vi "MC_8_21_12a_PD.vi"() -> ()   [LabVIEW 2011]
uses:
  <vilib>/Utility/file.llb/Read From Spreadsheet File (string).vi
  <vilib>/Utility/inputDevices.llb/keyboardAcquire.vi
  <vilib>/Utility/file.llb/Write To Spreadsheet File (DBL).vi
  <vilib>/Utility/file.llb/Write To Spreadsheet File (string).vi
  <vilib>/regexp/Match Regular Expression.xnode
panel:
  in  "Treatment Concentration (mM):":dbl=nan
  in  "Surface Treatment:":string="NaN"
  in  "# Drops*:":dbl=inf
  in  "Solution Temp (C):":dbl=nan
  in  "Relative Humidity (%):":dbl=nan
  in  "Room Temp (F):":dbl=nan
  in  "Time (s):":dbl=nan
  in  "RPM:":dbl=nan
  in  "Wait Time (s):":dbl=nan
  in  "Sample #:":dbl=1.0
  in  "Fabricator:":string="NaN"
  in  "Ramp (s):":dbl=3.0
  out "X Axis Display Type":string
  out "Opj X Axis":string
  in  "Room Temp":dbl=294.0
  out "No Image 2":path=path "\\\\acad1\\physics/Jurchescu-group/JW-PD/Image Not Found.png"
  out "Save1 Array":string[][](array[string])
  out "Lin Vd":dbl
  out "Lin-Vg Array-Used":dbl[](array[numeric])
  out "Lin Id-Used":dbl[](array[numeric])
  out "Rec: Comments":string
  out "Folder Index":dbl caption="Length"
  out "Current \nRecord":string[](array[string])
  out "Transformer \nHeaders":string[](array[string])
  out "Current Device ID":string
  out "Column":string
  out "Row":string
  out "Rec: Concentration":dbl
  out "Rec: Solvent":string
  out "Rec: Method":string
  in  "?":T1(tab)
  in  "Transport File":path
  out "Transport Folder":path
  out "Rec: Material":string
  out "Accel (RPM/s):":dbl
  in  "Transfer File":path
  out "Transfer Folder":path
  in  "Image Folder":path
  out "Image File":path=path "D:/UserData/Desktop/Jeremy/WFU/Research/Programs/VI mods/Image Not Found.png"
  in  "Manual Comments":bool
  in  "Comments:":string
  out "Calc: On/Off":dbl caption="On/Off-Sat" format="%#.2e"
  out "Calc: Off I-Sat":dbl caption="Off I-Sat" format="%#.2e"
  in  "Manuel-Dielectric":bool
  in  "Manuel-Length":bool
  out "Calc: VT-Lin":dbl
  out "New: VT-Lin":dbl
  out "Rec: VT-Lin":dbl caption="VT-Lin" format="%#_3g"
  out "Calc: Trap Density-STS":dbl format="%#.2e"
  out "New: Trap Density-STS":dbl format="%#.2e"
  out "Rec: Trap Density-STS":dbl caption="N-Sat (STS)" format="%#.2e"
  out "Calc: Trap Density-VT":dbl format="%#.2e"
  out "New: Trap Density-VT":dbl format="%#.2e"
  out "Rec: Trap Density-VT":dbl caption="N-Sat (VT)" format="%#.2e"
  out "Calc: Mobility-Lin":dbl format="%#.2e"
  out "New: Mobility-Lin":dbl format="%#_4e"
  out "Rec: Mobility-Lin":dbl caption="Mobility-Lin" format="%#_3e"
  out "Calc: Mobility-Sat":dbl format="%#.2e"
  out "Rec: Length":dbl caption="Length" format="%#_3g"
  out "Rec: Width":dbl caption="Width" format="%#_4g"
  out "Rec: Dielectric (d)":dbl caption="Dielectric (d)" format="%#_3g"
  in  "Cancel Button":bool
  in  "Up Button":bool
  in  "Down Button":bool
  out "Data Name:":string
  in  "Save Changes?":bool
  in  "New: Dielectric":dbl
  in  "New: Length":dbl
  in  "New: Width":dbl
  out "New: Mobility-Sat":dbl format="%#.2e"
  in  "Blank Button":bool
  in  "Zoom":i16(slide)=-3 scale=-5.0..5.0
  out "Image Out 2":T2(plugin-control)
  out "Image Out":T2(plugin-control)
  in  "Magnification":u16(ring) items=["5x", "10x", "20x", "50x", "80x"]
  out "Total Width":dbl
  out "Distances":dbl[](array[numeric])
  in  "Undo Button":bool
  in  "Remove Button":bool
  out "Rec: Mobility-Sat":dbl caption="Mobility-Sat" format="%#.2e"
  in  "Export":bool
  out "Calc: VT-Sat":dbl format="%#.2g"
  out "New: VT-Sat":dbl format="%#.2g"
  in  "Manual-Width":bool caption="Manual"
  out "Calc: STS":dbl format="%#.2g"
  out "New: STS":dbl format="%#.2g"
  out "Rec: VT-Sat":dbl caption="VT-Sat" format="%#.2g"
  out "Rec: STS":dbl caption="STS-Sat" format="%#.2g"
  out "Rec: On/Off":dbl caption="On/Off-Sat" format="%#.2e"
  in  "Save Changes? 2":bool
  in  "Save Changes? 3":bool
  out "Rec: Temp":dbl caption="Sample Temp" format="%.1f"
  in  "New: Temp":dbl format="%.1f"
  out "Rec: Off I-Sat":dbl caption="Off I-Sat" format="%#.2e"
  in  "Independant Variable":string(combo)="Length (um):"
  in  "Transfer Plots":enum32{"Linear", "Saturation"}(tab)=enum."Saturation"
  out "XY Graph-Lin":cluster{dbl[], dbl[]}[](graph)
  in  "Slide":dbl(slide) step=1.0 scale=-22.0..89.0 scale format="%#_1p"
  out "XY Graph":cluster{dbl[], dbl[]}[](graph)
  in  "Previous Button":bool
  in  "Next Button":bool
  in  "NumPts":dbl=5.0
  in  "Log Plots":enum32{"Linear", "Saturation"}(tab)=enum."Saturation"
  in  "Slide 2":dbl(slide) step=1.0 scale=-1.0..82.0 scale format="%#_1p"
  out "XY Graph 2":cluster{dbl[], dbl[]}[](graph)
  in  "Previous Button 2":bool
  in  "Next Button 2":bool
  in  "NumPts 2":dbl=5.0 caption="NumPts"
  in  "Manual-Temp":bool caption="Manual"
  out "Date Created":string caption="Fabricated"
  out "Date Recorded":string="Date Recorded" caption="Measured"
  out "Image Name":string
  out "Index":string
  in  "Origin Project File":path=path "\\\\acad1\\physics/Jurchescu-group/JW-PD/Group Library/Origin Project Files/DeviceData_8_10_12a_JW.opj"
  in  "No Image File":path=path "\\\\acad1\\physics/Jurchescu-group/JW-PD/Mega Awesome/Image Not Found.png"
  out "String":string
  out "Index 2":dbl
  out "Sat Id-Log-Used":dbl[](array[numeric])
  out "Vg Array-Log-Used":dbl[](array[numeric])
  out "ROI Descriptor out":T3 {"Contours"."Type" items=["No Selection", "Point", "Line", "Rectangle", "Oval", "Polygon", "Freehand Region", "Annulus", "Unused2", "Unused3", "Broken Line", "Freehand Line", "Rotated Rectangle"]}
  out "ROI Descriptor":T3 {"Contours"."Type" items=["No Selection", "Point", "Line", "Rectangle", "Oval", "Polygon", "Freehand Region", "Annulus", "Unused2", "Unused3", "Broken Line", "Freehand Line", "Rotated Rectangle"]}
  out "Numeric 3":dbl
  out "Array 6":dbl[][](array[numeric])
  out "Cluster":T4
  out "Array 5":dbl[](array[numeric])
  out "Array 4":dbl[](array[numeric])
  out "Array 3":dbl[](array[numeric])
  out "Numeric 2":dbl
  out "Numeric":dbl
  out "Sat Id-Used":dbl[](array[numeric])
  out "Sat Vg Array-Used":dbl[](array[numeric])
  out "MobVi Index":dbl
  in  "Row Start":dbl=20.0
  # "Sample Properties"
  # "*     Inf = Full coverage\n   NaN = Unknown or Not Applicable"
  # "Data Locations"
  # "Transport Location"
  # "Transfer Location"
  # "Image Location"
  # "Recorded"
  # "Calculated"
  # "Re-Calculated"
  # "Manual"
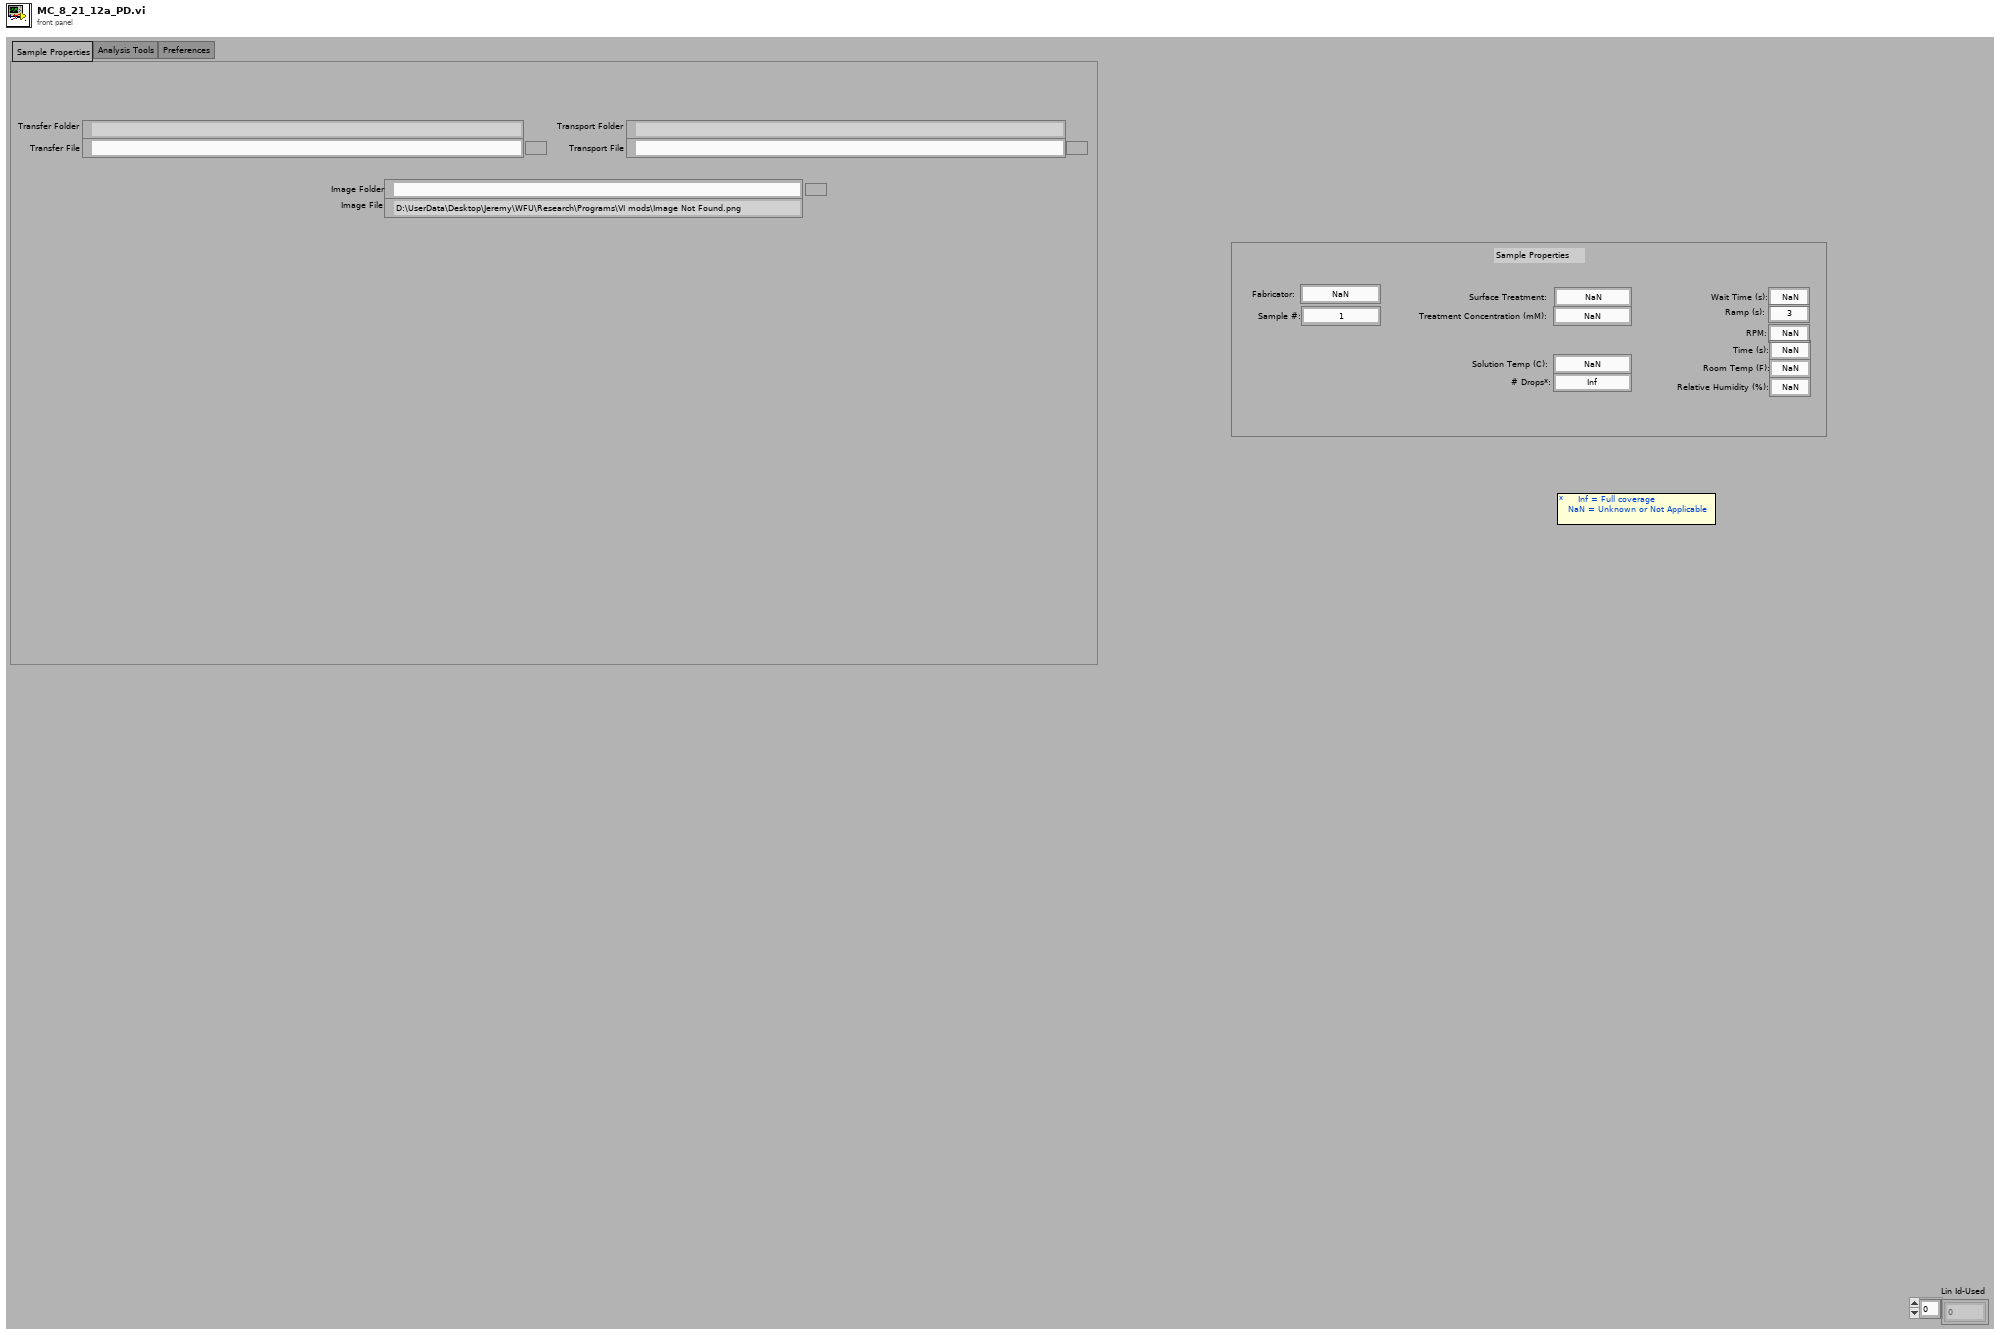
[diagram p1: front panel]
types:
  T1 = enum32{"Sample Properties", "Analysis Tools", "Preferences", "Current Database"}
  T2 = typedef "IMAQ Image.ctl" = refnum<image>
  T3 = typedef "ROI Descriptor" = cluster{"Global Rectangle":i32[], "Contours":cluster{"ID":enum32{"External", "Internal"}, "Type":u32, "Coordinates":i32[]}[]}
  T4 = cluster{"Numeric":dbl, "Numeric 2":dbl, "Numeric 3":dbl, "Numeric 4":dbl}
  T5 = cluster{"Mobility-Sat":dbl, "Moblitity-Lin":dbl, "On/Off":dbl, "Off Current":dbl, "Vt-Sat":dbl, "STS":dbl, "Trap Density-VT":dbl, "Trap Density-STS":dbl}
  T6 = cluster{"Date Recorded":string, "Index":string, "Length":dbl, "Width":dbl, "Sample Temp":dbl}
  T7 = cluster{"Date Created":string, "Material":string, "Solvent":string, "Concentration":dbl, "Method":string, "Dielectric (nm)":dbl, "Treatment":string, "Comments":string}
  T8 = cluster{"Mobility-Sat":dbl, "Vt-Sat":dbl, "Mobility-Lin":dbl, "Vt-Lin":dbl, "Off I-Sat":dbl, "On/Off I-Sat":dbl}
  T9 = cluster{"[0]":cluster{dbl[], dbl[]}, "[1]":cluster{dbl[], dbl[]}, "[2]":cluster{dbl[], dbl[]}, "[3]":cluster{dbl[], dbl[]}, "[4]":cluster{dbl[], dbl[]}, "[5]":cluster{dbl[], dbl[]}, "[6]":cluster{dbl[], dbl[]}, "[7]":cluster{dbl[], dbl[]}, "[8]":cluster{dbl[], dbl[]}}
  T10 = cluster{"Global Rectangle":i32[], "Contours":cluster{"Contour Type":u32, "ROI Type":u32, "Points":i32[]}[]}
  T11 = typedef "LVBoundsTypeDef.ctl" = cluster{"Width":u32, "Height":u32}
  T12 = enum16{"0", "1", "2", "3", "4", "5", "6", "7", "8", "9", "A", "B", "C", "D", "E", "F", "G", "H", "I", "J", "K", "L", "M", "N", "O", "P", "Q", "R", "S", "T", "U", "V", "W", "X", "Y", "Z", "F1", "F2", "F3", "F4", "F5", "F6", "F7", "F8", "F9", "F10", "F11", "F12", "F13", "F14", "F15", "ADD", "BACK", "BACKSLASH", "CAPITAL", "COMMA", "DECIMAL", "DELETE", "DIVIDE", "DOWN", "END", "EQUALS", "ESCAPE", "GRAVE (`)", "HOME", "INSERT", "LBRACKET", "LCONTROL", "LEFT", "L ALT", "LSHIFT", "LWIN", "MINUS", "MULTIPLY", "NEXT", "NUMLOCK", "NUMPAD_0", "NUMPAD_1", "NUMPAD_2", "NUMPAD_3", "NUMPAD_4", "NUMPAD_5", "NUMPAD_6", "NUMPAD_7", "NUMPAD_8", "NUMPAD_9", "PAUSE", "PERIOD", "PRIOR (PG UP)", "RBRACKET", "RCONTROL", "RETURN", "RIGHT", "R ALT", "RSHIFT", "RWIN", "SCROLL", "SEMICOLON", "SLASH", "SPACE", "SUBTRACT", "TAB", "UP", "ENTER (num pad)", "' (quote)"}[]
  T13 = enum16{"0", "1", "2", "3", "4", "5", "6", "7", "8", "9", "A", "B", "C", "D", "E", "F", "G", "H", "I", "J", "K", "L", "M", "N", "O", "P", "Q", "R", "S", "T", "U", "V", "W", "X", "Y", "Z", "F1", "F2", "F3", "F4", "F5", "F6", "F7", "F8", "F9", "F10", "F11", "F12", "F13", "F14", "F15", "ADD", "BACK", "BACKSLASH", "CAPITAL", "COMMA", "DECIMAL", "DELETE", "DIVIDE", "DOWN", "END", "EQUALS", "ESCAPE", "GRAVE (`)", "HOME", "INSERT", "LBRACKET", "LCONTROL", "LEFT", "L ALT", "LSHIFT", "LWIN", "MINUS", "MULTIPLY", "NEXT", "NUMLOCK", "NUMPAD_0", "NUMPAD_1", "NUMPAD_2", "NUMPAD_3", "NUMPAD_4", "NUMPAD_5", "NUMPAD_6", "NUMPAD_7", "NUMPAD_8", "NUMPAD_9", "PAUSE", "PERIOD", "PRIOR (PG UP)", "RBRACKET", "RCONTROL", "RETURN", "RIGHT", "R ALT", "RSHIFT", "RWIN", "SCROLL", "SEMICOLON", "SLASH", "SPACE", "SUBTRACT", "TAB", "UP", "ENTER (num pad)", "' (quote)"}
  T14 = cluster{"Contour Type":u32, "ROI Type":u32, "Points":i32[]}[]
  T15 = cluster{i32[], cluster{"Contour Type":u32, "ROI Type":u32, "Points":i32[]}[]}
  T16 = cluster{"Independant  Variable Indicator":string, "Parameter String Indicator":string}
  T17 = cluster{string, sgl, bool, bool, bool, bool, bool, bool, i32}
  T18 = cluster{i32, cluster{string, sgl, bool, bool, bool, bool, bool, bool, i32}, i32, i32}
  T19 = cluster{"Contour Type":u32, "ROI Type":u32, "Points":i32[]}
  T20 = cluster{"Points[0]":i32, "Points[1]":i32, "Points[2]":i32, "Points[3]":i32, "Points[4]":i32, "Points[5]":i32, "Points[6]":i32, "Points[7]":i32, "Points[8]":i32}
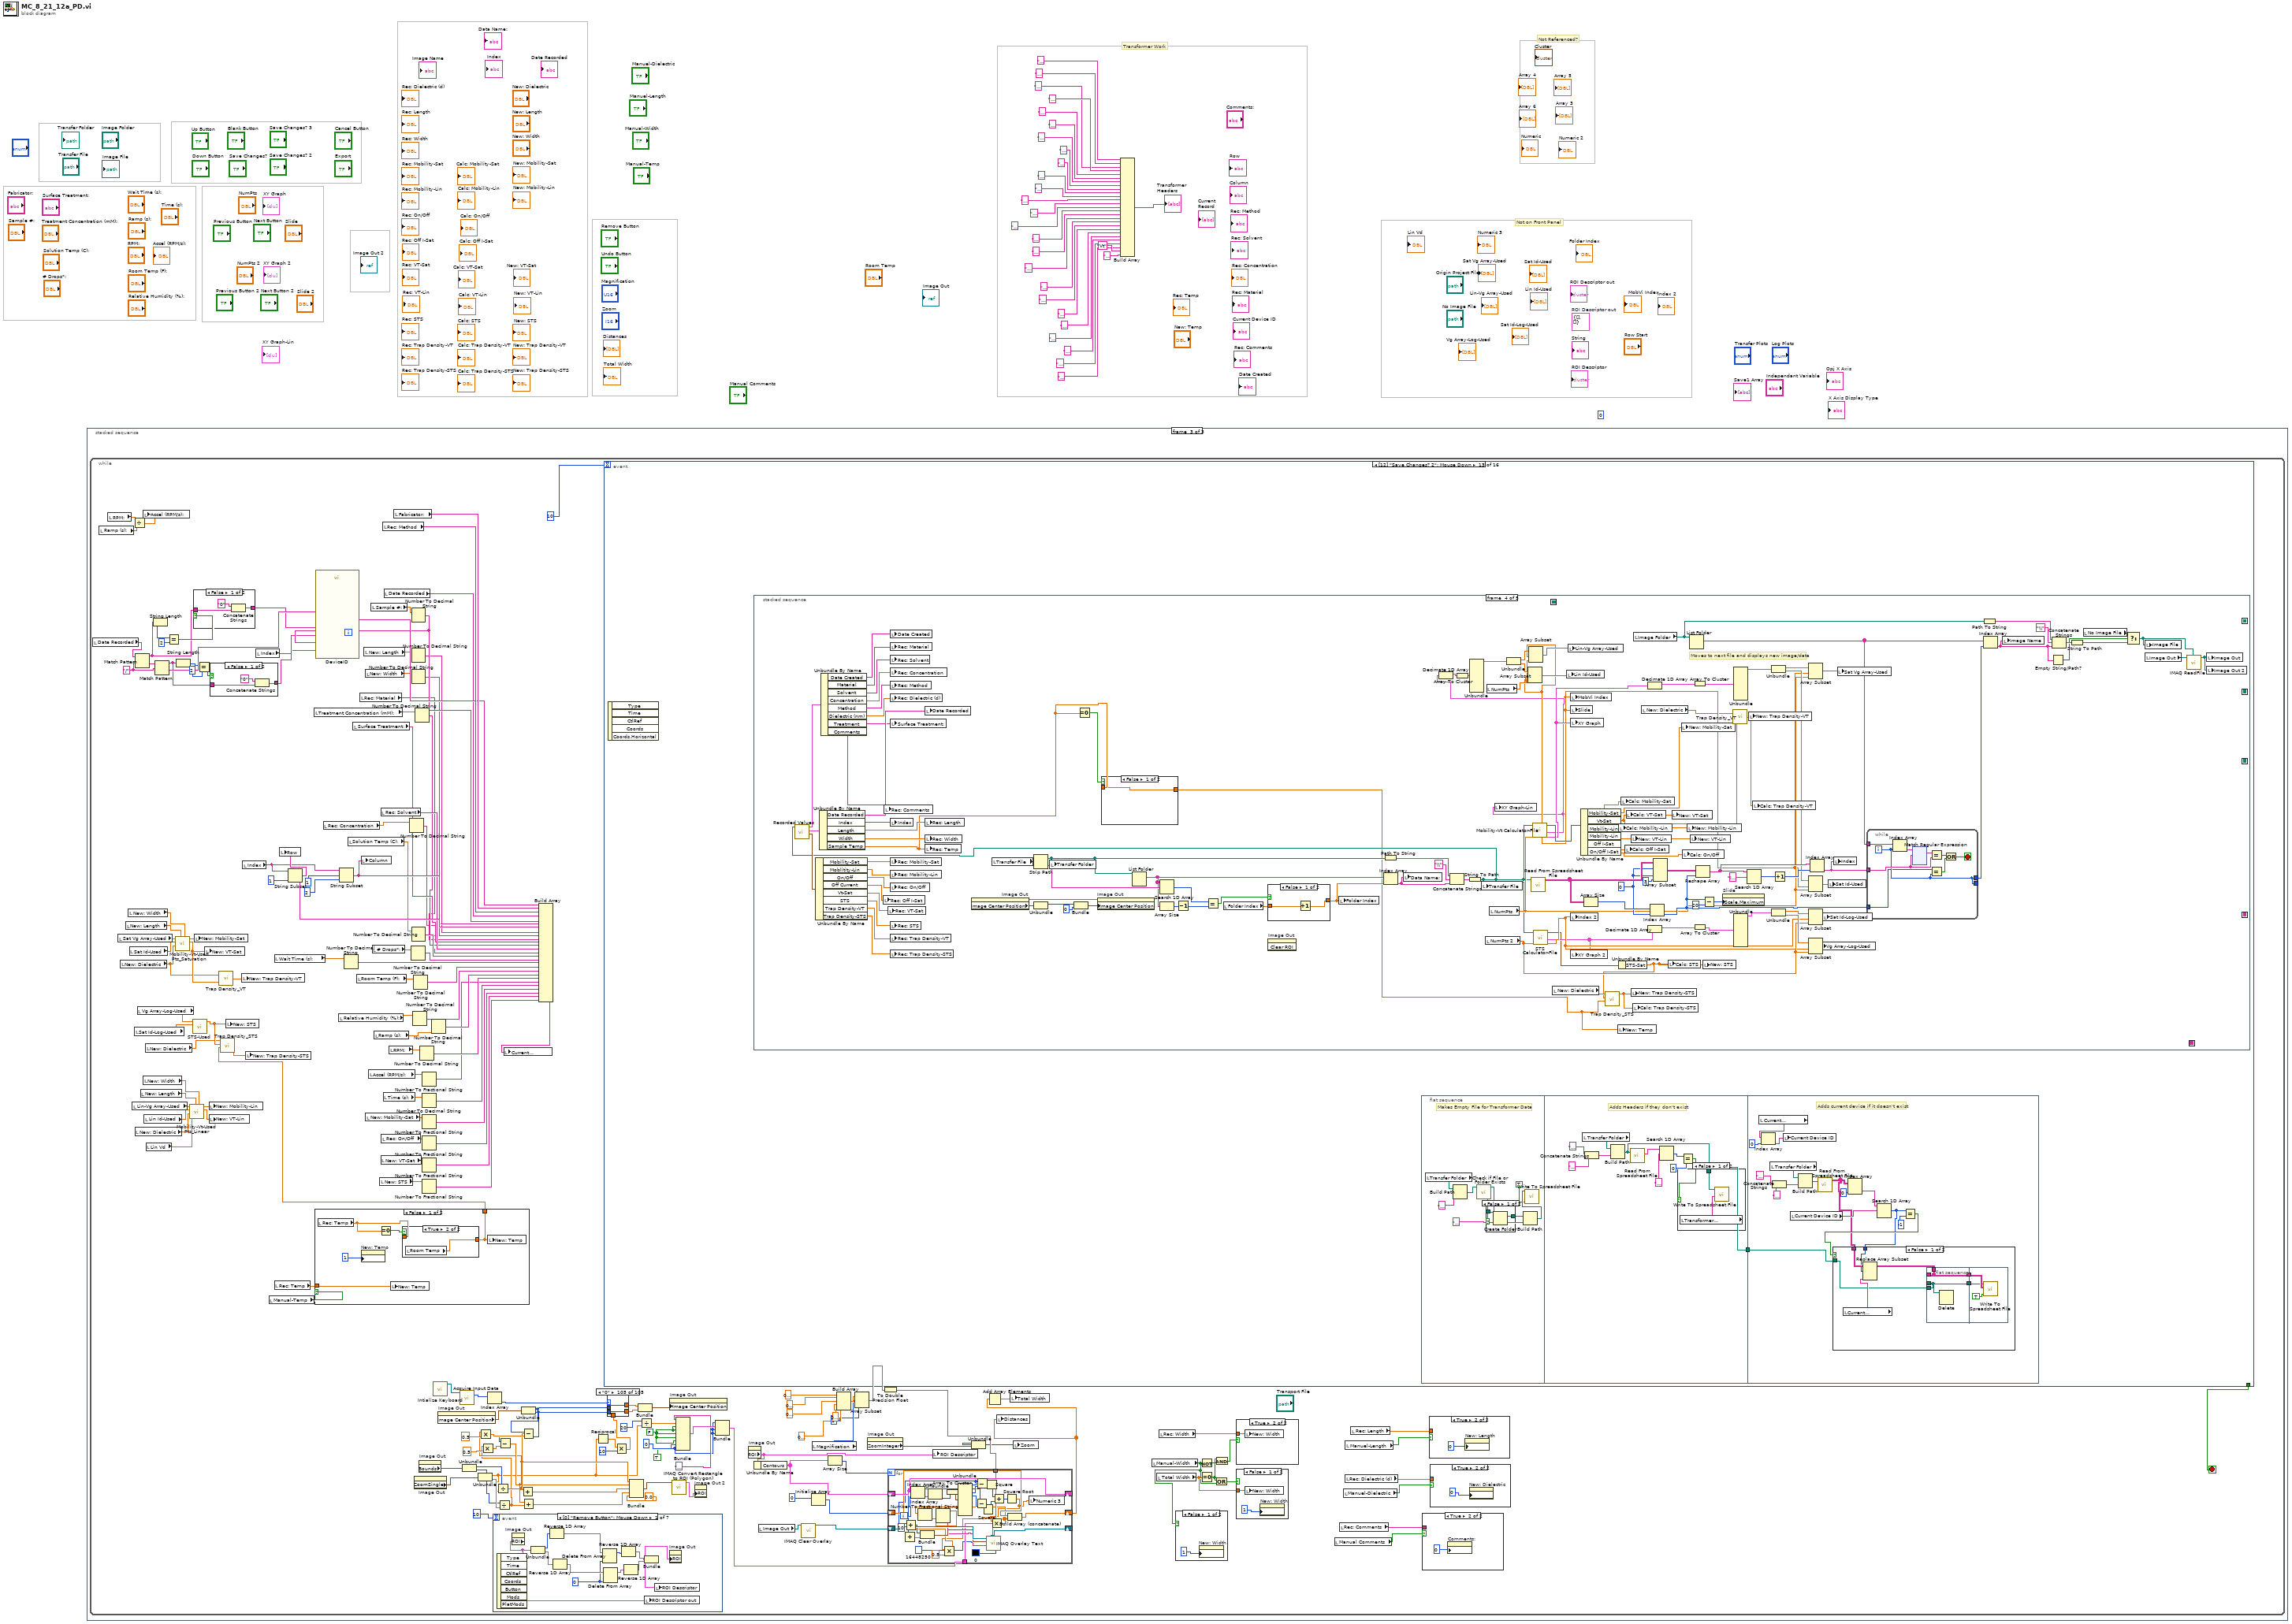
[diagram p0: block diagram]
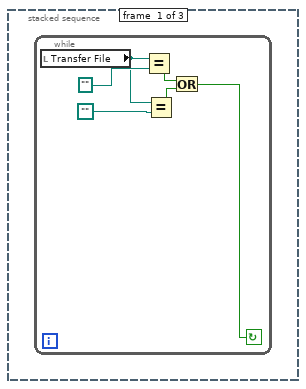
[diagram p2: hidden frame]
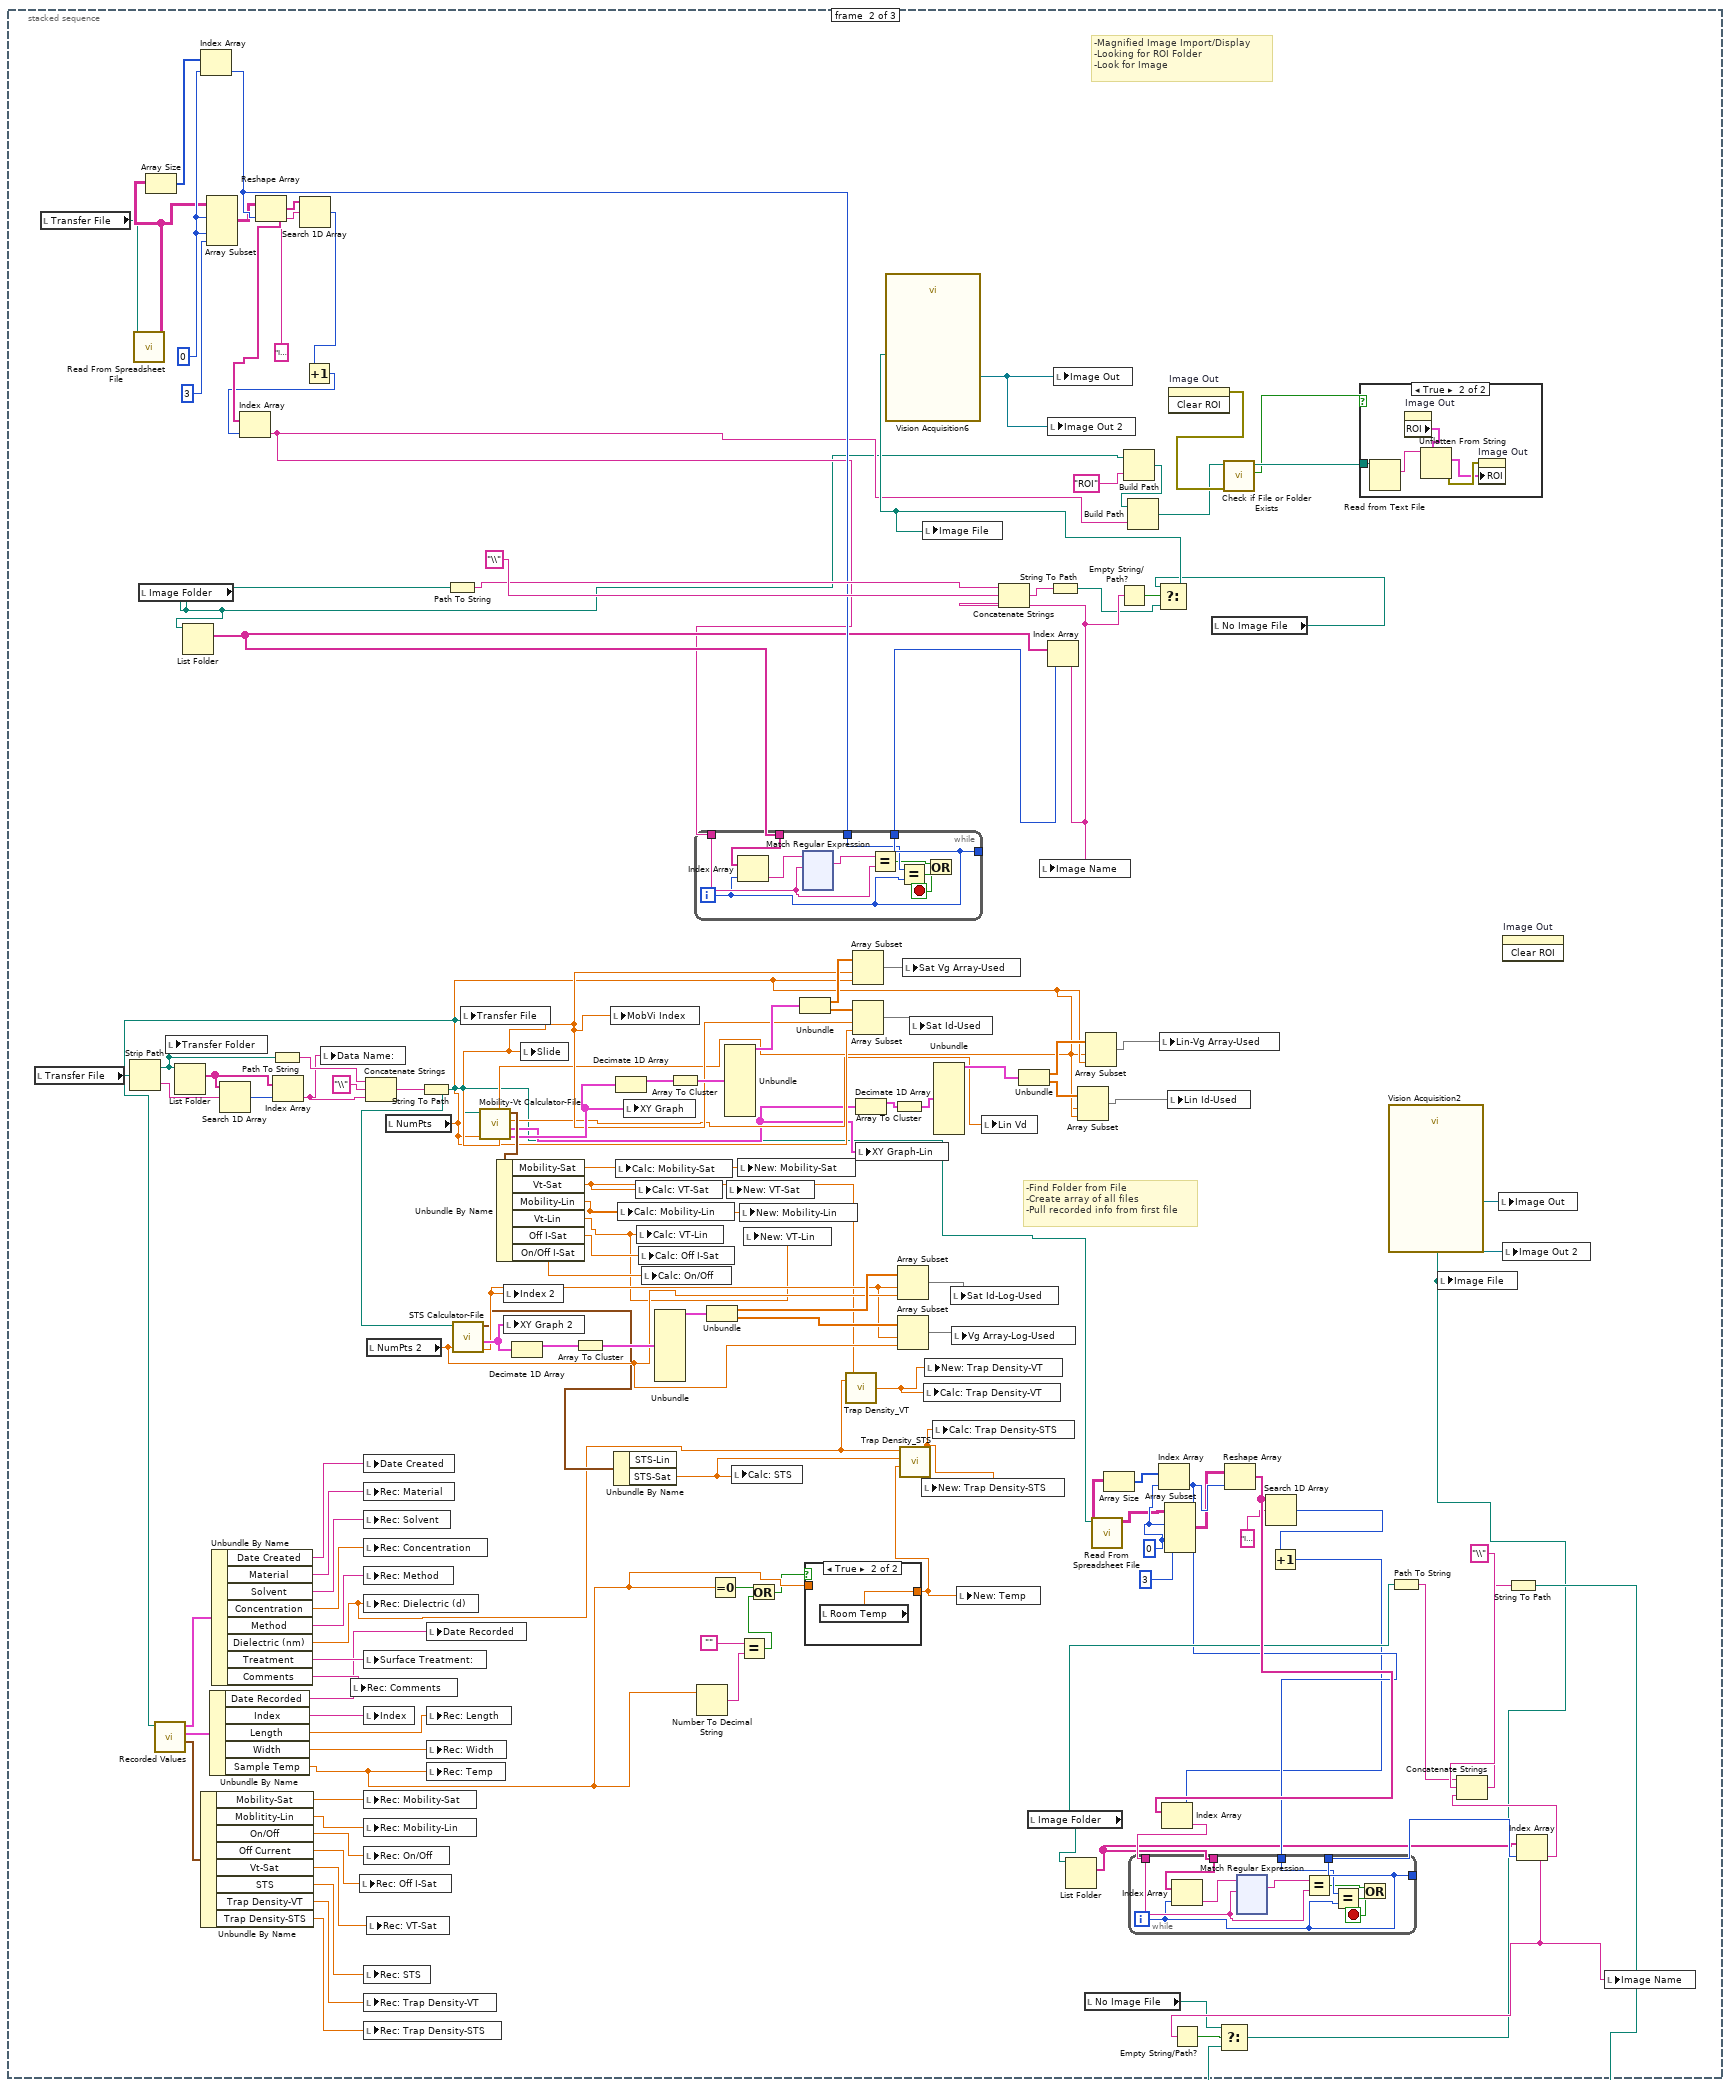
[diagram p3: hidden frame]
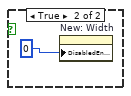
[diagram p6: hidden frame]
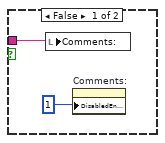
[diagram p7: hidden frame]
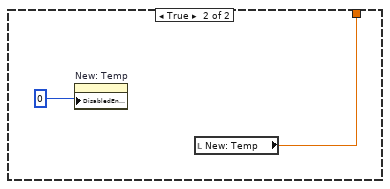
[diagram p9: hidden frame]
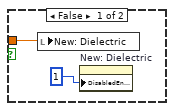
[diagram p10: hidden frame]
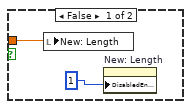
[diagram p11: hidden frame]
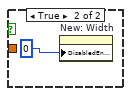
[diagram p15: hidden frame]
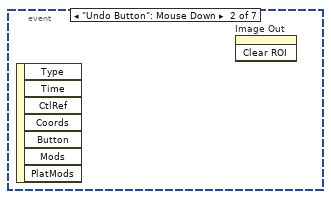
[diagram p16: hidden frame]
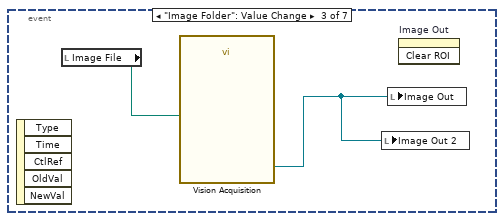
[diagram p17: hidden frame]
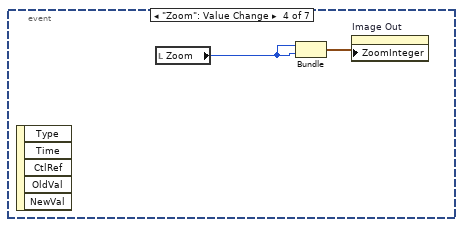
[diagram p18: hidden frame]
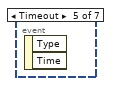
[diagram p19: hidden frame]
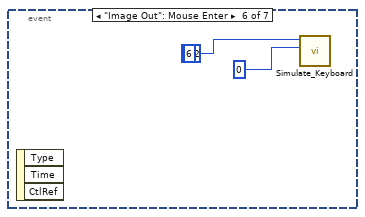
[diagram p20: hidden frame]
diagram:
  (unwired) 0
  (unwired) T3 {"Global Rectangle"=[], "Contours"=[]}  # ROI Descriptor out
  # "Not Referenced?"
  # "Transformer Work"
  # "Not on Front Panel"
  n1 = stacked-sequence {
    frame #0 {
      n2 = while {
        stop <- w29 continue-if-true
        n3 = local read "Transfer File"() -> (w31:path)
        n4 = Equal?(x=w31, y=path "") -> (x = y?=w33:bool)
        n5 = Equal?(x=w31, y=path "") -> (x = y?=w32:bool)
        n6 = Or(x=w33, y=w32) -> (x .or. y?=w29:bool)
      }
    }
    frame #1 {
      w133 = 0
      w157 = 0
      # "-Find Folder from File\n-Create array of all files\n-Pull recorded info from first file"
      # "-Magnified Image Import/Display\n-Looking for ROI Folder\n-Look for Image"
      n7 = local read "Transfer File"() -> (w137:path)
      n8 = local read "Transfer File"() -> (w152:path)
      n9 = Strip Path(path=w137) -> (stripped path=w138:path, name=w124:string)
      n10 = call-poly <vilib>:"Read From Spreadsheet File.vi"("file path (dialog if empty)"=w152) -> ("all rows"=w155:string[][])  [unwired: 6 in, 4 out]
      n11 = local read "Image Folder"() -> (w94:path)
      n12 = Array Size(array=w155) -> (size(s)=w156:i32[])
      n13 = local write "Transfer Folder"(w138) -> ()
      n14 = List Folder(path=w138) -> (filenames=w128:string[])  [unwired: 3 in, 3 out]
      n15 = List Folder(path=w94) -> (filenames=w161:string[])  [unwired: 3 in, 3 out]
      n16 = Index Array(array=w156, index=w157) -> (element=w163:i32)
      n17 = Array Subset(array=w155, index (row)=w157, index (col)=w157, length (col)=3) -> (w154:string[][])  [unwired: 1 in]
      n18 = Search 1D Array(1D array=w128, element=w124) -> (index of element=w127:i32)  [unwired: 1 in]
      n19 = Reshape Array(w154, w163) -> (w168:string[])
      n20 = Path To String(path=w138) -> (string=w123:string)
      n21 = Index Array(array=w128, index=w127) -> (element=w93:string)
      n22 = Search 1D Array(1D array=w168, element="Index:") -> (index of element=w160:i32)  [unwired: 1 in]
      n23 = Increment(x=w160) -> (x+1=w159:i32)
      n24 = Index Array(array=w168, index=w159) -> (element=w95:string)
      n25 = local write "Data Name:"(w93) -> ()
      n26 = Concatenate Strings(w123, "\\", w93) -> (w125:string)
      n27 = local read "NumPts 2"() -> (w68:dbl)
      n28 = local read "NumPts"() -> (w59:dbl)
      n29 = String To Path(string=w125) -> (path=w52:path)
      n30 = call "Recorded Values.vi"("Path"=w52) -> ("Recorded Char"=w91:T5, "Recorded Prop"=w90:T6, "Fabrication Prop"=w92:T7)  [unwired: 8 in]
      n31 = Unbundle By Name(w91) -> ("Mobility-Sat"=w79:dbl, "Moblitity-Lin"=w78:dbl, "On/Off"=w77:dbl, "Off Current"=w76:dbl, "Vt-Sat"=w38:dbl, "STS"=w75:dbl, "Trap Density-VT"=w74:dbl, "Trap Density-STS"=w73:dbl)
      n32 = Unbundle By Name(w90) -> ("Date Recorded"=w83:string, "Index"=w82:string, "Length"=w81:dbl, "Width"=w80:dbl, "Sample Temp"=w44:dbl)
      n33 = Unbundle By Name(w92) -> ("Date Created"=w72:string, "Material"=w89:string, "Solvent"=w88:string, "Concentration"=w87:dbl, "Method"=w86:string, "Dielectric (nm)"=w48:dbl, "Treatment"=w85:string, "Comments"=w84:string)
      n34 = local write "Rec: Comments"(w84) -> ()
      n35 = local write "Rec: Off I-Sat"(w76) -> ()
      n36 = local write "Date Created"(w72) -> ()
      n37 = local write "Rec: Material"(w89) -> ()
      n38 = local write "Rec: Solvent"(w88) -> ()
      n39 = local write "Rec: Concentration"(w87) -> ()
      n40 = local write "Rec: Method"(w86) -> ()
      n41 = local write "Rec: Dielectric (d)"(w48) -> ()
      n42 = local write "Surface Treatment:"(w85) -> ()
      n43 = local write "Index"(w82) -> ()
      n44 = local write "Rec: Mobility-Sat"(w79) -> ()
      n45 = local write "Rec: Mobility-Lin"(w78) -> ()
      n46 = local write "Rec: On/Off"(w77) -> ()
      n47 = local write "Rec: STS"(w75) -> ()
      n48 = local write "Rec: Trap Density-VT"(w74) -> ()
      n49 = local write "Rec: Trap Density-STS"(w73) -> ()
      n50 = local write "Rec: VT-Sat"(w38) -> ()
      n51 = local write "Date Recorded"(w83) -> ()
      n52 = local write "Rec: Length"(w81) -> ()
      n53 = local write "Rec: Width"(w80) -> ()
      n54 = local write "Rec: Temp"(w44) -> ()
      n55 = Path To String(path=w94) -> (string=w165:string)
      n56 = call "STS Calculator-File.vi"("NumPts"=w68, "Path"=w52) -> ("STS Index-Sat"=w66:dbl, "XY Graph-Sat"=w67:cluster{dbl[], dbl[]}[], "Ouput"=w65:cluster{"STS-Sat":dbl, "STS-Lin":dbl})  [unwired: 5 in, 2 out]
      n57 = local write "Transfer File"(w52) -> ()
      n58 = call "Mobility-Vt Calculator-File.vi"("NumPts"=w59, "Path"=w52) -> ("XY Graph-Sat"=w70:cluster{dbl[], dbl[]}[], "XY Graph-Lin"=w54:cluster{dbl[], dbl[]}[], "Lin Vd"=w55:dbl, "Output"=w71:T8, "Index-Sat"=w69:dbl, "Index-Lin"=w58:dbl)  [unwired: 4 in]
      n59 = Unbundle By Name(w71) -> ("Mobility-Sat"=w47:dbl, "Vt-Sat"=w46:dbl, "Mobility-Lin"=w37:dbl, "Vt-Lin"=w35:dbl, "Off I-Sat"=w53:dbl, "On/Off I-Sat"=w36:dbl)
      n60 = local write "Index 2"(w66) -> ()
      n61 = local write "XY Graph 2"(w67) -> ()
      n62 = Decimate 1D Array(w67) -> (w115:cluster{dbl[], dbl[]}[])  [unwired: 1 out]
      n63 = local write "Slide"(w69) -> ()
      n64 = Array To Cluster(array=w115) -> (cluster=w117:T9)
      n65 = local write "MobVi Index"(w69) -> ()
      n66 = Unbundle By Name(w65) -> ("STS-Sat"=w51:dbl)  [unwired: 1 out]
      n67 = Decimate 1D Array(w70) -> (w151:cluster{dbl[], dbl[]}[])  [unwired: 1 out]
      n68 = local write "Calc: Mobility-Sat"(w47) -> ()
      n69 = local write "Calc: Mobility-Lin"(w37) -> ()
      n70 = local write "XY Graph"(w70) -> ()
      n71 = local write "Calc: VT-Sat"(w46) -> ()
      n72 = local write "Calc: VT-Lin"(w35) -> ()
      n73 = local write "Calc: Off I-Sat"(w53) -> ()
      n74 = local write "Calc: On/Off"(w36) -> ()
      n75 = Unbundle(w117) -> ("[0]"=w116:cluster{dbl[], dbl[]})  [unwired: 8 out]
      n76 = Array To Cluster(array=w151) -> (cluster=w149:T9)
      n77 = while {
        tunnel: w161 -> [w303]
        tunnel: w95 -> [w301]
        tunnel: [w300] -> _
        tunnel: [w300] -> w162
        tunnel: w163 -> [w299]
        i -> [w300]
        stop <- w296 stop-if-true
        n78 = Index Array(array=w303, index=w300) -> (element=w304:string)
        n79 = xnode "Match Regular Expression"("input string"=w304, "regular expression"=w301) -> ("whole match"=w302:string)  [unwired: 4 in, 4 out]
        n80 = Equal?(x=w302, y=w301) -> (x = y?=w298:bool)
        n81 = Equal?(x=w299, y=w300) -> (x = y?=w297:bool)
        n82 = Or(x=w298, y=w297) -> (x .or. y?=w296:bool)
      }
      n83 = Number To Decimal String(number=w44) -> (decimal integer string=w42:string)  [unwired: 1 in]
      n84 = Unbundle(w116) -> (w113:dbl[], w112:dbl[])
      n85 = Equal To 0?(x=w44) -> (x = 0?=w43:bool)
      n86 = Unbundle(w149) -> ("[0]"=w150:cluster{dbl[], dbl[]})  [unwired: 8 out]
      n87 = local write "New: VT-Sat"(w46) -> ()
      n88 = local write "Calc: STS"(w51) -> ()
      n89 = local write "New: Mobility-Sat"(w47) -> ()
      n90 = Equal?(x="", y=w42) -> (x = y?=w40:bool)
      n91 = local write "New: Mobility-Lin"(w37) -> ()
      n92 = local write "New: VT-Lin"(w35) -> ()
      n93 = Or(x=w43, y=w40) -> (x .or. y?=w39:bool)
      n94 = Unbundle(w150) -> (w114:dbl[], w118:dbl[])
      n95 = case shown="True" w39 {
        tunnel: [w169 w170] -> w50
        tunnel: w44 -> [w169 _]
        frame False {
        }
        frame True {
          n96 = local read "Room Temp"() -> (w170:dbl)
        }
      }
      n97 = call "Trap Density_VT.vi"("VT"=w46, "Dielectric"=w48) -> ("Trap Density-VT"=w45:dbl)
      n98 = Array Subset(array=w114, index=w69, length=w59) -> (w121:dbl[])
      n99 = Array Subset(array=w118, index=w69, length=w59) -> (w122:dbl[])
      n100 = Decimate 1D Array(w54) -> (w64:cluster{dbl[], dbl[]}[])  [unwired: 1 out]
      n101 = local write "XY Graph-Lin"(w54) -> ()
      n102 = Array To Cluster(array=w64) -> (cluster=w63:T9)
      n103 = Array Subset(array=w113, index=w66, length=w68) -> (w120:dbl[])
      n104 = Array Subset(array=w112, index=w66, length=w68) -> (w119:dbl[])
      n105 = call "Trap Density_STS.vi"("Temp (T) [K]"=w50, "S.T.S. (S)"=w51, "Dielectric"=w48) -> ("Trap Density (N)"=w49:dbl)  [unwired: 8 in]
      n106 = local write "Sat Vg Array-Used"(w121) -> ()
      n107 = local write "Sat Id-Used"(w122) -> ()
      n108 = local write "New: Trap Density-STS"(w49) -> ()
      n109 = local write "Calc: Trap Density-VT"(w45) -> ()
      n110 = local write "New: Trap Density-VT"(w45) -> ()
      n111 = local write "Calc: Trap Density-STS"(w49) -> ()
      n112 = Unbundle(w63) -> ("[0]"=w62:cluster{dbl[], dbl[]})  [unwired: 8 out]
      n113 = local write "Sat Id-Log-Used"(w120) -> ()
      n114 = local write "Vg Array-Log-Used"(w119) -> ()
      n115 = local write "New: Temp"(w50) -> ()
      n116 = local write "Lin Vd"(w55) -> ()
      n117 = Unbundle(w62) -> (w61:dbl[], w60:dbl[])
      n118 = local read "Image Folder"() -> (w144:path)
      n119 = Index Array(array=w161, index=w162) -> (element=w111:string)
      n120 = Concatenate Strings(w165, "\\", w111) -> (w166:string)
      n121 = local write "Image Name"(w111) -> ()
      n122 = String To Path(string=w166) -> (path=w109:path)
      n123 = List Folder(path=w144) -> (filenames=w140:string[])  [unwired: 3 in, 3 out]
      n124 = Array Subset(array=w60, index=w58, length=w59) -> (w56:dbl[])
      n125 = local read "No Image File"() -> (w103:path)
      n126 = Array Subset(array=w61, index=w58, length=w59) -> (w57:dbl[])
      n127 = call-poly <vilib>:"Read From Spreadsheet File.vi"("file path (dialog if empty)"=w52) -> ("all rows"=w131:string[][])  [unwired: 6 in, 4 out]
      n128 = Array Size(array=w131) -> (size(s)=w132:i32[])
      n129 = Empty String/Path?(string/path=w111) -> (empty?=w110:bool)
      n130 = Build Path(base path=w94, name or relative path="ROI") -> (appended path=w97:path)
      n131 = Build Path(base path=w97, name or relative path=w95) -> (appended path=w96:path)
      n132 = Index Array(array=w132, index=w133) -> (element=w143:i32)
      n133 = local write "Lin-Vg Array-Used"(w57) -> ()
      n134 = Array Subset(array=w131, index (row)=w133, index (col)=w133, length (col)=3) -> (w130:string[][])  [unwired: 1 in]
      n135 = local write "Lin Id-Used"(w56) -> ()
      n136 = invoke on="Image Out" class="ImageControl" method="Clear ROI"() -> (error out=w101:errorcluster)  [unwired: 3 in, 2 out]
      n137 = local read "No Image File"() -> (w102:path)
      n138 = Select(t=w102, s=w110, f=w109) -> (s? t:f=w108:path)
      n139 = call "Vision Acquisition6"("Image Path"=w108) -> ("Image Out"=w164:T2)  [unwired: 25 in, 1 out]
      n140 = local write "Image File"(w108) -> ()
      n141 = local write "Image Out 2"(w164) -> ()
      n142 = local write "Image Out"(w164) -> ()
      n143 = call <vilib>:"Check if File or Folder Exists.vi"("error in (no error)"=w101, "path"=w96) -> ("file or folder exists?"=w99:bool, "dup path"=w100:path)  [unwired: 7 in, 1 out]
      n144 = Reshape Array(w130, w143) -> (w148:string[])
      n145 = Search 1D Array(1D array=w148, element="Index:") -> (index of element=w136:i32)  [unwired: 1 in]
      n146 = Increment(x=w136) -> (x+1=w135:i32)
      n147 = Index Array(array=w148, index=w135) -> (element=w141:string)
      n148 = while {
        tunnel: w140 -> [w183]
        tunnel: w141 -> [w181]
        tunnel: [w180] -> _
        tunnel: [w180] -> w142
        tunnel: w143 -> [w179]
        i -> [w180]
        stop <- w176 stop-if-true
        n149 = Index Array(array=w183, index=w180) -> (element=w184:string)
        n150 = xnode "Match Regular Expression"("input string"=w184, "regular expression"=w181) -> ("whole match"=w182:string)  [unwired: 4 in, 4 out]
        n151 = Equal?(x=w182, y=w181) -> (x = y?=w178:bool)
        n152 = Equal?(x=w179, y=w180) -> (x = y?=w177:bool)
        n153 = Or(x=w178, y=w177) -> (x .or. y?=w176:bool)
      }
      n154 = case shown="True" w99 {
        tunnel: w100 -> [_ w171]
        frame False {
        }
        frame True {
          n155 = Read from Text File(file (use dialog)=w171) -> (text=w175:string)  [unwired: 3 in, 3 out]
          n156 = property on="Image Out" class="ImageControl"() -> ("ROI"=w172:T10)  [unwired: 2 in, 2 out]
          n157 = Unflatten From String(type=w172, binary string=w175) -> (value=w173:T10, error out=w174:errorcluster)  [unwired: 3 in, 1 out]
          n158 = property on="Image Out" class="ImageControl"(error in=w174, "ROI"=w173) -> ()  [unwired: 1 in, 2 out]
        }
      }
      n159 = Path To String(path=w144) -> (string=w145:string)
      n160 = invoke on="Image Out" class="ImageControl" method="Clear ROI"() -> ()  [unwired: 3 in, 3 out]
      n161 = Index Array(array=w140, index=w142) -> (element=w106:string)
      n162 = Empty String/Path?(string/path=w106) -> (empty?=w107:bool)
      n163 = Concatenate Strings(w145, "\\", w106) -> (w146:string)
      n164 = String To Path(string=w146) -> (path=w105:path)
      n165 = Select(t=w103, s=w107, f=w105) -> (s? t:f=w104:path)
      n166 = call "Vision Acquisition2"("Image Path"=w104) -> ("Image Out"=w139:T2)  [unwired: 25 in, 1 out]
      n167 = local write "Image File"(w104) -> ()
      n168 = local write "Image Out"(w139) -> ()
      n169 = local write "Image Out 2"(w139) -> ()
      n170 = local write "Image Name"(w106) -> ()
    }
    frame #2 {
      n171 = while {
        stop <- w583 stop-if-true
        w480 = "/"
        w533 = FALSE
        w531 = 0
        n172 = local read "Date Recorded"() -> (w483:string)
        n173 = local read "Ramp (s):"() -> (w450:dbl)
        n174 = local read "RPM:"() -> (w451:dbl)
        n175 = local read "Sat Vg Array-Used"() -> (w439:dbl[])
        n176 = local read "New: Dielectric"() -> (w424:dbl)
        n177 = local read "New: Length"() -> (w440:dbl)
        n178 = local read "New: Width"() -> (w442:dbl)
        n179 = local read "Sat Id-Used"() -> (w438:dbl[])
        n180 = local read "Lin-Vg Array-Used"() -> (w433:dbl[])
        n181 = Divide(x=w451, y=w450) -> (x/y=w449:dbl)
        n182 = local read "Sat Id-Log-Used"() -> (w437:dbl[])
        n183 = local read "New: Dielectric"() -> (w430:dbl)
        n184 = Match Pattern(string=w483, regular expression=w480) -> (before substring=w474:string, after substring=w481:string)  [unwired: 1 in, 2 out]
        n185 = local read "Vg Array-Log-Used"() -> (w436:dbl[])
        n186 = local read "New: Length"() -> (w432:dbl)
        n187 = local write "Accel (RPM/s):"(w449) -> ()
        n188 = local read "New: Width"() -> (w429:dbl)
        n189 = local read "Lin Id-Used"() -> (w434:dbl[])
        n190 = local read "New: Dielectric"() -> (w426:dbl)
        n191 = local read "Lin Vd"() -> (w428:dbl)
        n192 = String Length(string=w474) -> (length=w477:i32)
        n193 = Match Pattern(string=w481, regular expression=w480) -> (before substring=w468:string, after substring=w479:string)  [unwired: 1 in, 2 out]
        n194 = Equal?(x=w477, y=2) -> (x = y?=w475:bool)
        n195 = call "Mobility-Vt-Used Pts_Saturation.vi"("Width"=w442, "Length"=w440, "Dielectric (d)"=w424, "Sat Id Used"=w438, "Vg Used"=w439) -> ("Vt"=w425:dbl, "Mobility"=w441:dbl)  [unwired: 4 in, 1 out]
        n196 = String Length(string=w468) -> (length=w470:i32)
        n197 = call "Mobility-Vt-Used Pts_Linear.vi"("Width"=w429, "Length"=w432, "Vd"=w428, "Dielectric (d)"=w430, "Sat Id Used"=w434, "Vg Used"=w433) -> ("Vt"=w435:dbl, "Mobility"=w431:dbl)  [unwired: 3 in, 1 out]
        n198 = call "STS-Used.vi"("Id Used"=w437, "Vg-Used"=w436) -> ("STS"=w427:dbl)  [unwired: 9 in]
        n199 = case shown="False" w475 {
          tunnel: w474 -> [w609 w611]
          tunnel: [w608 w611] -> w473
          frame False {
            n200 = Concatenate Strings("0", w609) -> (w608:string)
          }
          frame True {
          }
        }
        n201 = local write "New: Mobility-Sat"(w441) -> ()
        n202 = Equal?(x=w470, y=2) -> (x = y?=w472:bool)
        n203 = local write "New: VT-Sat"(w425) -> ()
        n204 = local write "New: Mobility-Lin"(w431) -> ()
        n205 = local write "New: VT-Lin"(w435) -> ()
        n206 = case shown="False" w472 {
          tunnel: w468 -> [w605 w607]
          tunnel: [w604 w607] -> w469
          frame False {
            n207 = Concatenate Strings("0", w605) -> (w604:string)
          }
          frame True {
          }
        }
        n208 = call "Trap Density_VT.vi"("VT"=w425, "Dielectric"=w424) -> ("Trap Density-VT"=w423:dbl)
        n209 = local write "New: STS"(w427) -> ()
        n210 = local write "New: Trap Density-VT"(w423) -> ()
        n211 = local read "Index"() -> (w453:string)
        n212 = local read "Index"() -> (w467:string)
        n213 = local read "Manual-Temp"() -> (w420:bool)
        n214 = local read "Wait Time (s):"() -> (w513:dbl)
        n215 = local read "Rec: Temp"() -> (w421:dbl)
        n216 = String Subset(string=w453, length (rest)=1) -> (substring=w508:string)  [unwired: 1 in]
        n217 = local write "Row"(w508) -> ()
        n218 = local read "Treatment Concentration (mM):"() -> (w461:dbl)
        n219 = case shown="False" w420 {
          tunnel: w421 -> [w593 _]
          tunnel: [w590 w597] -> w419
          frame False {
            n220 = local read "Rec: Temp"() -> (w591:dbl)
            n221 = property on="New: Temp" class="DigNum (strict)"("DisabledEnum"=1) -> ()  [unwired: 2 in, 2 out]
            n222 = Equal To 0?(x=w591) -> (x = 0?=w592:bool)
            n223 = local write "New: Temp"(w593) -> ()
            n224 = case shown="True" w592 {
              tunnel: [w594 w595] -> w590
              tunnel: w591 -> [w594 _]
              frame False {
              }
              frame True {
                n225 = local read "Room Temp"() -> (w595:dbl)
              }
            }
            n226 = local write "New: Temp"(w590) -> ()
          }
          frame True {
            n227 = property on="New: Temp" class="DigNum (strict)"("DisabledEnum"=0) -> ()  [unwired: 2 in, 2 out]
            n228 = local read "New: Temp"() -> (w597:dbl)
          }
        }
        n229 = call "Trap Density_STS.vi"("Temp (T) [K]"=w419, "S.T.S. (S)"=w427, "Dielectric"=w426) -> ("Trap Density (N)"=w422:dbl)  [unwired: 8 in]
        n230 = local write "New: Trap Density-STS"(w422) -> ()
        n231 = local read "Rec: Concentration"() -> (w448:dbl)
        n232 = local read "Relative Humidity (%):"() -> (w458:dbl)
        n233 = String Subset(string=w453, offset (0)=1, length (rest)=2) -> (substring=w509:string)
        n234 = Number To Decimal String(number=w513) -> (decimal integer string=w514:string)  [unwired: 1 in]
        n235 = local read "Solution Temp (C):"() -> (w502:dbl)
        n236 = local read "Surface Treatment:"() -> (w460:string)
        n237 = local read "Room Temp (F):"() -> (w506:dbl)
        n238 = local read "Rec: Material"() -> (w456:string)
        n239 = local write "Column"(w509) -> ()
        n240 = local read "New: Length"() -> (w466:dbl)
        n241 = local read "New: Width"() -> (w465:dbl)
        n242 = local read "New: Mobility-Sat"() -> (w495:dbl)
        n243 = local read "Accel (RPM/s):"() -> (w493:dbl)
        n244 = local read "Sample #:"() -> (w485:dbl)
        n245 = local read "# Drops*:"() -> (w503:dbl)
        n246 = local read "Ramp (s):"() -> (w511:dbl)
        n247 = local read "New: STS"() -> (w487:dbl)
        n248 = local read "Rec: Solvent"() -> (w462:string)
        n249 = local read "New: VT-Sat"() -> (w489:dbl)
        n250 = local read "Rec: On/Off"() -> (w491:dbl)
        n251 = local read "Rec: Method"() -> (w486:string)
        n252 = local read "Time (s):"() -> (w498:dbl)
        n253 = local read "Date Recorded"() -> (w482:string)
        n254 = local read "RPM:"() -> (w499:dbl)
        n255 = local read "Fabricator:"() -> (w507:string)
        n256 = Number To Decimal String(number=w448) -> (decimal integer string=w447:string)  [unwired: 1 in]
        n257 = Number To Decimal String(number=w503) -> (decimal integer string=w504:string)  [unwired: 1 in]
        n258 = Number To Decimal String(number=w485) -> (decimal integer string=w478:string)  [unwired: 1 in]
        n259 = call "DeviceID"("Sample"=w478, "Year"=w479, "Month"=w473, "Day"=w469, "Index"=w467) -> ("Result"=w484:string)  [unwired: 9 in, 1 out]
        n260 = Number To Decimal String(number=w466) -> (decimal integer string=w464:string)  [unwired: 1 in]
        n261 = Number To Decimal String(number=w465) -> (decimal integer string=w463:string)  [unwired: 1 in]
        n262 = Number To Decimal String(number=w502) -> (decimal integer string=w501:string)  [unwired: 1 in]
        n263 = Number To Decimal String(number=w458) -> (decimal integer string=w457:string)  [unwired: 1 in]
        n264 = Number To Decimal String(number=w506) -> (decimal integer string=w505:string)  [unwired: 1 in]
        n265 = property on="Image Out" class="ImageControl"() -> ("ZoomSingle"=w551:cluster{"X":sgl, "Y":sgl})  [unwired: 2 in, 2 out]
        n266 = Number To Decimal String(number=w461) -> (decimal integer string=w459:string)  [unwired: 1 in]
        n267 = property on="Image Out" class="ImageControl"() -> ("Bounds"=w552:T11)  [unwired: 2 in, 2 out]
        n268 = Number To Decimal String(number=w499) -> (decimal integer string=w500:string)  [unwired: 1 in]
        n269 = Number To Fractional String(number=w493) -> (F-format string=w494:string)  [unwired: 3 in]
        n270 = Number To Decimal String(number=w498) -> (decimal integer string=w497:string)  [unwired: 1 in]
        n271 = Number To Fractional String(number=w495) -> (F-format string=w496:string)  [unwired: 3 in]
        n272 = Number To Fractional String(number=w491) -> (F-format string=w492:string)  [unwired: 3 in]
        n273 = Number To Fractional String(number=w489) -> (F-format string=w490:string)  [unwired: 3 in]
        n274 = Number To Fractional String(number=w487) -> (F-format string=w488:string)  [unwired: 3 in]
        n275 = Number To Decimal String(number=w511) -> (decimal integer string=w512:string)  [unwired: 1 in]
        n276 = call <vilib>:"Intialize Keyboard.vi"() -> ("device ID"=w563:refnum<k1>)  [unwired: 10 in, 1 out]
        n277 = property on="Image Out" class="ImageControl"() -> ("Image Center Position"=w558:cluster{"X":u32, "Y":u32})  [unwired: 2 in, 2 out]
        n278 = call-poly <vilib>:"Acquire Input Data.vi"("device ID"=w563) -> ("keys pressed"=w562:T12)  [unwired: 16 in, 2 out]
        n279 = Unbundle(w552) -> ("Width"=w549:u32, "Height"=w548:u32)
        n280 = Unbundle(w551) -> ("X"=w526:sgl, "Y"=w550:sgl)
        n281 = Index Array(array=w562) -> (element=w566:T13)  [unwired: 1 in]
        n282 = event shown="[0] \"Remove Button\": Mouse Down" {
          selector: _ -> [_ _ _ _ _ _ _]
          dyn-events: _ -> [_ _ _ _ _ _ _]
          timeout: 10 -> [_ _ _ _ _ _ _]
          event "Remove Button": Mouse Down {
            w618 = 0
            n283 = event-data() -> ()  [unwired: 1 in, 7 out]
            n284 = property on="Image Out" class="ImageControl"() -> ("ROI"=w616:T10)  [unwired: 2 in, 2 out]
            n285 = Unbundle(w616) -> ("Global Rectangle"=w619:i32[], "Contours"=w621:T14)
            n286 = Reverse 1D Array(array=w619) -> (reversed array=w620:i32[])
            n287 = Reverse 1D Array(array=w621) -> (reversed array=w622:T14)
            n288 = Delete From Array(array=w620, index=w618) -> (array with subset deleted=w623:i32[])  [unwired: 1 in, 1 out]
            n289 = Delete From Array(array=w622, index=w618) -> (array with subset deleted=w624:T14)  [unwired: 1 in, 1 out]
            n290 = Reverse 1D Array(array=w623) -> (reversed array=w625:i32[])
            n291 = Reverse 1D Array(array=w624) -> (reversed array=w626:T14)
            n292 = Bundle(w625, w626) -> (w617:T15)  [unwired: 1 in]
            n293 = local write "ROI Descriptor out"(w616) -> ()
            n294 = local write "ROI Descriptor"(w617) -> ()
            n295 = property on="Image Out" class="ImageControl"("ROI"=w617) -> ()  [unwired: 2 in, 2 out]
          }
          event "Undo Button": Mouse Down {
            n296 = event-data() -> ()  [unwired: 1 in, 7 out]
            n297 = invoke on="Image Out" class="ImageControl" method="Clear ROI"() -> ()  [unwired: 3 in, 3 out]
          }
          event "Image Folder": Value Change {
            n298 = event-data() -> ()  [unwired: 1 in, 5 out]
            n299 = local read "Image File"() -> (w628:path)
            n300 = call "Vision Acquisition"("Image Path"=w628) -> ("Image Out"=w627:T2)  [unwired: 25 in, 1 out]
            n301 = local write "Image Out 2"(w627) -> ()
            n302 = local write "Image Out"(w627) -> ()
            n303 = invoke on="Image Out" class="ImageControl" method="Clear ROI"() -> ()  [unwired: 3 in, 3 out]
          }
          event "Zoom": Value Change {
            n304 = event-data() -> ()  [unwired: 1 in, 5 out]
            n305 = local read "Zoom"() -> (w629:i16)
            n306 = Bundle("Zoom"=w629, "Zoom"=w629) -> (w630:cluster{"Zoom":i16, "Zoom":i16})  [unwired: 1 in]
            n307 = property on="Image Out" class="ImageControl"("ZoomInteger"=w630) -> ()  [unwired: 2 in, 2 out]
          }
          event Timeout {
            n308 = event-data() -> ()  [unwired: 1 in, 2 out]
          }
          event "Image Out": Mouse Enter {
            (unwired) 6
            n309 = event-data() -> ()  [unwired: 1 in, 3 out]
            n310 = call "Simulate_Keyboard.vi"("Action"=0, "Virtual Key"=162) -> ()  [unwired: 7 in, 1 out]
          }
          event "Image Out": Mouse Leave {
            n311 = event-data() -> ()  [unwired: 1 in, 3 out]
            n312 = flat-sequence {
              frame #0 {
                n313 = Wait (ms)(milliseconds to wait=10) -> ()  [unwired: 1 out]
              }
              frame #1 {
                (unwired) 6
                n314 = call "Simulate_Keyboard.vi"("Action"=2, "Virtual Key"=162) -> ()  [unwired: 7 in, 1 out]
              }
            }
          }
        }
        n315 = Divide(x=w549, y=w526) -> (x/y=w539:sgl)
        n316 = Multiply(x=w539, y=0.5) -> (x*y=w545:dbl)
        n317 = Divide(x=w548, y=w550) -> (x/y=w538:sgl)
        n318 = Multiply(x=w538, y=0.5) -> (x*y=w544:dbl)
        n319 = Unbundle(w558) -> ("X"=w540:u32, "Y"=w541:u32)
        n320 = Subtract(x=w541, y=w544) -> (x-y=w542:dbl)
        n321 = Subtract(x=w540, y=w545) -> (x-y=w543:dbl)
        n322 = Add(x=w543, y=w539) -> (x+y=w557:dbl)
        n323 = Add(x=w542, y=w538) -> (x+y=w556:dbl)
        n324 = Build Array(w484, w507, w486, w482, w478, w508, w509, w464, w463, w456, w460, w459, w462, w447, w501, w504, w514, w505, w457, w512, w500, w494, w497, w496, w492, w490, w488) -> (w510:string[])
        n325 = local write "Current \nRecord"(w510) -> ()
        n326 = Reciprocal(x=w526) -> (1/x=w525:sgl)
        n327 = event shown="[12] \"Save Changes? 2\": Mouse Down" {
          selector: _ -> [_ _ _ _ _ _ _ _ _ _ _ _ _ _ _ _]
          dyn-events: _ -> [_ _ _ _ _ _ _ _ _ _ _ _ _ _ _ _]
          timeout: 10 -> [_ _ _ _ _ _ _ _ _ _ _ _ _ _ _ _]
          tunnel: [_ _ _ _ _ _ _ _ _ _ _ _ _ TRUE _ TRUE] -> w583
          event Timeout {
            n328 = event-data() -> ()  [unwired: 1 in, 2 out]
          }
          event "Down Button": Mouse Down {
            w970 = 0
            n329 = event-data() -> ()  [unwired: 1 in, 7 out]
            n330 = local read "Transfer File"() -> (w975:path)
            n331 = Strip Path(path=w975) -> (stripped path=w966:path, name=w984:string)
            n332 = local write "Transfer Folder"(w966) -> ()
            n333 = List Folder(path=w966) -> (filenames=w980:string[], error out=w920:errorcluster)  [unwired: 3 in, 2 out]
            n334 = local read "Folder Index"() -> (w922:dbl)
            n335 = Array Size(array=w980) -> (size(s)=w976:i32)
            n336 = Search 1D Array(1D array=w980, element=w984) -> (index of element=w977:i32)  [unwired: 1 in]
            n337 = property on="Image Out" class="ImageControl"() -> (error out=w923:errorcluster, "Image Center Position"=w927:cluster{"X":u32, "Y":u32})  [unwired: 2 in, 1 out]
            n338 = Decrement(x=w976) -> (x-1=w978:i32)
            n339 = Equal?(x=w977, y=w978) -> (x = y?=w979:bool)
            n340 = invoke on="Image Out" class="ImageControl" method="Clear ROI"() -> ()  [unwired: 3 in, 3 out]
            n341 = case shown="False" w979 {
              tunnel: w922 -> [w1137 _]
              tunnel: [w1136 0] -> w921
              tunnel: w920 -> [w1135 w1138]
              tunnel: [w1135 w1138] -> w919
              frame False {
                n342 = Increment(x=w1137) -> (x+1=w1136:dbl)
              }
              frame True {
              }
            }
            n343 = Unbundle(w927) -> ("X"=w925:u32)  [unwired: 1 out]
            n344 = local write "Folder Index"(w921) -> ()
            n345 = Bundle("X"=w925, 0) -> (w926:cluster{"X":u32, i32})  [unwired: 1 in]
            n346 = property on="Image Out" class="ImageControl"(error in=w923, "Image Center Position"=w926) -> ()  [unwired: 1 in, 2 out]
            n347 = Path To String(path=w966) -> (string=w985:string)
            n348 = Index Array(array=w980, index=w921) -> (element=w981:string)
            n349 = local write "Data Name:"(w981) -> ()
            n350 = Concatenate Strings(w985, "\\", w981) -> (w983:string)
            n351 = String To Path(string=w983) -> (path=w893:path)
            n352 = call "Recorded Values.vi"("Path"=w893) -> ("Recorded Char"=w987:T5, "Recorded Prop"=w988:T6, "Fabrication Prop"=w986:T7)  [unwired: 8 in]
            n353 = Unbundle By Name(w987) -> ("Mobility-Sat"=w1000:dbl, "Moblitity-Lin"=w1001:dbl, "On/Off"=w1002:dbl, "Off Current"=w1003:dbl, "Vt-Sat"=w888:dbl, "STS"=w1004:dbl, "Trap Density-VT"=w1005:dbl, "Trap Density-STS"=w1006:dbl)
            n354 = Unbundle By Name(w986) -> ("Date Created"=w1007:string, "Material"=w989:string, "Solvent"=w990:string, "Concentration"=w991:dbl, "Method"=w992:string, "Dielectric (nm)"=w993:dbl, "Treatment"=w994:string, "Comments"=w995:string)
            n355 = Unbundle By Name(w988) -> ("Date Recorded"=w996:string, "Index"=w997:string, "Length"=w998:dbl, "Width"=w999:dbl, "Sample Temp"=w890:dbl)
            n356 = local write "Date Created"(w1007) -> ()
            n357 = local write "Rec: Off I-Sat"(w1003) -> ()
            n358 = local write "Rec: Comments"(w995) -> ()
            n359 = local write "Rec: Material"(w989) -> ()
            n360 = local write "Rec: VT-Sat"(w888) -> ()
            n361 = local write "Rec: Concentration"(w991) -> ()
            n362 = local write "Rec: Method"(w992) -> ()
            n363 = local write "Rec: Dielectric (d)"(w993) -> ()
            n364 = local write "Surface Treatment:"(w994) -> ()
            n365 = local write "Index"(w997) -> ()
            n366 = local write "Rec: Mobility-Sat"(w1000) -> ()
            n367 = local write "Rec: Mobility-Lin"(w1001) -> ()
            n368 = local write "Rec: On/Off"(w1002) -> ()
            n369 = local write "Rec: STS"(w1004) -> ()
            n370 = local write "Rec: Trap Density-VT"(w1005) -> ()
            n371 = local write "Rec: Trap Density-STS"(w1006) -> ()
            n372 = local write "Rec: Solvent"(w990) -> ()
            n373 = local write "Date Recorded"(w996) -> ()
            n374 = local write "Rec: Length"(w998) -> ()
            n375 = local write "Rec: Width"(w999) -> ()
            n376 = local write "Rec: Temp"(w890) -> ()
            n377 = Equal To 0?(x=w890) -> (x = 0?=w891:bool)
            n378 = case shown="True" w891 {
              tunnel: [w1008 w1009] -> w889
              tunnel: w890 -> [w1008 _]
              frame False {
              }
              frame True {
                n379 = local read "Room Temp"() -> (w1009:dbl)
              }
            }
            n380 = local read "NumPts 2"() -> (w914:dbl)
            n381 = local write "Transfer File"(w893) -> ()
            n382 = local read "NumPts"() -> (w918:dbl)
            n383 = call-poly <vilib>:"Read From Spreadsheet File.vi"("file path (dialog if empty)"=w893) -> ("all rows"=w972:string[][])  [unwired: 6 in, 4 out]
            n384 = call "Mobility-Vt Calculator-File.vi"("NumPts"=w918, "Path"=w893) -> ("XY Graph-Sat"=w916:cluster{dbl[], dbl[]}[], "XY Graph-Lin"=w887:cluster{dbl[], dbl[]}[], "Output"=w917:T8, "Index-Sat"=w915:dbl, "Index-Lin"=w901:dbl)  [unwired: 4 in, 1 out]
            n385 = local read "New: Dielectric"() -> (w898:dbl)
            n386 = call "STS Calculator-File.vi"("NumPts"=w914, "Path"=w893) -> ("STS Index-Sat"=w913:dbl, "XY Graph-Sat"=w912:cluster{dbl[], dbl[]}[], "Ouput"=w911:cluster{"STS-Sat":dbl, "STS-Lin":dbl})  [unwired: 5 in, 2 out]
            n387 = Unbundle By Name(w917) -> ("Mobility-Sat"=w910:dbl, "Vt-Sat"=w897:dbl, "Mobility-Lin"=w909:dbl, "Vt-Lin"=w908:dbl, "Off I-Sat"=w894:dbl, "On/Off I-Sat"=w886:dbl)
            n388 = Unbundle By Name(w911) -> ("STS-Sat"=w892:dbl)  [unwired: 1 out]
            n389 = local write "Index 2"(w913) -> ()
            n390 = local write "XY Graph 2"(w912) -> ()
            n391 = local write "MobVi Index"(w915) -> ()
            n392 = local write "Slide"(w915) -> ()
            n393 = local write "XY Graph"(w916) -> ()
            n394 = Array Size(array=w972) -> (size(s)=w971:i32[])
            n395 = call "Trap Density_VT.vi"("VT"=w897, "Dielectric"=w898) -> ("Trap Density-VT"=w896:dbl)
            n396 = call "Trap Density_STS.vi"("Temp (T) [K]"=w889, "S.T.S. (S)"=w892, "Dielectric"=w898) -> ("Trap Density (N)"=w895:dbl)  [unwired: 8 in]
            n397 = local write "New: STS"(w892) -> ()
            n398 = local write "Calc: STS"(w892) -> ()
            n399 = local write "Calc: Mobility-Sat"(w910) -> ()
            n400 = local write "Calc: Off I-Sat"(w908) -> ()
            n401 = local write "Calc: Mobility-Lin"(w909) -> ()
            n402 = Index Array(array=w971, index=w970) -> (element=w952:i32)
            n403 = Decimate 1D Array(w912) -> (w946:cluster{dbl[], dbl[]}[])  [unwired: 1 out]
            n404 = Decimate 1D Array(w916) -> (w956:cluster{dbl[], dbl[]}[])  [unwired: 1 out]
            n405 = local write "Calc: Off I-Sat"(w894) -> ()
            n406 = local write "Calc: On/Off"(w886) -> ()
            n407 = Decimate 1D Array(w887) -> (w907:cluster{dbl[], dbl[]}[])  [unwired: 1 out]
            n408 = local write "Calc: VT-Sat"(w897) -> ()
            n409 = Array Subset(array=w972, index (row)=w970, index (col)=w970, length (col)=3) -> (w973:string[][])  [unwired: 1 in]
            n410 = local write "Calc: Trap Density-VT"(w896) -> ()
            n411 = local write "Calc: Trap Density-STS"(w895) -> ()
            n412 = local write "New: Trap Density-STS"(w895) -> ()
            n413 = local write "New: Trap Density-VT"(w896) -> ()
            n414 = local write "XY Graph-Lin"(w887) -> ()
            n415 = Array To Cluster(array=w946) -> (cluster=w944:T9)
            n416 = Array To Cluster(array=w956) -> (cluster=w958:T9)
            n417 = local write "New: VT-Lin"(w908) -> ()
            n418 = local write "New: VT-Sat"(w897) -> ()
            n419 = local write "New: Mobility-Sat"(w910) -> ()
            n420 = local write "New: Mobility-Lin"(w909) -> ()
            n421 = Reshape Array(w973, w952) -> (w959:string[])
            n422 = Array To Cluster(array=w907) -> (cluster=w906:T9)
            n423 = Subtract(x=w952, y=20) -> (x-y=w951:i32)
            n424 = property on="Slide" class="Slide (strict)"("Scale.Maximum"=w951) -> ()  [unwired: 2 in, 2 out]
            n425 = Unbundle(w944) -> ("[0]"=w945:cluster{dbl[], dbl[]})  [unwired: 8 out]
            n426 = Unbundle(w958) -> ("[0]"=w957:cluster{dbl[], dbl[]})  [unwired: 8 out]
            n427 = Unbundle(w906) -> ("[0]"=w903:cluster{dbl[], dbl[]})  [unwired: 8 out]
            n428 = Search 1D Array(1D array=w959, element="Index:") -> (index of element=w967:i32)  [unwired: 1 in]
            n429 = local read "NumPts"() -> (w902:dbl)
            n430 = Unbundle(w903) -> (w905:dbl[], w904:dbl[])
            n431 = Increment(x=w967) -> (x+1=w968:i32)
            n432 = Unbundle(w945) -> (w943:dbl[], w942:dbl[])
            n433 = Unbundle(w957) -> (w948:dbl[], w947:dbl[])
            n434 = Array Subset(array=w905, index=w901, length=w902) -> (w900:dbl[])
            n435 = Array Subset(array=w904, index=w901, length=w902) -> (w899:dbl[])
            n436 = Array Subset(array=w943, index=w913, length=w914) -> (w950:dbl[])
            n437 = Array Subset(array=w942, index=w913, length=w914) -> (w949:dbl[])
            n438 = Array Subset(array=w948, index=w915, length=w918) -> (w955:dbl[])
            n439 = Array Subset(array=w947, index=w915, length=w918) -> (w954:dbl[])
            n440 = Index Array(array=w959, index=w968) -> (element=w931:string)
            n441 = local write "Lin-Vg Array-Used"(w900) -> ()
            n442 = local write "Sat Vg Array-Used"(w955) -> ()
            n443 = local write "Vg Array-Log-Used"(w949) -> ()
            n444 = local write "Lin Id-Used"(w899) -> ()
            n445 = local read "Image Folder"() -> (w929:path)
            n446 = local write "Sat Id-Used"(w954) -> ()
            n447 = local write "Sat Id-Log-Used"(w950) -> ()
            n448 = List Folder(path=w929, error in=w919) -> (filenames=w965:string[], error out=w932:errorcluster)  [unwired: 2 in, 2 out]
            n449 = while {
              tunnel: w965 -> [w1022]
              tunnel: w931 -> [w1020]
              tunnel: [w1019] -> _
              tunnel: [w1019] -> w964
              tunnel: w952 -> [w1018]
              i -> [w1019]
              stop <- w1015 stop-if-true
              n450 = Index Array(array=w1022, index=w1019) -> (element=w1023:string)
              n451 = xnode "Match Regular Expression"("input string"=w1023, "regular expression"=w1020) -> ("whole match"=w1021:string)  [unwired: 4 in, 4 out]
              n452 = Equal?(x=w1021, y=w1020) -> (x = y?=w1017:bool)
              n453 = Equal?(x=w1018, y=w1019) -> (x = y?=w1016:bool)
              n454 = Or(x=w1017, y=w1016) -> (x .or. y?=w1015:bool)
            }
            n455 = Build Path(base path=w929, name or relative path="ROI") -> (appended path=w928:path)
            n456 = Path To String(path=w929) -> (string=w962:string)
            n457 = Index Array(array=w965, index=w964) -> (element=w940:string)
            n458 = invoke on="Image Out" class="ImageControl" method="Clear ROI"(error in=w932) -> (error out=w935:errorcluster)  [unwired: 2 in, 2 out]
            n459 = local write "Image Name"(w940) -> ()
            n460 = Build Path(base path=w928, name or relative path=w931) -> (appended path=w936:path)
            n461 = call <vilib>:"Check if File or Folder Exists.vi"("error in (no error)"=w935, "path"=w936) -> ("file or folder exists?"=w933:bool, "dup path"=w934:path)  [unwired: 7 in, 1 out]
            n462 = Concatenate Strings(w962, "\\", w940) -> (w961:string)
            n463 = case shown="False" w933 {
              tunnel: w934 -> [_ w1010]
              frame False {
              }
              frame True {
                n464 = Read from Text File(file (use dialog)=w1010) -> (text=w1014:string)  [unwired: 3 in, 3 out]
                n465 = property on="Image Out" class="ImageControl"() -> ("ROI"=w1011:T10)  [unwired: 2 in, 2 out]
                n466 = Unflatten From String(type=w1011, binary string=w1014) -> (value=w1012:T10, error out=w1013:errorcluster)  [unwired: 3 in, 1 out]
                n467 = property on="Image Out" class="ImageControl"(error in=w1013, "ROI"=w1012) -> ()  [unwired: 1 in, 2 out]
              }
            }
            n468 = String To Path(string=w961) -> (path=w939:path)
            n469 = Empty String/Path?(string/path=w940) -> (empty?=w941:bool)
            n470 = local read "No Image File"() -> (w937:path)
            n471 = Select(t=w937, s=w941, f=w939) -> (s? t:f=w938:path)
            n472 = local write "Image File"(w938) -> ()
            n473 = call "Vision Acquisition4"("Image Path"=w938) -> ("Image Out"=w963:T2)  [unwired: 25 in, 1 out]
            n474 = local write "Image Out"(w963) -> ()
            n475 = local write "Image Out 2"(w963) -> ()
          }
          event "Transfer File": Value Change {
            w1246 = 0
            n476 = event-data() -> ()  [unwired: 1 in, 5 out]
            n477 = local read "Transfer File"() -> (w1242:path)
            n478 = Strip Path(path=w1242) -> (stripped path=w1241:path, name=w1255:string)
            n479 = local write "Transfer Folder"(w1241) -> ()
            n480 = property on="Image Out" class="ImageControl"() -> (error out=w1197:errorcluster, "Image Center Position"=w1201:cluster{"X":u32, "Y":u32})  [unwired: 2 in, 1 out]
            n481 = List Folder(path=w1241) -> (filenames=w1251:string[], error out=w1207:errorcluster)  [unwired: 3 in, 2 out]
            n482 = Search 1D Array(1D array=w1251, element=w1255) -> (index of element=w1196:i32)  [unwired: 1 in]
            n483 = local write "Folder Index"(w1196) -> ()
            n484 = Unbundle(w1201) -> ("X"=w1199:u32)  [unwired: 1 out]
            n485 = Path To String(path=w1241) -> (string=w1256:string)
            n486 = Index Array(array=w1251, index=w1196) -> (element=w1252:string)
            n487 = Bundle("X"=w1199, 0) -> (w1200:cluster{"X":u32, i32})  [unwired: 1 in]
            n488 = local write "Data Name:"(w1252) -> ()
            n489 = property on="Image Out" class="ImageControl"(error in=w1197, "Image Center Position"=w1200) -> ()  [unwired: 1 in, 2 out]
            n490 = Concatenate Strings(w1256, "\\", w1252) -> (w1254:string)
            n491 = String To Path(string=w1254) -> (path=w1147:path)
            n492 = call "Recorded Values.vi"("Path"=w1147) -> ("Recorded Char"=w1194:T5, "Recorded Prop"=w1193:T6, "Fabrication Prop"=w1195:T7)  [unwired: 8 in]
            n493 = Unbundle By Name(w1194) -> ("Mobility-Sat"=w1181:dbl, "Moblitity-Lin"=w1180:dbl, "On/Off"=w1179:dbl, "Off Current"=w1178:dbl, "Vt-Sat"=w1143:dbl, "STS"=w1177:dbl, "Trap Density-VT"=w1176:dbl, "Trap Density-STS"=w1175:dbl)
            n494 = Unbundle By Name(w1195) -> ("Date Created"=w1174:string, "Material"=w1192:string, "Solvent"=w1191:string, "Concentration"=w1190:dbl, "Method"=w1189:string, "Dielectric (nm)"=w1188:dbl, "Treatment"=w1187:string, "Comments"=w1186:string)
            n495 = Unbundle By Name(w1193) -> ("Date Recorded"=w1185:string, "Index"=w1184:string, "Length"=w1183:dbl, "Width"=w1182:dbl, "Sample Temp"=w1145:dbl)
            n496 = local write "Date Created"(w1174) -> ()
            n497 = local write "Rec: Material"(w1192) -> ()
            n498 = local write "Rec: Off I-Sat"(w1178) -> ()
            n499 = local write "Rec: Comments"(w1186) -> ()
            n500 = local write "Rec: VT-Sat"(w1143) -> ()
            n501 = local write "Rec: Concentration"(w1190) -> ()
            n502 = local write "Rec: Method"(w1189) -> ()
            n503 = local write "Rec: Dielectric (d)"(w1188) -> ()
            n504 = local write "Surface Treatment:"(w1187) -> ()
            n505 = local write "Index"(w1184) -> ()
            n506 = local write "Rec: Mobility-Sat"(w1181) -> ()
            n507 = local write "Rec: Mobility-Lin"(w1180) -> ()
            n508 = local write "Rec: On/Off"(w1179) -> ()
            n509 = local write "Rec: STS"(w1177) -> ()
            n510 = local write "Rec: Trap Density-VT"(w1176) -> ()
            n511 = local write "Rec: Trap Density-STS"(w1175) -> ()
            n512 = local write "Rec: Solvent"(w1191) -> ()
            n513 = local write "Date Recorded"(w1185) -> ()
            n514 = local write "Rec: Length"(w1183) -> ()
            n515 = local write "Rec: Width"(w1182) -> ()
            n516 = local write "Rec: Temp"(w1145) -> ()
            n517 = Equal To 0?(x=w1145) -> (x = 0?=w1146:bool)
            n518 = case shown="False" w1146 {
              tunnel: [w1257 w1258] -> w1144
              tunnel: w1145 -> [w1257 _]
              frame False {
              }
              frame True {
                n519 = local read "Room Temp"() -> (w1258:dbl)
              }
            }
            n520 = local write "Transfer File"(w1147) -> ()
            n521 = local read "NumPts 2"() -> (w1169:dbl)
            n522 = local read "NumPts"() -> (w1170:dbl)
            n523 = call-poly <vilib>:"Read From Spreadsheet File.vi"("file path (dialog if empty)"=w1147) -> ("all rows"=w1248:string[][])  [unwired: 6 in, 4 out]
            n524 = local read "New: Dielectric"() -> (w1153:dbl)
            n525 = call "STS Calculator-File.vi"("NumPts"=w1169, "Path"=w1147) -> ("STS Index-Sat"=w1167:dbl, "XY Graph-Sat"=w1168:cluster{dbl[], dbl[]}[], "Ouput"=w1166:cluster{"STS-Sat":dbl, "STS-Lin":dbl})  [unwired: 5 in, 2 out]
            n526 = call "Mobility-Vt Calculator-File.vi"("NumPts"=w1170, "Path"=w1147) -> ("XY Graph-Sat"=w1173:cluster{dbl[], dbl[]}[], "XY Graph-Lin"=w1142:cluster{dbl[], dbl[]}[], "Output"=w1171:T8, "Index-Sat"=w1172:dbl, "Index-Lin"=w1159:dbl)  [unwired: 4 in, 1 out]
            n527 = Unbundle By Name(w1171) -> ("Mobility-Sat"=w1155:dbl, "Vt-Sat"=w1149:dbl, "Mobility-Lin"=w1154:dbl, "Vt-Lin"=w1140:dbl, "Off I-Sat"=w1148:dbl, "On/Off I-Sat"=w1141:dbl)
            n528 = local write "Index 2"(w1167) -> ()
            n529 = local write "XY Graph 2"(w1168) -> ()
            n530 = Unbundle By Name(w1166) -> ("STS-Sat"=w1150:dbl)  [unwired: 1 out]
            n531 = local write "MobVi Index"(w1172) -> ()
            n532 = Array Size(array=w1248) -> (size(s)=w1247:i32[])
            n533 = call "Trap Density_VT.vi"("VT"=w1149, "Dielectric"=w1153) -> ("Trap Density-VT"=w1152:dbl)
            n534 = call "Trap Density_STS.vi"("Temp (T) [K]"=w1144, "S.T.S. (S)"=w1150, "Dielectric"=w1153) -> ("Trap Density (N)"=w1151:dbl)  [unwired: 8 in]
            n535 = local write "Slide"(w1172) -> ()
            n536 = local write "Calc: Mobility-Lin"(w1154) -> ()
            n537 = local write "Calc: Mobility-Sat"(w1155) -> ()
            n538 = local write "Calc: VT-Sat"(w1149) -> ()
            n539 = local write "Calc: Off I-Sat"(w1148) -> ()
            n540 = local write "Calc: VT-Lin"(w1140) -> ()
            n541 = local write "Calc: On/Off"(w1141) -> ()
            n542 = local write "Calc: STS"(w1150) -> ()
            n543 = Decimate 1D Array(w1142) -> (w1165:cluster{dbl[], dbl[]}[])  [unwired: 1 out]
            n544 = local write "Calc: Trap Density-VT"(w1152) -> ()
            n545 = local write "Calc: Trap Density-STS"(w1151) -> ()
            n546 = local write "New: Trap Density-STS"(w1151) -> ()
            n547 = local write "New: Trap Density-VT"(w1152) -> ()
            n548 = local write "XY Graph-Lin"(w1142) -> ()
            n549 = local write "New: VT-Sat"(w1149) -> ()
            n550 = Decimate 1D Array(w1168) -> (w1222:cluster{dbl[], dbl[]}[])  [unwired: 1 out]
            n551 = Index Array(array=w1247, index=w1246) -> (element=w1228:i32)
            n552 = Decimate 1D Array(w1173) -> (w1231:cluster{dbl[], dbl[]}[])  [unwired: 1 out]
            n553 = local write "XY Graph"(w1173) -> ()
            n554 = local write "New: Mobility-Lin"(w1154) -> ()
            n555 = Array Subset(array=w1248, index (row)=w1246, index (col)=w1246, length (col)=3) -> (w1249:string[][])  [unwired: 1 in]
            n556 = local write "New: VT-Lin"(w1140) -> ()
            n557 = Array To Cluster(array=w1165) -> (cluster=w1164:T9)
            n558 = local write "New: STS"(w1150) -> ()
            n559 = local write "New: Mobility-Sat"(w1155) -> ()
            n560 = Array To Cluster(array=w1222) -> (cluster=w1220:T9)
            n561 = Array To Cluster(array=w1231) -> (cluster=w1233:T9)
            n562 = Reshape Array(w1249, w1228) -> (w1234:string[])
            n563 = Subtract(x=w1228, y=20) -> (x-y=w1226:i32)
            n564 = Unbundle(w1164) -> ("[0]"=w1163:cluster{dbl[], dbl[]})  [unwired: 8 out]
            n565 = property on="Slide" class="Slide (strict)"("Scale.Maximum"=w1226) -> ()  [unwired: 2 in, 2 out]
            n566 = local read "NumPts"() -> (w1160:dbl)
            n567 = Unbundle(w1163) -> (w1162:dbl[], w1161:dbl[])
            n568 = Unbundle(w1220) -> ("[0]"=w1221:cluster{dbl[], dbl[]})  [unwired: 8 out]
            n569 = Unbundle(w1233) -> ("[0]"=w1232:cluster{dbl[], dbl[]})  [unwired: 8 out]
            n570 = Search 1D Array(1D array=w1234, element="Index:") -> (index of element=w1243:i32)  [unwired: 1 in]
            n571 = local read "NumPts"() -> (w1156:dbl)
            n572 = Array Subset(array=w1162, index=w1159, length=w1160) -> (w1158:dbl[])
            n573 = Array Subset(array=w1161, index=w1159, length=w1160) -> (w1157:dbl[])
            n574 = Increment(x=w1243) -> (x+1=w1244:i32)
            n575 = Unbundle(w1221) -> (w1218:dbl[], w1217:dbl[])
            n576 = Unbundle(w1232) -> (w1219:dbl[], w1223:dbl[])
            n577 = local read "Image Folder"() -> (w1203:path)
            n578 = local write "Lin-Vg Array-Used"(w1158) -> ()
            n579 = Array Subset(array=w1218, index=w1167, length=w1169) -> (w1225:dbl[])
            n580 = Array Subset(array=w1217, index=w1167, length=w1169) -> (w1224:dbl[])
            n581 = Array Subset(array=w1219, index=w1172, length=w1156) -> (w1230:dbl[])
            n582 = Array Subset(array=w1223, index=w1172, length=w1156) -> (w1229:dbl[])
            n583 = Index Array(array=w1234, index=w1244) -> (element=w1205:string)
            n584 = local write "Lin Id-Used"(w1157) -> ()
            n585 = local write "Sat Vg Array-Used"(w1230) -> ()
            n586 = local write "Vg Array-Log-Used"(w1224) -> ()
            n587 = local write "Sat Id-Log-Used"(w1225) -> ()
            n588 = local write "Sat Id-Used"(w1229) -> ()
            n589 = local write "Index"(w1205) -> ()
            n590 = List Folder(path=w1203, error in=w1207) -> (filenames=w1239:string[], error out=w1206:errorcluster)  [unwired: 2 in, 2 out]
            n591 = Build Path(base path=w1203, name or relative path="ROI") -> (appended path=w1202:path)
            n592 = invoke on="Image Out" class="ImageControl" method="Clear ROI"(error in=w1206) -> (error out=w1210:errorcluster)  [unwired: 2 in, 2 out]
            n593 = Build Path(base path=w1202, name or relative path=w1205) -> (appended path=w1211:path)
            n594 = while {
              tunnel: w1239 -> [w1271]
              tunnel: w1205 -> [w1269]
              tunnel: [w1268] -> _
              tunnel: [w1268] -> w1238
              tunnel: w1228 -> [w1267]
              i -> [w1268]
              stop <- w1264 stop-if-true
              n595 = Index Array(array=w1271, index=w1268) -> (element=w1272:string)
              n596 = xnode "Match Regular Expression"("input string"=w1272, "regular expression"=w1269) -> ("whole match"=w1270:string)  [unwired: 4 in, 4 out]
              n597 = Equal?(x=w1270, y=w1269) -> (x = y?=w1266:bool)
              n598 = Equal?(x=w1267, y=w1268) -> (x = y?=w1265:bool)
              n599 = Or(x=w1266, y=w1265) -> (x .or. y?=w1264:bool)
            }
            n600 = call <vilib>:"Check if File or Folder Exists.vi"("error in (no error)"=w1210, "path"=w1211) -> ("file or folder exists?"=w1208:bool, "dup path"=w1209:path)  [unwired: 7 in, 1 out]
            n601 = case shown="True" w1208 {
              tunnel: w1209 -> [_ w1259]
              frame False {
              }
              frame True {
                n602 = Read from Text File(file (use dialog)=w1259) -> (text=w1263:string)  [unwired: 3 in, 3 out]
                n603 = property on="Image Out" class="ImageControl"() -> ("ROI"=w1260:T10)  [unwired: 2 in, 2 out]
                n604 = Unflatten From String(type=w1260, binary string=w1263) -> (value=w1261:T10, error out=w1262:errorcluster)  [unwired: 3 in, 1 out]
                n605 = property on="Image Out" class="ImageControl"(error in=w1262, "ROI"=w1261) -> ()  [unwired: 1 in, 2 out]
              }
            }
            n606 = invoke on="Image Out" class="ImageControl" method="Clear ROI"() -> ()  [unwired: 3 in, 3 out]
            n607 = Path To String(path=w1203) -> (string=w1237:string)
            n608 = Index Array(array=w1239, index=w1238) -> (element=w1215:string)
            n609 = Concatenate Strings(w1237, "\\", w1215) -> (w1236:string)
            n610 = local write "Image Name"(w1215) -> ()
            n611 = String To Path(string=w1236) -> (path=w1214:path)
            n612 = Empty String/Path?(string/path=w1215) -> (empty?=w1216:bool)
            n613 = local read "No Image File"() -> (w1212:path)
            n614 = Select(t=w1212, s=w1216, f=w1214) -> (s? t:f=w1213:path)
            n615 = local write "Image File"(w1213) -> ()
            n616 = call "Vision Acquisition3"("Image Path"=w1213) -> ("Image Out"=w1240:T2)  [unwired: 25 in, 1 out]
            n617 = local write "Image Out"(w1240) -> ()
            n618 = local write "Image Out 2"(w1240) -> ()
          }
          event "Up Button": Mouse Down {
            w1491 = 0
            n619 = event-data() -> ()  [unwired: 1 in, 5 out]
            n620 = local read "Transfer File"() -> (w1487:path)
            n621 = Strip Path(path=w1487) -> (stripped path=w1486:path, name=w1502:string)
            n622 = local write "Transfer Folder"(w1486) -> ()
            n623 = List Folder(path=w1486) -> (filenames=w1496:string[], error out=w1453:errorcluster)  [unwired: 3 in, 2 out]
            n624 = Array Size(array=w1496) -> (size(s)=w1441:i32)
            n625 = Search 1D Array(1D array=w1496, element=w1502) -> (index of element=w1497:i32)  [unwired: 1 in]
            n626 = Equal To 0?(x=w1497) -> (x = 0?=w1498:bool)
            n627 = local read "Folder Index"() -> (w1440:dbl)
            n628 = property on="Image Out" class="ImageControl"() -> (error out=w1443:errorcluster, "Image Center Position"=w1447:cluster{"X":u32, "Y":u32})  [unwired: 2 in, 1 out]
            n629 = case shown="True" w1498 {
              tunnel: w1440 -> [w1632 _]
              tunnel: [w1631 w1633] -> w1439
              tunnel: w1441 -> [_ w1634]
              frame False {
                n630 = Decrement(x=w1632) -> (x-1=w1631:dbl)
              }
              frame True {
                n631 = Decrement(x=w1634) -> (x-1=w1633:i32)
              }
            }
            n632 = Unbundle(w1447) -> ("X"=w1445:u32)  [unwired: 1 out]
            n633 = local write "Folder Index"(w1439) -> ()
            n634 = Bundle("X"=w1445, 0) -> (w1446:cluster{"X":u32, i32})  [unwired: 1 in]
            n635 = Path To String(path=w1486) -> (string=w1503:string)
            n636 = Index Array(array=w1496, index=w1439) -> (element=w1499:string)
            n637 = local write "Data Name:"(w1499) -> ()
            n638 = property on="Image Out" class="ImageControl"(error in=w1443, "Image Center Position"=w1446) -> ()  [unwired: 1 in, 2 out]
            n639 = Concatenate Strings(w1503, "\\", w1499) -> (w1501:string)
            n640 = String To Path(string=w1501) -> (path=w1390:path)
            n641 = call "Recorded Values.vi"("Path"=w1390) -> ("Recorded Char"=w1437:T5, "Recorded Prop"=w1436:T6, "Fabrication Prop"=w1438:T7)  [unwired: 8 in]
            n642 = Unbundle By Name(w1437) -> ("Mobility-Sat"=w1424:dbl, "Moblitity-Lin"=w1423:dbl, "On/Off"=w1422:dbl, "Off Current"=w1421:dbl, "Vt-Sat"=w1386:dbl, "STS"=w1420:dbl, "Trap Density-VT"=w1419:dbl, "Trap Density-STS"=w1418:dbl)
            n643 = Unbundle By Name(w1438) -> ("Date Created"=w1417:string, "Material"=w1435:string, "Solvent"=w1434:string, "Concentration"=w1433:dbl, "Method"=w1432:string, "Dielectric (nm)"=w1431:dbl, "Treatment"=w1430:string, "Comments"=w1429:string)
            n644 = Unbundle By Name(w1436) -> ("Date Recorded"=w1428:string, "Index"=w1427:string, "Length"=w1426:dbl, "Width"=w1425:dbl, "Sample Temp"=w1387:dbl)
            n645 = local write "Date Created"(w1417) -> ()
            n646 = local write "Rec: Material"(w1435) -> ()
            n647 = local write "Rec: Off I-Sat"(w1421) -> ()
            n648 = local write "Rec: Comments"(w1429) -> ()
            n649 = local write "Rec: VT-Sat"(w1386) -> ()
            n650 = local write "Rec: Solvent"(w1434) -> ()
            n651 = local write "Rec: Concentration"(w1433) -> ()
            n652 = local write "Rec: Method"(w1432) -> ()
            n653 = local write "Rec: Dielectric (d)"(w1431) -> ()
            n654 = local write "Surface Treatment:"(w1430) -> ()
            n655 = local write "Index"(w1427) -> ()
            n656 = local write "Rec: Mobility-Sat"(w1424) -> ()
            n657 = local write "Rec: Mobility-Lin"(w1423) -> ()
            n658 = local write "Rec: On/Off"(w1422) -> ()
            n659 = local write "Rec: STS"(w1420) -> ()
            n660 = local write "Rec: Trap Density-VT"(w1419) -> ()
            n661 = local write "Rec: Trap Density-STS"(w1418) -> ()
            n662 = local write "Date Recorded"(w1428) -> ()
            n663 = local write "Rec: Length"(w1426) -> ()
            n664 = local write "Rec: Width"(w1425) -> ()
            n665 = local write "Rec: Temp"(w1387) -> ()
            n666 = Equal To 0?(x=w1387) -> (x = 0?=w1389:bool)
            n667 = case shown="False" w1389 {
              tunnel: [w1504 w1505] -> w1388
              tunnel: w1387 -> [w1504 _]
              frame False {
              }
              frame True {
                n668 = local read "Room Temp"() -> (w1505:dbl)
              }
            }
            n669 = local write "Transfer File"(w1390) -> ()
            n670 = local read "NumPts 2"() -> (w1412:dbl)
            n671 = local read "NumPts"() -> (w1416:dbl)
            n672 = local read "New: Dielectric"() -> (w1396:dbl)
            n673 = call "Mobility-Vt Calculator-File.vi"("NumPts"=w1416, "Path"=w1390) -> ("XY Graph-Sat"=w1414:cluster{dbl[], dbl[]}[], "XY Graph-Lin"=w1385:cluster{dbl[], dbl[]}[], "Output"=w1415:T8, "Index-Sat"=w1413:dbl, "Index-Lin"=w1400:dbl)  [unwired: 4 in, 1 out]
            n674 = call "STS Calculator-File.vi"("NumPts"=w1412, "Path"=w1390) -> ("STS Index-Sat"=w1411:dbl, "XY Graph-Sat"=w1410:cluster{dbl[], dbl[]}[], "Ouput"=w1409:cluster{"STS-Sat":dbl, "STS-Lin":dbl})  [unwired: 5 in, 2 out]
            n675 = call-poly <vilib>:"Read From Spreadsheet File.vi"("file path (dialog if empty)"=w1390) -> ("all rows"=w1493:string[][])  [unwired: 6 in, 4 out]
            n676 = Unbundle By Name(w1415) -> ("Mobility-Sat"=w1399:dbl, "Vt-Sat"=w1392:dbl, "Mobility-Lin"=w1398:dbl, "Vt-Lin"=w1397:dbl, "Off I-Sat"=w1391:dbl, "On/Off I-Sat"=w1384:dbl)
            n677 = Unbundle By Name(w1409) -> ("STS-Sat"=w1393:dbl)  [unwired: 1 out]
            n678 = local write "Index 2"(w1411) -> ()
            n679 = local write "XY Graph 2"(w1410) -> ()
            n680 = local write "MobVi Index"(w1413) -> ()
            n681 = local write "Slide"(w1413) -> ()
            n682 = local write "XY Graph"(w1414) -> ()
            n683 = local write "Calc: Mobility-Sat"(w1399) -> ()
            n684 = local write "Calc: VT-Sat"(w1392) -> ()
            n685 = local write "Calc: Mobility-Lin"(w1398) -> ()
            n686 = local write "Calc: Off I-Sat"(w1391) -> ()
            n687 = local write "Calc: On/Off"(w1384) -> ()
            n688 = Array Size(array=w1493) -> (size(s)=w1492:i32[])
            n689 = local write "Calc: VT-Lin"(w1397) -> ()
            n690 = call "Trap Density_VT.vi"("VT"=w1392, "Dielectric"=w1396) -> ("Trap Density-VT"=w1395:dbl)
            n691 = call "Trap Density_STS.vi"("Temp (T) [K]"=w1388, "S.T.S. (S)"=w1393, "Dielectric"=w1396) -> ("Trap Density (N)"=w1394:dbl)  [unwired: 8 in]
            n692 = local write "Calc: STS"(w1393) -> ()
            n693 = local write "New: STS"(w1393) -> ()
            n694 = Decimate 1D Array(w1385) -> (w1408:cluster{dbl[], dbl[]}[])  [unwired: 1 out]
            n695 = local write "Calc: Trap Density-VT"(w1395) -> ()
            n696 = local write "New: VT-Sat"(w1392) -> ()
            n697 = local write "Calc: Trap Density-STS"(w1394) -> ()
            n698 = local write "New: Trap Density-STS"(w1394) -> ()
            n699 = local write "New: Trap Density-VT"(w1395) -> ()
            n700 = local write "XY Graph-Lin"(w1385) -> ()
            n701 = local write "New: VT-Lin"(w1397) -> ()
            n702 = local write "New: Mobility-Sat"(w1399) -> ()
            n703 = local write "New: Mobility-Lin"(w1398) -> ()
            n704 = Decimate 1D Array(w1410) -> (w1470:cluster{dbl[], dbl[]}[])  [unwired: 1 out]
            n705 = Index Array(array=w1492, index=w1491) -> (element=w1476:i32)
            n706 = Decimate 1D Array(w1414) -> (w1480:cluster{dbl[], dbl[]}[])  [unwired: 1 out]
            n707 = Array To Cluster(array=w1408) -> (cluster=w1407:T9)
            n708 = Array Subset(array=w1493, index (row)=w1491, index (col)=w1491, length (col)=3) -> (w1494:string[][])  [unwired: 1 in]
            n709 = Array To Cluster(array=w1470) -> (cluster=w1468:T9)
            n710 = Array To Cluster(array=w1480) -> (cluster=w1482:T9)
            n711 = Reshape Array(w1494, w1476) -> (w1483:string[])
            n712 = Subtract(x=w1476, y=20) -> (x-y=w1475:i32)
            n713 = Unbundle(w1407) -> ("[0]"=w1404:cluster{dbl[], dbl[]})  [unwired: 8 out]
            n714 = property on="Slide" class="Slide (strict)"("Scale.Maximum"=w1475) -> ()  [unwired: 2 in, 2 out]
            n715 = Unbundle(w1468) -> ("[0]"=w1469:cluster{dbl[], dbl[]})  [unwired: 8 out]
            n716 = Unbundle(w1482) -> ("[0]"=w1481:cluster{dbl[], dbl[]})  [unwired: 8 out]
            n717 = local read "NumPts"() -> (w1401:dbl)
            n718 = Unbundle(w1404) -> (w1403:dbl[], w1402:dbl[])
            n719 = Search 1D Array(1D array=w1483, element="Index:") -> (index of element=w1488:i32)  [unwired: 1 in]
            n720 = Increment(x=w1488) -> (x+1=w1489:i32)
            n721 = Unbundle(w1469) -> (w1467:dbl[], w1466:dbl[])
            n722 = Unbundle(w1481) -> (w1474:dbl[], w1473:dbl[])
            n723 = Array Subset(array=w1403, index=w1400, length=w1401) -> (w1405:dbl[])
            n724 = Array Subset(array=w1402, index=w1400, length=w1401) -> (w1406:dbl[])
            n725 = local read "Image Folder"() -> (w1442:path)
            n726 = local write "Lin-Vg Array-Used"(w1405) -> ()
            n727 = Array Subset(array=w1467, index=w1411, length=w1412) -> (w1472:dbl[])
            n728 = Array Subset(array=w1466, index=w1411, length=w1412) -> (w1471:dbl[])
            n729 = Array Subset(array=w1474, index=w1413, length=w1416) -> (w1479:dbl[])
            n730 = Array Subset(array=w1473, index=w1413, length=w1416) -> (w1478:dbl[])
            n731 = local write "Lin Id-Used"(w1406) -> ()
            n732 = Index Array(array=w1483, index=w1489) -> (element=w1449:string)
            n733 = local write "Sat Vg Array-Used"(w1479) -> ()
            n734 = local write "Vg Array-Log-Used"(w1471) -> ()
            n735 = local write "Sat Id-Log-Used"(w1472) -> ()
            n736 = local write "Sat Id-Used"(w1478) -> ()
            n737 = local write "Index"(w1449) -> ()
            n738 = List Folder(path=w1442, error in=w1453) -> (filenames=w1485:string[], error out=w1452:errorcluster)  [unwired: 2 in, 2 out]
            n739 = Build Path(base path=w1442, name or relative path="ROI") -> (appended path=w1450:path)
            n740 = invoke on="Image Out" class="ImageControl" method="Clear ROI"(error in=w1452) -> (error out=w1456:errorcluster)  [unwired: 2 in, 2 out]
            n741 = while {
              tunnel: w1485 -> [w1518]
              tunnel: w1449 -> [w1516]
              tunnel: [w1515] -> w1484
              tunnel: w1476 -> [w1514]
              i -> [w1515]
              stop <- w1511 stop-if-true
              n742 = Index Array(array=w1518, index=w1515) -> (element=w1519:string)
              n743 = xnode "Match Regular Expression"("input string"=w1519, "regular expression"=w1516) -> ("whole match"=w1517:string)  [unwired: 4 in, 4 out]
              n744 = Equal?(x=w1517, y=w1516) -> (x = y?=w1513:bool)
              n745 = Equal?(x=w1514, y=w1515) -> (x = y?=w1512:bool)
              n746 = Or(x=w1513, y=w1512) -> (x .or. y?=w1511:bool)
            }
            n747 = Build Path(base path=w1450, name or relative path=w1449) -> (appended path=w1448:path)
            n748 = call <vilib>:"Check if File or Folder Exists.vi"("error in (no error)"=w1456, "path"=w1448) -> ("file or folder exists?"=w1454:bool, "dup path"=w1455:path)  [unwired: 7 in, 1 out]
            n749 = case shown="True" w1454 {
              tunnel: w1455 -> [_ w1506]
              frame False {
              }
              frame True {
                n750 = Read from Text File(file (use dialog)=w1506) -> (text=w1510:string)  [unwired: 3 in, 3 out]
                n751 = property on="Image Out" class="ImageControl"() -> ("ROI"=w1507:T10)  [unwired: 2 in, 2 out]
                n752 = Unflatten From String(type=w1507, binary string=w1510) -> (value=w1508:T10, error out=w1509:errorcluster)  [unwired: 3 in, 1 out]
                n753 = property on="Image Out" class="ImageControl"(error in=w1509, "ROI"=w1508) -> ()  [unwired: 1 in, 2 out]
              }
            }
            n754 = Index Array(array=w1485, index=w1484) -> (element=w1458:string)
            n755 = local write "Image Name"(w1458) -> ()
            n756 = Empty String/Path?(string/path=w1458) -> (empty?=w1465:bool)
            n757 = Build Path(base path=w1442, name or relative path=w1458) -> (appended path=w1457:path)
            n758 = local read "No Image File"() -> (w1464:path)
            n759 = Select(t=w1464, s=w1465, f=w1457) -> (s? t:f=w1459:path)
            n760 = call <vilib>:"Get File Extension.vi"("file"=w1459) -> ("lowercase file extension"=w1461:string)  [unwired: 7 in, 3 out]
            n761 = local write "Image File"(w1459) -> ()
            n762 = local write "String"(w1461) -> ()
            n763 = Search 1D Array(1D array=string[] ["bmp", "jpeg", "png", "jpg", "gif"], element=w1461) -> (index of element=w1460:i32)  [unwired: 1 in]
            n764 = call "Vision Acquisition5"("Image Path"=w1459) -> ("Image Out"=w1463:T2)  [unwired: 25 in, 1 out]
            n765 = Less Than 0?(x=w1460) -> ()  [unwired: 1 out]
            n766 = local write "Image Out"(w1463) -> ()
            n767 = local write "Image Out 2"(w1463) -> ()
          }
          event "Save Changes? 3": Mouse Down {
            n768 = event-data() -> ()  [unwired: 1 in, 7 out]
            n769 = local read "Image Folder"() -> (w1635:path)
            n770 = Build Path(base path=w1635, name or relative path="ROI") -> (appended path=w1642:path)
            n771 = call <vilib>:"Check if File or Folder Exists.vi"("path"=w1642) -> ("file or folder exists?"=w1644:bool, "dup path"=w1641:path)  [unwired: 8 in, 1 out]
            n772 = case shown="False" w1644 {
              tunnel: w1641 -> [w1646 w1647]
              tunnel: [w1645 w1647] -> w1636
              frame False {
                n773 = Create Folder(path (use dialog)=w1646) -> (created path=w1645:path)  [unwired: 2 in, 2 out]
              }
              frame True {
              }
            }
            n774 = local read "Index"() -> (w1638:string)
            n775 = property on="Image Out" class="ImageControl"() -> ("ROI"=w1640:T10)  [unwired: 2 in, 2 out]
            n776 = Build Path(base path=w1636, name or relative path=w1638) -> (appended path=w1637:path)
            n777 = Flatten To String(anything=w1640) -> (data string=w1639:string)  [unwired: 3 in, 2 out]
            n778 = Write to Text File(file (use dialog)=w1637, text=w1639) -> ()  [unwired: 2 in, 3 out]
          }
          event "Next Button": Mouse Down {
            n779 = event-data() -> ()  [unwired: 1 in, 5 out]
            n780 = local read "XY Graph"() -> (w1660:cluster{dbl[], dbl[]}[])
            n781 = Decimate 1D Array(w1660) -> (w1656:cluster{dbl[], dbl[]}[], w1655:cluster{dbl[], dbl[]}[])
            n782 = Array To Cluster(array=w1656) -> (cluster=w1666:T9)
            n783 = local read "MobVi Index"() -> (w1662:dbl)
            n784 = Unbundle(w1666) -> ("[0]"=w1665:cluster{dbl[], dbl[]})  [unwired: 8 out]
            n785 = local read "NumPts"() -> (w1661:dbl)
            n786 = Unbundle(w1665) -> (w1664:dbl[], w1663:dbl[])
            n787 = Increment(x=w1662) -> (x+1=w1657:dbl)
            n788 = local read "New: Dielectric"() -> (w1651:dbl)
            n789 = local read "New: Length"() -> (w1650:dbl)
            n790 = local read "New: Width"() -> (w1649:dbl)
            n791 = local write "MobVi Index"(w1657) -> ()
            n792 = Array Subset(array=w1664, index=w1657, length=w1661) -> (w1653:dbl[])
            n793 = Array Subset(array=w1663, index=w1657, length=w1661) -> (w1652:dbl[])
            n794 = local write "Sat Vg Array-Used"(w1653) -> ()
            n795 = local write "Sat Id-Used"(w1652) -> ()
            n796 = call "Mobility-Vt-Used Pts_Saturation.vi"("Width"=w1649, "Length"=w1650, "Dielectric (d)"=w1651, "Sat Id Used"=w1652, "Vg Used"=w1653) -> ("Vt"=w1648:dbl, "Mobility"=w1654:dbl)  [unwired: 4 in, 1 out]
            n797 = Bundle(w1653, w1652) -> (w1659:cluster{dbl[], dbl[]})  [unwired: 1 in]
            n798 = Build Array (concatenate)(w1656, w1655, w1659) -> (w1658:cluster{dbl[], dbl[]}[])
            n799 = local write "New: Mobility-Sat"(w1654) -> ()
            n800 = local write "New: VT-Sat"(w1648) -> ()
            n801 = local write "XY Graph"(w1658) -> ()
          }
          event "Next Button 2": Mouse Down {
            n802 = event-data() -> ()  [unwired: 1 in, 7 out]
            n803 = local read "XY Graph 2"() -> (w1675:cluster{dbl[], dbl[]}[])
            n804 = Decimate 1D Array(w1675) -> (w1671:cluster{dbl[], dbl[]}[], w1670:cluster{dbl[], dbl[]}[])
            n805 = Array To Cluster(array=w1671) -> (cluster=w1681:T9)
            n806 = local read "Index 2"() -> (w1677:dbl)
            n807 = Unbundle(w1681) -> ("[0]"=w1680:cluster{dbl[], dbl[]})  [unwired: 8 out]
            n808 = local read "NumPts 2"() -> (w1676:dbl)
            n809 = Unbundle(w1680) -> (w1679:dbl[], w1678:dbl[])
            n810 = Increment(x=w1677) -> (x+1=w1672:dbl)
            n811 = local write "Index 2"(w1672) -> ()
            n812 = Array Subset(array=w1678, index=w1672, length=w1676) -> (w1667:dbl[])
            n813 = Array Subset(array=w1679, index=w1672, length=w1676) -> (w1668:dbl[])
            n814 = call "STS-Used.vi"("Id Used"=w1668, "Vg-Used"=w1667) -> ("STS"=w1669:dbl)  [unwired: 9 in]
            n815 = Bundle(w1668, w1667) -> (w1674:cluster{dbl[], dbl[]})  [unwired: 1 in]
            n816 = local write "Vg Array-Log-Used"(w1667) -> ()
            n817 = local write "Sat Id-Log-Used"(w1668) -> ()
            n818 = local write "New: STS"(w1669) -> ()
            n819 = Build Array (concatenate)(w1671, w1670, w1674) -> (w1673:cluster{dbl[], dbl[]}[])
            n820 = local write "XY Graph 2"(w1673) -> ()
          }
          event "Previous Button 2": Mouse Down {
            n821 = event-data() -> ()  [unwired: 1 in, 7 out]
            n822 = local read "XY Graph 2"() -> (w1691:cluster{dbl[], dbl[]}[])
            n823 = Decimate 1D Array(w1691) -> (w1688:cluster{dbl[], dbl[]}[], w1687:cluster{dbl[], dbl[]}[])
            n824 = Array To Cluster(array=w1688) -> (cluster=w1696:T9)
            n825 = local read "Index 2"() -> (w1684:dbl)
            n826 = Unbundle(w1696) -> ("[0]"=w1695:cluster{dbl[], dbl[]})  [unwired: 8 out]
            n827 = local read "NumPts 2"() -> (w1692:dbl)
            n828 = Unbundle(w1695) -> (w1694:dbl[], w1693:dbl[])
            n829 = Decrement(x=w1684) -> (x-1=w1685:dbl)
            n830 = local write "Index 2"(w1685) -> ()
            n831 = Array Subset(array=w1694, index=w1685, length=w1692) -> (w1682:dbl[])
            n832 = Array Subset(array=w1693, index=w1685, length=w1692) -> (w1683:dbl[])
            n833 = local write "Vg Array-Log-Used"(w1683) -> ()
            n834 = local write "Sat Id-Log-Used"(w1682) -> ()
            n835 = Bundle(w1682, w1683) -> (w1690:cluster{dbl[], dbl[]})  [unwired: 1 in]
            n836 = call "STS-Used.vi"("Id Used"=w1682, "Vg-Used"=w1683) -> ("STS"=w1686:dbl)  [unwired: 9 in]
            n837 = Build Array (concatenate)(w1688, w1687, w1690) -> (w1689:cluster{dbl[], dbl[]}[])
            n838 = local write "New: STS"(w1686) -> ()
            n839 = local write "XY Graph 2"(w1689) -> ()
          }
          event "Previous Button": Mouse Down {
            n840 = event-data() -> ()  [unwired: 1 in, 5 out]
            n841 = local read "XY Graph"() -> (w1710:cluster{dbl[], dbl[]}[])
            n842 = Decimate 1D Array(w1710) -> (w1707:cluster{dbl[], dbl[]}[], w1706:cluster{dbl[], dbl[]}[])
            n843 = Array To Cluster(array=w1707) -> (cluster=w1715:T9)
            n844 = local read "MobVi Index"() -> (w1705:dbl)
            n845 = Unbundle(w1715) -> ("[0]"=w1714:cluster{dbl[], dbl[]})  [unwired: 8 out]
            n846 = local read "NumPts"() -> (w1711:dbl)
            n847 = Unbundle(w1714) -> (w1713:dbl[], w1712:dbl[])
            n848 = Decrement(x=w1705) -> (x-1=w1704:dbl)
            n849 = local read "New: Dielectric"() -> (w1698:dbl)
            n850 = local read "New: Length"() -> (w1699:dbl)
            n851 = local read "New: Width"() -> (w1700:dbl)
            n852 = local write "MobVi Index"(w1704) -> ()
            n853 = Array Subset(array=w1713, index=w1704, length=w1711) -> (w1703:dbl[])
            n854 = Array Subset(array=w1712, index=w1704, length=w1711) -> (w1702:dbl[])
            n855 = local write "Sat Vg Array-Used"(w1703) -> ()
            n856 = local write "Sat Id-Used"(w1702) -> ()
            n857 = call "Mobility-Vt-Used Pts_Linear.vi"("Width"=w1700, "Length"=w1699, "Dielectric (d)"=w1698, "Sat Id Used"=w1702, "Vg Used"=w1703) -> ("Vt"=w1697:dbl, "Mobility"=w1701:dbl)  [unwired: 4 in, 1 out]
            n858 = Bundle(w1703, w1702) -> (w1709:cluster{dbl[], dbl[]})  [unwired: 1 in]
            n859 = local write "New: VT-Sat"(w1697) -> ()
            n860 = Build Array (concatenate)(w1707, w1706, w1709) -> (w1708:cluster{dbl[], dbl[]}[])
            n861 = local write "New: Mobility-Sat"(w1701) -> ()
            n862 = local write "XY Graph"(w1708) -> ()
          }
          event "Slide": Value Change {
            n863 = event-data() -> ()  [unwired: 1 in, 5 out]
            n864 = local read "XY Graph"() -> (w1728:cluster{dbl[], dbl[]}[])
            n865 = Decimate 1D Array(w1728) -> (w1725:cluster{dbl[], dbl[]}[], w1724:cluster{dbl[], dbl[]}[])
            n866 = Array To Cluster(array=w1725) -> (cluster=w1733:T9)
            n867 = Unbundle(w1733) -> ("[0]"=w1732:cluster{dbl[], dbl[]})  [unwired: 8 out]
            n868 = local read "NumPts"() -> (w1729:dbl)
            n869 = local read "Slide"() -> (w1717:dbl)
            n870 = Unbundle(w1732) -> (w1731:dbl[], w1730:dbl[])
            n871 = local read "New: Dielectric"() -> (w1718:dbl)
            n872 = local read "New: Length"() -> (w1719:dbl)
            n873 = local read "New: Width"() -> (w1720:dbl)
            n874 = local write "MobVi Index"(w1717) -> ()
            n875 = Array Subset(array=w1731, index=w1717, length=w1729) -> (w1723:dbl[])
            n876 = Array Subset(array=w1730, index=w1717, length=w1729) -> (w1722:dbl[])
            n877 = local write "Sat Vg Array-Used"(w1723) -> ()
            n878 = local write "Sat Id-Used"(w1722) -> ()
            n879 = call "Mobility-Vt-Used Pts_Linear.vi"("Width"=w1720, "Length"=w1719, "Dielectric (d)"=w1718, "Sat Id Used"=w1722, "Vg Used"=w1723) -> ("Vt"=w1716:dbl, "Mobility"=w1721:dbl)  [unwired: 4 in, 1 out]
            n880 = Bundle(w1723, w1722) -> (w1727:cluster{dbl[], dbl[]})  [unwired: 1 in]
            n881 = local write "New: VT-Sat"(w1716) -> ()
            n882 = Build Array (concatenate)(w1725, w1724, w1727) -> (w1726:cluster{dbl[], dbl[]}[])
            n883 = local write "New: Mobility-Sat"(w1721) -> ()
            n884 = local write "XY Graph"(w1726) -> ()
          }
          event "Slide 2": Value Change {
            n885 = event-data() -> ()  [unwired: 1 in, 5 out]
            n886 = local read "XY Graph 2"() -> (w1742:cluster{dbl[], dbl[]}[])
            n887 = Decimate 1D Array(w1742) -> (w1739:cluster{dbl[], dbl[]}[], w1738:cluster{dbl[], dbl[]}[])
            n888 = Array To Cluster(array=w1739) -> (cluster=w1747:T9)
            n889 = Unbundle(w1747) -> ("[0]"=w1746:cluster{dbl[], dbl[]})  [unwired: 8 out]
            n890 = local read "NumPts 2"() -> (w1743:dbl)
            n891 = local read "Slide 2"() -> (w1737:dbl)
            n892 = Unbundle(w1746) -> (w1745:dbl[], w1744:dbl[])
            n893 = local write "Index 2"(w1737) -> ()
            n894 = Array Subset(array=w1745, index=w1737, length=w1743) -> (w1735:dbl[])
            n895 = Array Subset(array=w1744, index=w1737, length=w1743) -> (w1734:dbl[])
            n896 = local write "Vg Array-Log-Used"(w1734) -> ()
            n897 = local write "Sat Id-Log-Used"(w1735) -> ()
            n898 = call "STS-Used.vi"("Id Used"=w1735, "Vg-Used"=w1734) -> ("STS"=w1736:dbl)  [unwired: 9 in]
            n899 = Bundle(w1735, w1734) -> (w1741:cluster{dbl[], dbl[]})  [unwired: 1 in]
            n900 = local write "New: STS"(w1736) -> ()
            n901 = Build Array (concatenate)(w1739, w1738, w1741) -> (w1740:cluster{dbl[], dbl[]}[])
            n902 = local write "XY Graph 2"(w1740) -> ()
          }
          event "Save Changes?": Mouse Down {
            n903 = event-data() -> ()  [unwired: 1 in, 5 out]
            n904 = flat-sequence {
              tunnel: [w1754] -> w1752
              tunnel: [w1762] -> w1751
              tunnel: [w1755] -> w1750
              tunnel: w1752 -> [w2294]
              tunnel: w1751 -> [w2291]
              tunnel: [w2292] -> w1749
              tunnel: w1750 -> [w2292]
              tunnel: [w2291] -> w1748
              tunnel: w1749 -> [w2299]
              tunnel: w1748 -> [w2298]
              frame #0 {
                n905 = Wait (ms)(milliseconds to wait=1) -> ()  [unwired: 1 out]
              }
              frame #1 {
                n906 = local read "Transfer File"() -> (w1754:path)
                n907 = local read "New: Temp"() -> (w1756:dbl)
                n908 = local read "New: Length"() -> (w1760:dbl)
                n909 = local read "New: Width"() -> (w1758:dbl)
                n910 = To Single Precision Float(number=w1756) -> (single precision float=w1757:sgl)
                n911 = Number To Decimal String(number=w1757) -> (decimal integer string=w1765:string)  [unwired: 1 in]
                n912 = To Single Precision Float(number=w1758) -> (single precision float=w1759:sgl)
                n913 = To Single Precision Float(number=w1760) -> (single precision float=w1761:sgl)
                n914 = local read "Index"() -> (w1770:string)
                n915 = Strip Path(path=w1754) -> (stripped path=w1775:path)  [unwired: 1 out]
                n916 = Number To Decimal String(number=w1761) -> (decimal integer string=w1768:string)  [unwired: 1 in]
                n917 = Number To Decimal String(number=w1759) -> (decimal integer string=w1769:string)  [unwired: 1 in]
                n918 = Concatenate Strings("_", w1765, "K") -> (w1763:string)
                n919 = call "Build Text"("Temp"=w1763, "Index"=w1770, "Length"=w1768, "Width"=w1769) -> ("Result"=w1771:string)  [unwired: 10 in, 1 out]
                n920 = flat-sequence {
                  tunnel: [w2248] -> w1767
                  tunnel: w1767 -> [w2265]
                  frame #0 {
                    # "Makes Empty File for Transformer Data"
                    n921 = local read "Transfer Folder"() -> (w2237:path)
                    n922 = Build Path(base path=w2237, name or relative path="Stats") -> (appended path=w2239:path)
                    n923 = call <vilib>:"Check if File or Folder Exists.vi"("path"=w2239) -> ("file or folder exists?"=w2240:bool, "dup path"=w2241:path)  [unwired: 8 in, 1 out]
                    n924 = case shown="False" w2240 {
                      tunnel: [w2245 w2247] -> w2242
                      tunnel: w2241 -> [w2246 w2247]
                      frame False {
                        n925 = Create Folder(path (use dialog)=w2246) -> (created path=w2245:path)  [unwired: 2 in, 2 out]
                      }
                      frame True {
                      }
                    }
                    n926 = Build Path(base path=w2242, name or relative path="Tranformer Data.txt") -> (appended path=w2244:path)
                    n927 = call-poly <vilib>:"Write To Spreadsheet File.vi"("append to file? (new file:F)"=TRUE, "file path (dialog if empty)"=w2244) -> ()  [unwired: 6 in, 1 out]
                  }
                  frame #1 {
                    # "Adds Headers if they don't exist"
                    n928 = local read "Transfer Folder"() -> (w2254:path)
                    n929 = Concatenate Strings("Stats\\", "Tranformer Data.txt") -> (w2255:string)
                    n930 = Build Path(base path=w2254, name or relative path=w2255) -> (appended path=w2248:path)
                    n931 = call-poly <vilib>:"Read From Spreadsheet File.vi"("file path (dialog if empty)"=w2248) -> ("first row"=w2253:string[])  [unwired: 6 in, 4 out]
                    n932 = Search 1D Array(1D array=w2253, element="DeviceID") -> (index of element=w2251:i32)  [unwired: 1 in]
                    n933 = Equal?(x=w2251, y=0) -> (x = y?=w2249:bool)
                    n934 = case shown="False" w2249 {
                      tunnel: w2248 -> [w2259 _]
                      frame False {
                        n935 = local read "Transformer \nHeaders"() -> (w2258:string[])
                        n936 = call-poly <vilib>:"Write To Spreadsheet File.vi"("1D data"=w2258, "file path (dialog if empty)"=w2259) -> ()  [unwired: 6 in, 1 out]
                      }
                      frame True {
                      }
                    }
                  }
                  frame #2 {
                    # "Adds current device if it doesn't exist"
                    n937 = local read "Current \nRecord"() -> (w2264:string[])
                    n938 = Index Array(array=w2264, index=0) -> (element=w2263:string)
                    n939 = local read "Transfer Folder"() -> (w2267:path)
                    n940 = Concatenate Strings("Stats\\", "Tranformer Data.txt") -> (w2268:string)
                    n941 = local write "Current Device ID"(w2263) -> ()
                    n942 = local read "Current Device ID"() -> (w2273:string)
                    n943 = Build Path(base path=w2267, name or relative path=w2268) -> (appended path=w2266:path)
                    n944 = call-poly <vilib>:"Read From Spreadsheet File.vi"("file path (dialog if empty)"=w2266) -> ("all rows"=w2260:string[][])  [unwired: 6 in, 4 out]
                    n945 = Index Array(array=w2260, index (col)=0) -> (element=w2261:string[])  [unwired: 1 in]
                    n946 = Search 1D Array(1D array=w2261, element=w2273) -> (index of element=w2262:i32)  [unwired: 1 in]
                    n947 = Equal?(x=w2262, y=-1) -> (x = y?=w2275:bool)
                    n948 = case shown="False" w2275 {
                      tunnel: w2265 -> [w2278 w2289]
                      tunnel: w2262 -> [w2281 _]
                      tunnel: w2260 -> [w2282 _]
                      frame False {
                        n949 = local read "Current \nRecord"() -> (w2280:string[])
                        n950 = Replace Array Subset(array=w2282, new element=w2280, index (row)=w2281) -> (w2279:string[][])  [unwired: 1 in]
                        n951 = flat-sequence {
                          tunnel: w2278 -> [w2283]
                          tunnel: w2279 -> [w2284]
                          tunnel: [w2284] -> w2277
                          tunnel: [w2283] -> w2276
                          tunnel: w2277 -> [w2286]
                          tunnel: w2276 -> [w2285]
                          frame #0 {
                            n952 = Delete(path (use dialog)=w2283) -> ()  [unwired: 4 in, 3 out]
                          }
                          frame #1 {
                            n953 = call-poly <vilib>:"Write To Spreadsheet File.vi"("append to file? (new file:F)"=TRUE, "2D data"=w2286, "file path (dialog if empty)"=w2285) -> ()  [unwired: 5 in, 1 out]
                          }
                        }
                      }
                      frame True {
                        n954 = local read "Current \nRecord"() -> (w2288:string[])
                        n955 = call-poly <vilib>:"Write To Spreadsheet File.vi"("append to file? (new file:F)"=TRUE, "1D data"=w2288, "file path (dialog if empty)"=w2289) -> ()  [unwired: 5 in, 1 out]
                      }
                    }
                  }
                }
                n956 = Path To String(path=w1775) -> (string=w1773:string)
                n957 = stacked-sequence {
                  tunnel: [_ _ _ _ _ _ _ _ _ _ _ _ _ w2208] -> w1755
                  tunnel: w1754 -> [w1777 _ _ _ _ _ _ _ _ _ _ _ _ _]
                  frame #0 {
                    n958 = call-poly <vilib>:"Read From Spreadsheet File.vi"("file path (dialog if empty)"=w1777) -> ("all rows"=w1776:string[][])  [unwired: 6 in, 4 out]
                    n959 = Array Size(array=w1776) -> (size(s)=w1781:i32[])
                    n960 = Array Subset(array=w1776, index (row)=0, index (col)=0, length (col)=3) -> (w1785:string[][])  [unwired: 1 in]
                    n961 = Index Array(array=w1781, index=0) -> (element=w1779:i32)
                    n962 = Reshape Array(w1785, w1779) -> (w1778:string[])
                    n963 = Search 1D Array(1D array=w1778, element="Dielectric (nm):") -> (index of element=w1788:i32)  [unwired: 1 in]
                    n964 = Equal?(x=w1788, y=-1) -> (x = y?=w1787:bool)
                    n965 = case shown="False" w1787 {
                      tunnel: w1776 -> [w1796 w1800]
                      tunnel: w1788 -> [w1792 _]
                      tunnel: [w1791 w1800] -> w1786
                      frame False {
                        n966 = local read "New: Dielectric"() -> (w1798:dbl)
                        n967 = Number To Fractional String(number=w1798) -> (F-format string=w1793:string)  [unwired: 3 in]
                        n968 = Divide(x=w1792, y=3) -> (x/y=w1795:dbl)
                        n969 = To Word Integer(number=w1795) -> (16bit integer=w1794:i16)
                        n970 = Replace Array Subset(array=w1796, new element=w1793, index (row)=w1794, index (col)=1) -> (w1791:string[][])
                      }
                      frame True {
                      }
                    }
                    n971 = local write "Save1 Array"(w1786) -> ()
                  }
                  frame #1 {
                    n972 = local read "Save1 Array"() -> (w1802:string[][])
                    n973 = Array Size(array=w1802) -> (size(s)=w1805:i32[])
                    n974 = Array Subset(array=w1802, index (row)=0, index (col)=0, length (col)=3) -> (w1809:string[][])  [unwired: 1 in]
                    n975 = Index Array(array=w1805, index=0) -> (element=w1803:i32)
                    n976 = Reshape Array(w1809, w1803) -> (w1801:string[])
                    n977 = Search 1D Array(1D array=w1801, element="Comments:") -> (index of element=w1812:i32)  [unwired: 1 in]
                    n978 = Equal?(x=w1812, y=-1) -> (x = y?=w1811:bool)
                    n979 = case shown="False" w1811 {
                      tunnel: w1802 -> [w1820 w1823]
                      tunnel: w1812 -> [w1817 _]
                      tunnel: [w1816 w1823] -> w1810
                      frame False {
                        n980 = local read "Comments:"() -> (w1815:string)
                        n981 = Divide(x=w1817, y=3) -> (x/y=w1819:dbl)
                        n982 = To Word Integer(number=w1819) -> (16bit integer=w1818:i16)
                        n983 = Replace Array Subset(array=w1820, new element=w1815, index (row)=w1818, index (col)=1) -> (w1816:string[][])
                      }
                      frame True {
                      }
                    }
                    n984 = local write "Save1 Array"(w1810) -> ()
                  }
                  frame #2 {
                    n985 = local read "Save1 Array"() -> (w1825:string[][])
                    n986 = Array Size(array=w1825) -> (size(s)=w1828:i32[])
                    n987 = Array Subset(array=w1825, index (row)=0, index (col)=0, length (col)=3) -> (w1832:string[][])  [unwired: 1 in]
                    n988 = Index Array(array=w1828, index=0) -> (element=w1826:i32)
                    n989 = Reshape Array(w1832, w1826) -> (w1824:string[])
                    n990 = Search 1D Array(1D array=w1824, element="Length (um):") -> (index of element=w1835:i32)  [unwired: 1 in]
                    n991 = Equal?(x=w1835, y=-1) -> (x = y?=w1834:bool)
                    n992 = case shown="False" w1834 {
                      tunnel: w1825 -> [w1845 w1848]
                      tunnel: w1835 -> [w1842 _]
                      tunnel: [w1841 w1848] -> w1833
                      frame False {
                        n993 = local read "New: Length"() -> (w1838:dbl)
                        n994 = Divide(x=w1842, y=3) -> (x/y=w1844:dbl)
                        n995 = Format Value(format string="%#g", value (0)=w1838) -> (output string=w1839:string)  [unwired: 1 in]
                        n996 = To Word Integer(number=w1844) -> (16bit integer=w1843:i16)
                        n997 = Replace Array Subset(array=w1845, new element=w1839, index (row)=w1843, index (col)=1) -> (w1841:string[][])
                      }
                      frame True {
                      }
                    }
                    n998 = local write "Save1 Array"(w1833) -> ()
                  }
                  frame #3 {
                    n999 = local read "Save1 Array"() -> (w1850:string[][])
                    n1000 = Array Size(array=w1850) -> (size(s)=w1855:i32[])
                    n1001 = Array Subset(array=w1850, index (row)=0, index (col)=0, length (col)=3) -> (w1851:string[][])  [unwired: 1 in]
                    n1002 = Index Array(array=w1855, index=0) -> (element=w1857:i32)
                    n1003 = Reshape Array(w1851, w1857) -> (w1849:string[])
                    n1004 = Search 1D Array(1D array=w1849, element="Width (um):") -> (index of element=w1860:i32)  [unwired: 1 in]
                    n1005 = Equal?(x=w1860, y=-1) -> (x = y?=w1859:bool)
                    n1006 = case shown="False" w1859 {
                      tunnel: w1860 -> [w1868 _]
                      tunnel: w1850 -> [w1867 w1873]
                      tunnel: [w1866 w1873] -> w1858
                      frame False {
                        n1007 = local read "New: Width"() -> (w1863:dbl)
                        n1008 = Divide(x=w1868, y=3) -> (x/y=w1870:dbl)
                        n1009 = To Word Integer(number=w1870) -> (16bit integer=w1869:i16)
                        n1010 = Format Value(format string="%#g", value (0)=w1863) -> (output string=w1864:string)  [unwired: 1 in]
                        n1011 = Replace Array Subset(array=w1867, new element=w1864, index (row)=w1869, index (col)=1) -> (w1866:string[][])
                      }
                      frame True {
                      }
                    }
                    n1012 = local write "Save1 Array"(w1858) -> ()
                  }
                  frame #4 {
                    w1883 = "Sample Temp (K):"
                    n1013 = local read "Save1 Array"() -> (w1875:string[][])
                    n1014 = Array Size(array=w1875) -> (size(s)=w1880:i32[])
                    n1015 = Array Subset(array=w1875, index (row)=0, index (col)=0, length (col)=3) -> (w1876:string[][])  [unwired: 1 in]
                    n1016 = Index Array(array=w1880, index=0) -> (element=w1882:i32)
                    n1017 = Reshape Array(w1876, w1882) -> (w1874:string[])
                    n1018 = Search 1D Array(1D array=w1874, element=w1883) -> (index of element=w1886:i32)  [unwired: 1 in]
                    n1019 = Equal?(x=w1886, y=-1) -> (x = y?=w1885:bool)
                    n1020 = case shown="True" w1885 {
                      tunnel: w1875 -> [w1895 w1909]
                      tunnel: w1886 -> [w1892 _]
                      tunnel: [w1891 w1908] -> w1884
                      tunnel: w1874 -> [_ w1911]
                      tunnel: w1883 -> [_ w1898]
                      frame False {
                        n1021 = local read "New: Temp"() -> (w1889:dbl)
                        n1022 = Divide(x=w1892, y=3) -> (x/y=w1894:dbl)
                        n1023 = Format Value(format string="%#g", value (0)=w1889) -> (output string=w1888:string)  [unwired: 1 in]
                        n1024 = To Word Integer(number=w1894) -> (16bit integer=w1893:i16)
                        n1025 = Replace Array Subset(array=w1895, new element=w1888, index (row)=w1893, index (col)=1) -> (w1891:string[][])
                      }
                      frame True {
                        n1026 = local read "New: Temp"() -> (w1900:dbl)
                        n1027 = Search 1D Array(1D array=w1911, element="Width (um):") -> (index of element=w1905:i32)  [unwired: 1 in]
                        n1028 = Divide(x=w1905, y=3) -> (x/y=w1906:dbl)
                        n1029 = To Word Integer(number=w1906) -> (16bit integer=w1904:i16)
                        n1030 = Format Value(format string="%#g", value (0)=w1900) -> (output string=w1899:string)  [unwired: 1 in]
                        n1031 = Build Array(w1898, w1899) -> (w1902:string[])
                        n1032 = Increment(x=w1904) -> (x+1=w1903:i16)
                        n1033 = Insert Into Array(array=w1909, index (row)=w1903, new element=w1902) -> (w1908:string[][])  [unwired: 1 in]
                      }
                    }
                    n1034 = local write "Save1 Array"(w1884) -> ()
                  }
                  frame #5 {
                    w1921 = "Mobility-Sat (cm^2/Vs):"
                    n1035 = local read "Save1 Array"() -> (w1913:string[][])
                    n1036 = Array Size(array=w1913) -> (size(s)=w1918:i32[])
                    n1037 = Array Subset(array=w1913, index (row)=0, index (col)=0, length (col)=3) -> (w1914:string[][])  [unwired: 1 in]
                    n1038 = Index Array(array=w1918, index=0) -> (element=w1920:i32)
                    n1039 = Reshape Array(w1914, w1920) -> (w1912:string[])
                    n1040 = Search 1D Array(1D array=w1912, element=w1921) -> (index of element=w1924:i32)  [unwired: 1 in]
                    n1041 = Equal?(x=w1924, y=-1) -> (x = y?=w1923:bool)
                    n1042 = case shown="True" w1923 {
                      tunnel: w1913 -> [w1933 w1941]
                      tunnel: w1924 -> [w1930 _]
                      tunnel: [w1929 w1940] -> w1922
                      tunnel: w1912 -> [_ w1938]
                      tunnel: w1921 -> [_ w1936]
                      frame False {
                        n1043 = local read "New: Mobility-Sat"() -> (w1926:dbl)
                        n1044 = Divide(x=w1930, y=3) -> (x/y=w1932:dbl)
                        n1045 = To Word Integer(number=w1932) -> (16bit integer=w1931:i16)
                        n1046 = Format Value(format string="%#g", value (0)=w1926) -> (output string=w1927:string)  [unwired: 1 in]
                        n1047 = Replace Array Subset(array=w1933, new element=w1927, index (row)=w1931, index (col)=1) -> (w1929:string[][])
                      }
                      frame True {
                        n1048 = local read "New: Mobility-Sat"() -> (w1942:dbl)
                        n1049 = Search 1D Array(1D array=w1938, element="Mobility (cm^2/Vs):") -> (index of element=w1945:i32)  [unwired: 1 in]
                        n1050 = Divide(x=w1945, y=3) -> (x/y=w1946:dbl)
                        n1051 = To Word Integer(number=w1946) -> (16bit integer=w1937:i16)
                        n1052 = Format Value(format string="%#g", value (0)=w1942) -> (output string=w1939:string)  [unwired: 1 in]
                        n1053 = Build Array(w1936, w1939) -> (w1944:string[])
                        n1054 = Replace Array Subset(array=w1941, new element=w1944, index (row)=w1937) -> (w1940:string[][])  [unwired: 1 in]
                      }
                    }
                    n1055 = local write "Save1 Array"(w1922) -> ()
                  }
                  frame #6 {
                    w1958 = "Mobility-Lin (cm^2/Vs):"
                    n1056 = local read "Save1 Array"() -> (w1949:string[][])
                    n1057 = Array Size(array=w1949) -> (size(s)=w1955:i32[])
                    n1058 = Array Subset(array=w1949, index (row)=0, index (col)=0, length (col)=3) -> (w1951:string[][])  [unwired: 1 in]
                    n1059 = Index Array(array=w1955, index=0) -> (element=w1957:i32)
                    n1060 = Reshape Array(w1951, w1957) -> (w1950:string[])
                    n1061 = Search 1D Array(1D array=w1950, element=w1958) -> (index of element=w1961:i32)  [unwired: 1 in]
                    n1062 = Equal?(x=w1961, y=-1) -> (x = y?=w1960:bool)
                    n1063 = case shown="True" w1960 {
                      tunnel: w1949 -> [w1970 w1976]
                      tunnel: w1961 -> [w1967 _]
                      tunnel: [w1966 w1975] -> w1959
                      tunnel: w1950 -> [_ w1974]
                      tunnel: w1958 -> [_ w1973]
                      frame False {
                        n1064 = local read "Calc: Mobility-Lin"() -> (w1963:dbl)
                        n1065 = Divide(x=w1967, y=3) -> (x/y=w1969:dbl)
                        n1066 = To Word Integer(number=w1969) -> (16bit integer=w1968:i16)
                        n1067 = Format Value(format string="%#g", value (0)=w1963) -> (output string=w1964:string)  [unwired: 1 in]
                        n1068 = Replace Array Subset(array=w1970, new element=w1964, index (row)=w1968, index (col)=1) -> (w1966:string[][])
                      }
                      frame True {
                        n1069 = local read "Calc: Mobility-Lin"() -> (w1977:dbl)
                        n1070 = Search 1D Array(1D array=w1974, element="Mobility-Sat (cm^2/Vs):") -> (index of element=w1982:i32)  [unwired: 1 in]
                        n1071 = Divide(x=w1982, y=3) -> (x/y=w1983:dbl)
                        n1072 = To Word Integer(number=w1983) -> (16bit integer=w1981:i16)
                        n1073 = Format Value(format string="%#g", value (0)=w1977) -> (output string=w1986:string)  [unwired: 1 in]
                        n1074 = Build Array(w1973, w1986) -> (w1979:string[])
                        n1075 = Increment(x=w1981) -> (x+1=w1980:i16)
                        n1076 = Insert Into Array(array=w1976, index (row)=w1980, new element=w1979) -> (w1975:string[][])  [unwired: 1 in]
                      }
                    }
                    n1077 = local write "Save1 Array"(w1959) -> ()
                  }
                  frame #7 {
                    w1996 = "On/Off I-Sat:"
                    n1078 = local read "Save1 Array"() -> (w1987:string[][])
                    n1079 = Array Size(array=w1987) -> (size(s)=w1993:i32[])
                    n1080 = Array Subset(array=w1987, index (row)=0, index (col)=0, length (col)=3) -> (w1989:string[][])  [unwired: 1 in]
                    n1081 = Index Array(array=w1993, index=0) -> (element=w1995:i32)
                    n1082 = Reshape Array(w1989, w1995) -> (w1988:string[])
                    n1083 = Search 1D Array(1D array=w1988, element=w1996) -> (index of element=w1999:i32)  [unwired: 1 in]
                    n1084 = Equal?(x=w1999, y=-1) -> (x = y?=w1998:bool)
                    n1085 = case shown="True" w1998 {
                      tunnel: w1987 -> [w2008 w2015]
                      tunnel: w1999 -> [w2005 _]
                      tunnel: [w2004 w2016] -> w1997
                      tunnel: w1988 -> [_ w2013]
                      tunnel: w1996 -> [_ w2011]
                      frame False {
                        n1086 = local read "Calc: On/Off"() -> (w2001:dbl)
                        n1087 = Divide(x=w2005, y=3) -> (x/y=w2007:dbl)
                        n1088 = To Word Integer(number=w2007) -> (16bit integer=w2006:i16)
                        n1089 = Format Value(format string="%#g", value (0)=w2001) -> (output string=w2002:string)  [unwired: 1 in]
                        n1090 = Replace Array Subset(array=w2008, new element=w2002, index (row)=w2006, index (col)=1) -> (w2004:string[][])
                      }
                      frame True {
                        n1091 = local read "Calc: On/Off"() -> (w2017:dbl)
                        n1092 = Search 1D Array(1D array=w2013, element="On/Off Current:") -> (index of element=w2020:i32)  [unwired: 1 in]
                        n1093 = Divide(x=w2020, y=3) -> (x/y=w2021:dbl)
                        n1094 = To Word Integer(number=w2021) -> (16bit integer=w2012:i16)
                        n1095 = Format Value(format string="%#g", value (0)=w2017) -> (output string=w2014:string)  [unwired: 1 in]
                        n1096 = Build Array(w2011, w2014) -> (w2019:string[])
                        n1097 = Replace Array Subset(array=w2015, new element=w2019, index (row)=w2012) -> (w2016:string[][])  [unwired: 1 in]
                      }
                    }
                    n1098 = local write "Save1 Array"(w1997) -> ()
                  }
                  frame #8 {
                    w2033 = "Off I-Sat (A):"
                    n1099 = local read "Save1 Array"() -> (w2024:string[][])
                    n1100 = Array Size(array=w2024) -> (size(s)=w2030:i32[])
                    n1101 = Array Subset(array=w2024, index (row)=0, index (col)=0, length (col)=3) -> (w2026:string[][])  [unwired: 1 in]
                    n1102 = Index Array(array=w2030, index=0) -> (element=w2032:i32)
                    n1103 = Reshape Array(w2026, w2032) -> (w2025:string[])
                    n1104 = Search 1D Array(1D array=w2025, element=w2033) -> (index of element=w2036:i32)  [unwired: 1 in]
                    n1105 = Equal?(x=w2036, y=-1) -> (x = y?=w2035:bool)
                    n1106 = case shown="True" w2035 {
                      tunnel: w2024 -> [w2045 w2051]
                      tunnel: w2036 -> [w2042 _]
                      tunnel: [w2041 w2050] -> w2034
                      tunnel: w2025 -> [_ w2049]
                      tunnel: w2033 -> [_ w2048]
                      frame False {
                        n1107 = local read "Calc: Off I-Sat"() -> (w2040:dbl)
                        n1108 = Divide(x=w2042, y=3) -> (x/y=w2044:dbl)
                        n1109 = Format Value(format string="%#g", value (0)=w2040) -> (output string=w2038:string)  [unwired: 1 in]
                        n1110 = To Word Integer(number=w2044) -> (16bit integer=w2043:i16)
                        n1111 = Replace Array Subset(array=w2045, new element=w2038, index (row)=w2043, index (col)=1) -> (w2041:string[][])
                      }
                      frame True {
                        n1112 = local read "Calc: Off I-Sat"() -> (w2052:dbl)
                        n1113 = Search 1D Array(1D array=w2049, element="On/Off I-Sat:") -> (index of element=w2057:i32)  [unwired: 1 in]
                        n1114 = Divide(x=w2057, y=3) -> (x/y=w2058:dbl)
                        n1115 = To Word Integer(number=w2058) -> (16bit integer=w2056:i16)
                        n1116 = Format Value(format string="%#g", value (0)=w2052) -> (output string=w2061:string)  [unwired: 1 in]
                        n1117 = Build Array(w2048, w2061) -> (w2054:string[])
                        n1118 = Increment(x=w2056) -> (x+1=w2055:i16)
                        n1119 = Insert Into Array(array=w2051, index (row)=w2055, new element=w2054) -> (w2050:string[][])  [unwired: 1 in]
                      }
                    }
                    n1120 = local write "Save1 Array"(w2034) -> ()
                  }
                  frame #9 {
                    w2063 = "Vt-Sat (V):"
                    n1121 = local read "Save1 Array"() -> (w2064:string[][])
                    n1122 = Array Size(array=w2064) -> (size(s)=w2069:i32[])
                    n1123 = Array Subset(array=w2064, index (row)=0, index (col)=0, length (col)=3) -> (w2065:string[][])  [unwired: 1 in]
                    n1124 = Index Array(array=w2069, index=0) -> (element=w2071:i32)
                    n1125 = Reshape Array(w2065, w2071) -> (w2062:string[])
                    n1126 = Search 1D Array(1D array=w2062, element=w2063) -> (index of element=w2074:i32)  [unwired: 1 in]
                    n1127 = Equal?(x=w2074, y=-1) -> (x = y?=w2073:bool)
                    n1128 = case shown="True" w2073 {
                      tunnel: w2064 -> [w2081 w2090]
                      tunnel: w2074 -> [w2077 _]
                      tunnel: [w2076 w2089] -> w2072
                      tunnel: w2063 -> [_ w2088]
                      tunnel: w2062 -> [_ w2087]
                      frame False {
                        n1129 = local read "New: VT-Sat"() -> (w2083:dbl)
                        n1130 = Number To Fractional String(number=w2083) -> (F-format string=w2078:string)  [unwired: 3 in]
                        n1131 = Divide(x=w2077, y=3) -> (x/y=w2080:dbl)
                        n1132 = To Word Integer(number=w2080) -> (16bit integer=w2079:i16)
                        n1133 = Replace Array Subset(array=w2081, new element=w2078, index (row)=w2079, index (col)=1) -> (w2076:string[][])
                      }
                      frame True {
                        n1134 = local read "New: VT-Sat"() -> (w2091:dbl)
                        n1135 = Search 1D Array(1D array=w2087, element="Threshold V (V):") -> (index of element=w2086:i32)  [unwired: 1 in]
                        n1136 = Divide(x=w2086, y=3) -> (x/y=w2094:dbl)
                        n1137 = To Word Integer(number=w2094) -> (16bit integer=w2085:i16)
                        n1138 = Format Value(format string="%#g", value (0)=w2091) -> (output string=w2097:string)  [unwired: 1 in]
                        n1139 = Build Array(w2088, w2097) -> (w2093:string[])
                        n1140 = Replace Array Subset(array=w2090, new element=w2093, index (row)=w2085) -> (w2089:string[][])  [unwired: 1 in]
                      }
                    }
                    n1141 = local write "Save1 Array"(w2072) -> ()
                  }
                  frame #10 {
                    n1142 = local read "Save1 Array"() -> (w2098:string[][])
                    n1143 = Array Size(array=w2098) -> (size(s)=w2104:i32[])
                    n1144 = Array Subset(array=w2098, index (row)=0, index (col)=0, length (col)=3) -> (w2100:string[][])  [unwired: 1 in]
                    n1145 = Index Array(array=w2104, index=0) -> (element=w2106:i32)
                    n1146 = Reshape Array(w2100, w2106) -> (w2099:string[])
                    n1147 = Search 1D Array(1D array=w2099, element="VT-Lin (V):") -> (index of element=w2109:i32)  [unwired: 1 in]
                    n1148 = Equal?(x=w2109, y=-1) -> (x = y?=w2108:bool)
                    n1149 = case shown="False" w2108 {
                      tunnel: w2098 -> [w2119 w2122]
                      tunnel: w2109 -> [w2116 _]
                      tunnel: [w2115 w2122] -> w2107
                      frame False {
                        n1150 = local read "New: VT-Lin"() -> (w2113:dbl)
                        n1151 = Divide(x=w2116, y=3) -> (x/y=w2118:dbl)
                        n1152 = Format Value(format string="%#g", value (0)=w2113) -> (output string=w2112:string)  [unwired: 1 in]
                        n1153 = To Word Integer(number=w2118) -> (16bit integer=w2117:i16)
                        n1154 = Replace Array Subset(array=w2119, new element=w2112, index (row)=w2117, index (col)=1) -> (w2115:string[][])
                      }
                      frame True {
                      }
                    }
                    n1155 = local write "Save1 Array"(w2107) -> ()
                  }
                  frame #11 {
                    w2123 = "STS-Sat (V/decade):"
                    n1156 = local read "Save1 Array"() -> (w2125:string[][])
                    n1157 = Array Size(array=w2125) -> (size(s)=w2130:i32[])
                    n1158 = Array Subset(array=w2125, index (row)=0, index (col)=0, length (col)=3) -> (w2126:string[][])  [unwired: 1 in]
                    n1159 = Index Array(array=w2130, index=0) -> (element=w2132:i32)
                    n1160 = Reshape Array(w2126, w2132) -> (w2124:string[])
                    n1161 = Search 1D Array(1D array=w2124, element=w2123) -> (index of element=w2135:i32)  [unwired: 1 in]
                    n1162 = Equal?(x=w2135, y=-1) -> (x = y?=w2134:bool)
                    n1163 = case shown="True" w2134 {
                      tunnel: w2125 -> [w2144 w2150]
                      tunnel: w2135 -> [w2141 _]
                      tunnel: [w2140 w2151] -> w2133
                      tunnel: w2124 -> [_ w2149]
                      tunnel: w2123 -> [_ w2148]
                      frame False {
                        n1164 = local read "New: STS"() -> (w2138:dbl)
                        n1165 = Divide(x=w2141, y=3) -> (x/y=w2143:dbl)
                        n1166 = Format Value(format string="%#g", value (0)=w2138) -> (output string=w2137:string)  [unwired: 1 in]
                        n1167 = To Word Integer(number=w2143) -> (16bit integer=w2142:i16)
                        n1168 = Replace Array Subset(array=w2144, new element=w2137, index (row)=w2142, index (col)=1) -> (w2140:string[][])
                      }
                      frame True {
                        n1169 = local read "New: STS"() -> (w2152:dbl)
                        n1170 = Search 1D Array(1D array=w2149, element="S.T.S. (V/decade):") -> (index of element=w2155:i32)  [unwired: 1 in]
                        n1171 = Divide(x=w2155, y=3) -> (x/y=w2156:dbl)
                        n1172 = To Word Integer(number=w2156) -> (16bit integer=w2147:i16)
                        n1173 = Format Value(format string="%#g", value (0)=w2152) -> (output string=w2159:string)  [unwired: 1 in]
                        n1174 = Build Array(w2148, w2159) -> (w2154:string[])
                        n1175 = Replace Array Subset(array=w2150, new element=w2154, index (row)=w2147) -> (w2151:string[][])  [unwired: 1 in]
                      }
                    }
                    n1176 = local write "Save1 Array"(w2133) -> ()
                  }
                  frame #12 {
                    w2160 = "Trap Density-VT (Traps/Vcm^2):"
                    n1177 = local read "Save1 Array"() -> (w2162:string[][])
                    n1178 = Array Size(array=w2162) -> (size(s)=w2167:i32[])
                    n1179 = Array Subset(array=w2162, index (row)=0, index (col)=0, length (col)=3) -> (w2163:string[][])  [unwired: 1 in]
                    n1180 = Index Array(array=w2167, index=0) -> (element=w2169:i32)
                    n1181 = Reshape Array(w2163, w2169) -> (w2161:string[])
                    n1182 = Search 1D Array(1D array=w2161, element=w2160) -> (index of element=w2172:i32)  [unwired: 1 in]
                    n1183 = Equal?(x=w2172, y=-1) -> (x = y?=w2171:bool)
                    n1184 = case shown="True" w2171 {
                      tunnel: w2162 -> [w2181 w2186]
                      tunnel: w2172 -> [w2177 _]
                      tunnel: [w2176 w2187] -> w2170
                      tunnel: w2161 -> [_ w2185]
                      tunnel: w2160 -> [_ w2184]
                      frame False {
                        n1185 = local read "New: Trap Density-VT"() -> (w2175:dbl)
                        n1186 = Format Value(format string="%#g", value (0)=w2175) -> (output string=w2178:string)  [unwired: 1 in]
                        n1187 = Divide(x=w2177, y=3) -> (x/y=w2180:dbl)
                        n1188 = To Word Integer(number=w2180) -> (16bit integer=w2179:i16)
                        n1189 = Replace Array Subset(array=w2181, new element=w2178, index (row)=w2179, index (col)=1) -> (w2176:string[][])
                      }
                      frame True {
                        n1190 = local read "New: Trap Density-VT"() -> (w2197:dbl)
                        n1191 = Search 1D Array(1D array=w2185, element="STS-Sat (V/decade):") -> (index of element=w2192:i32)  [unwired: 1 in]
                        n1192 = Divide(x=w2192, y=3) -> (x/y=w2191:dbl)
                        n1193 = To Word Integer(number=w2191) -> (16bit integer=w2193:i16)
                        n1194 = Format Value(format string="%#g", value (0)=w2197) -> (output string=w2188:string)  [unwired: 1 in]
                        n1195 = Build Array(w2184, w2188) -> (w2195:string[])
                        n1196 = Increment(x=w2193) -> (x+1=w2194:i16)
                        n1197 = Insert Into Array(array=w2186, index (row)=w2194, new element=w2195) -> (w2187:string[][])  [unwired: 1 in]
                      }
                    }
                    n1198 = local write "Save1 Array"(w2170) -> ()
                  }
                  frame #13 {
                    w2198 = "Trap Density-STS (Traps/Vcm^2):"
                    n1199 = local read "Save1 Array"() -> (w2200:string[][])
                    n1200 = Array Size(array=w2200) -> (size(s)=w2205:i32[])
                    n1201 = Array Subset(array=w2200, index (row)=0, index (col)=0, length (col)=3) -> (w2201:string[][])  [unwired: 1 in]
                    n1202 = Index Array(array=w2205, index=0) -> (element=w2207:i32)
                    n1203 = Reshape Array(w2201, w2207) -> (w2199:string[])
                    n1204 = Search 1D Array(1D array=w2199, element=w2198) -> (index of element=w2210:i32)  [unwired: 1 in]
                    n1205 = Equal?(x=w2210, y=-1) -> (x = y?=w2209:bool)
                    n1206 = case shown="True" w2209 {
                      tunnel: w2200 -> [w2219 w2224]
                      tunnel: w2210 -> [w2216 _]
                      tunnel: [w2215 w2225] -> w2208
                      tunnel: w2199 -> [_ w2223]
                      tunnel: w2198 -> [_ w2222]
                      frame False {
                        n1207 = local read "New: Trap Density-STS"() -> (w2213:dbl)
                        n1208 = Divide(x=w2216, y=3) -> (x/y=w2218:dbl)
                        n1209 = To Word Integer(number=w2218) -> (16bit integer=w2217:i16)
                        n1210 = Format Value(format string="%#g", value (0)=w2213) -> (output string=w2212:string)  [unwired: 1 in]
                        n1211 = Replace Array Subset(array=w2219, new element=w2212, index (row)=w2217, index (col)=1) -> (w2215:string[][])
                      }
                      frame True {
                        n1212 = local read "New: Trap Density-STS"() -> (w2226:dbl)
                        n1213 = Search 1D Array(1D array=w2223, element="Trap Density-VT (Traps/Vcm^2):") -> (index of element=w2231:i32)  [unwired: 1 in]
                        n1214 = Divide(x=w2231, y=3) -> (x/y=w2232:dbl)
                        n1215 = To Word Integer(number=w2232) -> (16bit integer=w2230:i16)
                        n1216 = Format Value(format string="%#g", value (0)=w2226) -> (output string=w2235:string)  [unwired: 1 in]
                        n1217 = Build Array(w2222, w2235) -> (w2228:string[])
                        n1218 = Increment(x=w2230) -> (x+1=w2229:i16)
                        n1219 = Insert Into Array(array=w2224, index (row)=w2229, new element=w2228) -> (w2225:string[][])  [unwired: 1 in]
                      }
                    }
                    n1220 = local write "Save1 Array"(w2208) -> ()
                  }
                }
                n1221 = Concatenate Strings(w1773, "\\", w1771) -> (w1772:string)
                n1222 = String To Path(string=w1772) -> (path=w1762:path)
                n1223 = disable-structure shown="Disabled" {
                  frame Disabled {
                  }
                  frame Enabled {
                  }
                }
              }
              frame #2 {
                n1224 = Equal?(x=w2294, y=w2291) -> (x = y?=w2293:bool)
                n1225 = case shown="False" w2293 {
                  tunnel: w2294 -> [w2297 _]
                  tunnel: w2291 -> [w2296 _]
                  frame False {
                    n1226 = Move(source path=w2297, 9:TRUE, 10:w2296) -> ()  [unwired: 2 in, 3 out]
                  }
                  frame True {
                  }
                }
              }
              frame #3 {
                n1227 = local write "Transfer File"(w2298) -> ()
                n1228 = call-poly <vilib>:"Write To Spreadsheet File.vi"("2D data"=w2299, "file path (dialog if empty)"=w2298) -> ()  [unwired: 6 in, 1 out]
              }
            }
          }
          event "Save Changes? 2": Mouse Down {
            n1229 = event-data() -> ()  [unwired: 1 in, 5 out]
            n1230 = stacked-sequence {
              seq-local: [w2357 _ _ _ _] -> [_ w2840 _ _ _]
              seq-local: [w2356 _ _ _ _] -> [_ w2841 _ _ _]
              seq-local: [w2356 _ _ _ _] -> [_ w2839 _ _ _]
              seq-local: [w2358 _ _ _ _] -> [_ w2837 _ _ _]
              seq-local: [_ w2841 _ _ _] -> [_ _ w2846 _ _]
              seq-local: [_ w2837 _ _ _] -> [_ _ w2845 _ _]
              frame #0 {
                n1231 = local read "Transfer File"() -> (w2357:path)
                n1232 = local read "New: Temp"() -> (w2360:dbl)
                n1233 = local read "New: Length"() -> (w2363:dbl)
                n1234 = local read "New: Width"() -> (w2361:dbl)
                n1235 = To Word Integer(number=w2360) -> (16bit integer=w2359:i16)
                n1236 = Number To Decimal String(number=w2359) -> (decimal integer string=w2367:string)  [unwired: 1 in]
                n1237 = To Single Precision Float(number=w2361) -> (single precision float=w2362:sgl)
                n1238 = To Single Precision Float(number=w2363) -> (single precision float=w2364:sgl)
                n1239 = local read "Index"() -> (w2371:string)
                n1240 = Strip Path(path=w2357) -> (stripped path=w2376:path)  [unwired: 1 out]
                n1241 = Number To Decimal String(number=w2364) -> (decimal integer string=w2369:string)  [unwired: 1 in]
                n1242 = Number To Decimal String(number=w2362) -> (decimal integer string=w2370:string)  [unwired: 1 in]
                n1243 = Concatenate Strings("_", w2367, "K") -> (w2365:string)
                n1244 = call "Build Text2"("Temp"=w2365, "Index"=w2371, "Length"=w2369, "Width"=w2370) -> ("Result"=w2372:string)  [unwired: 10 in, 1 out]
                n1245 = Path To String(path=w2376) -> (string=w2374:string)
                n1246 = Concatenate Strings(w2374, "\\", w2372) -> (w2373:string)
                n1247 = stacked-sequence {
                  tunnel: [_ _ _ _ _ _ _ _ _ _ _ _ _ w2799] -> _
                  tunnel: w2357 -> [w2378 _ _ _ _ _ _ _ _ _ _ _ _ _]
                  tunnel: [_ _ _ _ _ _ _ _ _ _ _ _ _ w2799] -> w2358
                  frame #0 {
                    n1248 = call-poly <vilib>:"Read From Spreadsheet File.vi"("file path (dialog if empty)"=w2378) -> ("all rows"=w2377:string[][])  [unwired: 6 in, 4 out]
                    n1249 = Array Size(array=w2377) -> (size(s)=w2382:i32[])
                    n1250 = Array Subset(array=w2377, index (row)=0, index (col)=0, length (col)=3) -> (w2386:string[][])  [unwired: 1 in]
                    n1251 = Index Array(array=w2382, index=0) -> (element=w2380:i32)
                    n1252 = Reshape Array(w2386, w2380) -> (w2379:string[])
                    n1253 = Search 1D Array(1D array=w2379, element="Dielectric (nm):") -> (index of element=w2389:i32)  [unwired: 1 in]
                    n1254 = Equal?(x=w2389, y=-1) -> (x = y?=w2388:bool)
                    n1255 = case shown="False" w2388 {
                      tunnel: w2377 -> [w2397 w2401]
                      tunnel: w2389 -> [w2393 _]
                      tunnel: [w2392 w2401] -> w2387
                      frame False {
                        n1256 = local read "New: Dielectric"() -> (w2399:dbl)
                        n1257 = Number To Fractional String(number=w2399) -> (F-format string=w2394:string)  [unwired: 3 in]
                        n1258 = Divide(x=w2393, y=3) -> (x/y=w2396:dbl)
                        n1259 = To Word Integer(number=w2396) -> (16bit integer=w2395:i16)
                        n1260 = Replace Array Subset(array=w2397, new element=w2394, index (row)=w2395, index (col)=1) -> (w2392:string[][])
                      }
                      frame True {
                      }
                    }
                    n1261 = local write "Save1 Array"(w2387) -> ()
                  }
                  frame #1 {
                    n1262 = local read "Save1 Array"() -> (w2403:string[][])
                    n1263 = Array Size(array=w2403) -> (size(s)=w2406:i32[])
                    n1264 = Array Subset(array=w2403, index (row)=0, index (col)=0, length (col)=3) -> (w2410:string[][])  [unwired: 1 in]
                    n1265 = Index Array(array=w2406, index=0) -> (element=w2404:i32)
                    n1266 = Reshape Array(w2410, w2404) -> (w2402:string[])
                    n1267 = Search 1D Array(1D array=w2402, element="Comments:") -> (index of element=w2413:i32)  [unwired: 1 in]
                    n1268 = Equal?(x=w2413, y=-1) -> (x = y?=w2412:bool)
                    n1269 = case shown="False" w2412 {
                      tunnel: w2403 -> [w2421 w2424]
                      tunnel: w2413 -> [w2418 _]
                      tunnel: [w2417 w2424] -> w2411
                      frame False {
                        n1270 = local read "Comments:"() -> (w2416:string)
                        n1271 = Divide(x=w2418, y=3) -> (x/y=w2420:dbl)
                        n1272 = To Word Integer(number=w2420) -> (16bit integer=w2419:i16)
                        n1273 = Replace Array Subset(array=w2421, new element=w2416, index (row)=w2419, index (col)=1) -> (w2417:string[][])
                      }
                      frame True {
                      }
                    }
                    n1274 = local write "Save1 Array"(w2411) -> ()
                  }
                  frame #2 {
                    n1275 = local read "Save1 Array"() -> (w2426:string[][])
                    n1276 = Array Size(array=w2426) -> (size(s)=w2429:i32[])
                    n1277 = Array Subset(array=w2426, index (row)=0, index (col)=0, length (col)=3) -> (w2433:string[][])  [unwired: 1 in]
                    n1278 = Index Array(array=w2429, index=0) -> (element=w2427:i32)
                    n1279 = Reshape Array(w2433, w2427) -> (w2425:string[])
                    n1280 = Search 1D Array(1D array=w2425, element="Length (um):") -> (index of element=w2436:i32)  [unwired: 1 in]
                    n1281 = Equal?(x=w2436, y=-1) -> (x = y?=w2435:bool)
                    n1282 = case shown="False" w2435 {
                      tunnel: w2426 -> [w2446 w2449]
                      tunnel: w2436 -> [w2443 _]
                      tunnel: [w2442 w2449] -> w2434
                      frame False {
                        n1283 = local read "New: Length"() -> (w2439:dbl)
                        n1284 = Divide(x=w2443, y=3) -> (x/y=w2445:dbl)
                        n1285 = Format Value(format string="%#g", value (0)=w2439) -> (output string=w2440:string)  [unwired: 1 in]
                        n1286 = To Word Integer(number=w2445) -> (16bit integer=w2444:i16)
                        n1287 = Replace Array Subset(array=w2446, new element=w2440, index (row)=w2444, index (col)=1) -> (w2442:string[][])
                      }
                      frame True {
                      }
                    }
                    n1288 = local write "Save1 Array"(w2434) -> ()
                  }
                  frame #3 {
                    n1289 = local read "Save1 Array"() -> (w2451:string[][])
                    n1290 = Array Size(array=w2451) -> (size(s)=w2456:i32[])
                    n1291 = Array Subset(array=w2451, index (row)=0, index (col)=0, length (col)=3) -> (w2452:string[][])  [unwired: 1 in]
                    n1292 = Index Array(array=w2456, index=0) -> (element=w2458:i32)
                    n1293 = Reshape Array(w2452, w2458) -> (w2450:string[])
                    n1294 = Search 1D Array(1D array=w2450, element="Width (um):") -> (index of element=w2461:i32)  [unwired: 1 in]
                    n1295 = Equal?(x=w2461, y=-1) -> (x = y?=w2460:bool)
                    n1296 = case shown="False" w2460 {
                      tunnel: w2461 -> [w2469 _]
                      tunnel: w2451 -> [w2468 w2474]
                      tunnel: [w2467 w2474] -> w2459
                      frame False {
                        n1297 = local read "New: Width"() -> (w2464:dbl)
                        n1298 = Divide(x=w2469, y=3) -> (x/y=w2471:dbl)
                        n1299 = To Word Integer(number=w2471) -> (16bit integer=w2470:i16)
                        n1300 = Format Value(format string="%#g", value (0)=w2464) -> (output string=w2465:string)  [unwired: 1 in]
                        n1301 = Replace Array Subset(array=w2468, new element=w2465, index (row)=w2470, index (col)=1) -> (w2467:string[][])
                      }
                      frame True {
                      }
                    }
                    n1302 = local write "Save1 Array"(w2459) -> ()
                  }
                  frame #4 {
                    w2484 = "Sample Temp (K):"
                    n1303 = local read "Save1 Array"() -> (w2476:string[][])
                    n1304 = Array Size(array=w2476) -> (size(s)=w2481:i32[])
                    n1305 = Array Subset(array=w2476, index (row)=0, index (col)=0, length (col)=3) -> (w2477:string[][])  [unwired: 1 in]
                    n1306 = Index Array(array=w2481, index=0) -> (element=w2483:i32)
                    n1307 = Reshape Array(w2477, w2483) -> (w2475:string[])
                    n1308 = Search 1D Array(1D array=w2475, element=w2484) -> (index of element=w2487:i32)  [unwired: 1 in]
                    n1309 = Equal?(x=w2487, y=-1) -> (x = y?=w2486:bool)
                    n1310 = case shown="True" w2486 {
                      tunnel: w2476 -> [w2496 w2510]
                      tunnel: w2487 -> [w2493 _]
                      tunnel: [w2492 w2509] -> w2485
                      tunnel: w2475 -> [_ w2512]
                      tunnel: w2484 -> [_ w2499]
                      frame False {
                        n1311 = local read "New: Temp"() -> (w2490:dbl)
                        n1312 = Divide(x=w2493, y=3) -> (x/y=w2495:dbl)
                        n1313 = Format Value(format string="%#g", value (0)=w2490) -> (output string=w2489:string)  [unwired: 1 in]
                        n1314 = To Word Integer(number=w2495) -> (16bit integer=w2494:i16)
                        n1315 = Replace Array Subset(array=w2496, new element=w2489, index (row)=w2494, index (col)=1) -> (w2492:string[][])
                      }
                      frame True {
                        n1316 = local read "New: Temp"() -> (w2501:dbl)
                        n1317 = Search 1D Array(1D array=w2512, element="Width (um):") -> (index of element=w2506:i32)  [unwired: 1 in]
                        n1318 = Divide(x=w2506, y=3) -> (x/y=w2507:dbl)
                        n1319 = To Word Integer(number=w2507) -> (16bit integer=w2505:i16)
                        n1320 = Format Value(format string="%#g", value (0)=w2501) -> (output string=w2500:string)  [unwired: 1 in]
                        n1321 = Build Array(w2499, w2500) -> (w2503:string[])
                        n1322 = Increment(x=w2505) -> (x+1=w2504:i16)
                        n1323 = Insert Into Array(array=w2510, index (row)=w2504, new element=w2503) -> (w2509:string[][])  [unwired: 1 in]
                      }
                    }
                    n1324 = local write "Save1 Array"(w2485) -> ()
                  }
                  frame #5 {
                    w2522 = "Mobility-Sat (cm^2/Vs):"
                    n1325 = local read "Save1 Array"() -> (w2514:string[][])
                    n1326 = Array Size(array=w2514) -> (size(s)=w2519:i32[])
                    n1327 = Array Subset(array=w2514, index (row)=0, index (col)=0, length (col)=3) -> (w2515:string[][])  [unwired: 1 in]
                    n1328 = Index Array(array=w2519, index=0) -> (element=w2521:i32)
                    n1329 = Reshape Array(w2515, w2521) -> (w2513:string[])
                    n1330 = Search 1D Array(1D array=w2513, element=w2522) -> (index of element=w2525:i32)  [unwired: 1 in]
                    n1331 = Equal?(x=w2525, y=-1) -> (x = y?=w2524:bool)
                    n1332 = case shown="True" w2524 {
                      tunnel: w2514 -> [w2534 w2542]
                      tunnel: w2525 -> [w2531 _]
                      tunnel: [w2530 w2541] -> w2523
                      tunnel: w2513 -> [_ w2539]
                      tunnel: w2522 -> [_ w2537]
                      frame False {
                        n1333 = local read "New: Mobility-Sat"() -> (w2527:dbl)
                        n1334 = Divide(x=w2531, y=3) -> (x/y=w2533:dbl)
                        n1335 = To Word Integer(number=w2533) -> (16bit integer=w2532:i16)
                        n1336 = Format Value(format string="%#g", value (0)=w2527) -> (output string=w2528:string)  [unwired: 1 in]
                        n1337 = Replace Array Subset(array=w2534, new element=w2528, index (row)=w2532, index (col)=1) -> (w2530:string[][])
                      }
                      frame True {
                        n1338 = local read "New: Mobility-Sat"() -> (w2543:dbl)
                        n1339 = Search 1D Array(1D array=w2539, element="Mobility (cm^2/Vs):") -> (index of element=w2546:i32)  [unwired: 1 in]
                        n1340 = Divide(x=w2546, y=3) -> (x/y=w2547:dbl)
                        n1341 = To Word Integer(number=w2547) -> (16bit integer=w2538:i16)
                        n1342 = Format Value(format string="%#g", value (0)=w2543) -> (output string=w2540:string)  [unwired: 1 in]
                        n1343 = Build Array(w2537, w2540) -> (w2545:string[])
                        n1344 = Replace Array Subset(array=w2542, new element=w2545, index (row)=w2538) -> (w2541:string[][])  [unwired: 1 in]
                      }
                    }
                    n1345 = local write "Save1 Array"(w2523) -> ()
                  }
                  frame #6 {
                    w2559 = "Mobility-Lin (cm^2/Vs):"
                    n1346 = local read "Save1 Array"() -> (w2550:string[][])
                    n1347 = Array Size(array=w2550) -> (size(s)=w2556:i32[])
                    n1348 = Array Subset(array=w2550, index (row)=0, index (col)=0, length (col)=3) -> (w2552:string[][])  [unwired: 1 in]
                    n1349 = Index Array(array=w2556, index=0) -> (element=w2558:i32)
                    n1350 = Reshape Array(w2552, w2558) -> (w2551:string[])
                    n1351 = Search 1D Array(1D array=w2551, element=w2559) -> (index of element=w2562:i32)  [unwired: 1 in]
                    n1352 = Equal?(x=w2562, y=-1) -> (x = y?=w2561:bool)
                    n1353 = case shown="True" w2561 {
                      tunnel: w2550 -> [w2571 w2577]
                      tunnel: w2562 -> [w2568 _]
                      tunnel: [w2567 w2576] -> w2560
                      tunnel: w2551 -> [_ w2575]
                      tunnel: w2559 -> [_ w2574]
                      frame False {
                        n1354 = local read "Calc: Mobility-Lin"() -> (w2564:dbl)
                        n1355 = Divide(x=w2568, y=3) -> (x/y=w2570:dbl)
                        n1356 = To Word Integer(number=w2570) -> (16bit integer=w2569:i16)
                        n1357 = Format Value(format string="%#g", value (0)=w2564) -> (output string=w2565:string)  [unwired: 1 in]
                        n1358 = Replace Array Subset(array=w2571, new element=w2565, index (row)=w2569, index (col)=1) -> (w2567:string[][])
                      }
                      frame True {
                        n1359 = local read "Calc: Mobility-Lin"() -> (w2578:dbl)
                        n1360 = Search 1D Array(1D array=w2575, element="Mobility-Sat (cm^2/Vs):") -> (index of element=w2583:i32)  [unwired: 1 in]
                        n1361 = Divide(x=w2583, y=3) -> (x/y=w2584:dbl)
                        n1362 = To Word Integer(number=w2584) -> (16bit integer=w2582:i16)
                        n1363 = Format Value(format string="%#g", value (0)=w2578) -> (output string=w2587:string)  [unwired: 1 in]
                        n1364 = Build Array(w2574, w2587) -> (w2580:string[])
                        n1365 = Increment(x=w2582) -> (x+1=w2581:i16)
                        n1366 = Insert Into Array(array=w2577, index (row)=w2581, new element=w2580) -> (w2576:string[][])  [unwired: 1 in]
                      }
                    }
                    n1367 = local write "Save1 Array"(w2560) -> ()
                  }
                  frame #7 {
                    w2597 = "On/Off I-Sat:"
                    n1368 = local read "Save1 Array"() -> (w2588:string[][])
                    n1369 = Array Size(array=w2588) -> (size(s)=w2594:i32[])
                    n1370 = Array Subset(array=w2588, index (row)=0, index (col)=0, length (col)=3) -> (w2590:string[][])  [unwired: 1 in]
                    n1371 = Index Array(array=w2594, index=0) -> (element=w2596:i32)
                    n1372 = Reshape Array(w2590, w2596) -> (w2589:string[])
                    n1373 = Search 1D Array(1D array=w2589, element=w2597) -> (index of element=w2600:i32)  [unwired: 1 in]
                    n1374 = Equal?(x=w2600, y=-1) -> (x = y?=w2599:bool)
                    n1375 = case shown="True" w2599 {
                      tunnel: w2588 -> [w2609 w2616]
                      tunnel: w2600 -> [w2606 _]
                      tunnel: [w2605 w2617] -> w2598
                      tunnel: w2589 -> [_ w2614]
                      tunnel: w2597 -> [_ w2612]
                      frame False {
                        n1376 = local read "Calc: On/Off"() -> (w2602:dbl)
                        n1377 = Divide(x=w2606, y=3) -> (x/y=w2608:dbl)
                        n1378 = To Word Integer(number=w2608) -> (16bit integer=w2607:i16)
                        n1379 = Format Value(format string="%#g", value (0)=w2602) -> (output string=w2603:string)  [unwired: 1 in]
                        n1380 = Replace Array Subset(array=w2609, new element=w2603, index (row)=w2607, index (col)=1) -> (w2605:string[][])
                      }
                      frame True {
                        n1381 = local read "Calc: On/Off"() -> (w2618:dbl)
                        n1382 = Search 1D Array(1D array=w2614, element="On/Off Current:") -> (index of element=w2621:i32)  [unwired: 1 in]
                        n1383 = Divide(x=w2621, y=3) -> (x/y=w2622:dbl)
                        n1384 = To Word Integer(number=w2622) -> (16bit integer=w2613:i16)
                        n1385 = Format Value(format string="%#g", value (0)=w2618) -> (output string=w2615:string)  [unwired: 1 in]
                        n1386 = Build Array(w2612, w2615) -> (w2620:string[])
                        n1387 = Replace Array Subset(array=w2616, new element=w2620, index (row)=w2613) -> (w2617:string[][])  [unwired: 1 in]
                      }
                    }
                    n1388 = local write "Save1 Array"(w2598) -> ()
                  }
                  frame #8 {
                    w2634 = "Off I-Sat (A):"
                    n1389 = local read "Save1 Array"() -> (w2625:string[][])
                    n1390 = Array Size(array=w2625) -> (size(s)=w2631:i32[])
                    n1391 = Array Subset(array=w2625, index (row)=0, index (col)=0, length (col)=3) -> (w2627:string[][])  [unwired: 1 in]
                    n1392 = Index Array(array=w2631, index=0) -> (element=w2633:i32)
                    n1393 = Reshape Array(w2627, w2633) -> (w2626:string[])
                    n1394 = Search 1D Array(1D array=w2626, element=w2634) -> (index of element=w2637:i32)  [unwired: 1 in]
                    n1395 = Equal?(x=w2637, y=-1) -> (x = y?=w2636:bool)
                    n1396 = case shown="True" w2636 {
                      tunnel: w2625 -> [w2646 w2652]
                      tunnel: w2637 -> [w2643 _]
                      tunnel: [w2642 w2651] -> w2635
                      tunnel: w2626 -> [_ w2650]
                      tunnel: w2634 -> [_ w2649]
                      frame False {
                        n1397 = local read "Calc: Off I-Sat"() -> (w2641:dbl)
                        n1398 = Divide(x=w2643, y=3) -> (x/y=w2645:dbl)
                        n1399 = Format Value(format string="%#g", value (0)=w2641) -> (output string=w2639:string)  [unwired: 1 in]
                        n1400 = To Word Integer(number=w2645) -> (16bit integer=w2644:i16)
                        n1401 = Replace Array Subset(array=w2646, new element=w2639, index (row)=w2644, index (col)=1) -> (w2642:string[][])
                      }
                      frame True {
                        n1402 = local read "Calc: Off I-Sat"() -> (w2653:dbl)
                        n1403 = Search 1D Array(1D array=w2650, element="On/Off I-Sat:") -> (index of element=w2658:i32)  [unwired: 1 in]
                        n1404 = Divide(x=w2658, y=3) -> (x/y=w2659:dbl)
                        n1405 = To Word Integer(number=w2659) -> (16bit integer=w2657:i16)
                        n1406 = Format Value(format string="%#g", value (0)=w2653) -> (output string=w2662:string)  [unwired: 1 in]
                        n1407 = Build Array(w2649, w2662) -> (w2655:string[])
                        n1408 = Increment(x=w2657) -> (x+1=w2656:i16)
                        n1409 = Insert Into Array(array=w2652, index (row)=w2656, new element=w2655) -> (w2651:string[][])  [unwired: 1 in]
                      }
                    }
                    n1410 = local write "Save1 Array"(w2635) -> ()
                  }
                  frame #9 {
                    w2664 = "Vt-Sat (V):"
                    n1411 = local read "Save1 Array"() -> (w2665:string[][])
                    n1412 = Array Size(array=w2665) -> (size(s)=w2670:i32[])
                    n1413 = Array Subset(array=w2665, index (row)=0, index (col)=0, length (col)=3) -> (w2666:string[][])  [unwired: 1 in]
                    n1414 = Index Array(array=w2670, index=0) -> (element=w2672:i32)
                    n1415 = Reshape Array(w2666, w2672) -> (w2663:string[])
                    n1416 = Search 1D Array(1D array=w2663, element=w2664) -> (index of element=w2675:i32)  [unwired: 1 in]
                    n1417 = Equal?(x=w2675, y=-1) -> (x = y?=w2674:bool)
                    n1418 = case shown="True" w2674 {
                      tunnel: w2665 -> [w2682 w2691]
                      tunnel: w2675 -> [w2678 _]
                      tunnel: [w2677 w2690] -> w2673
                      tunnel: w2664 -> [_ w2689]
                      tunnel: w2663 -> [_ w2688]
                      frame False {
                        n1419 = local read "New: VT-Sat"() -> (w2684:dbl)
                        n1420 = Number To Fractional String(number=w2684) -> (F-format string=w2679:string)  [unwired: 3 in]
                        n1421 = Divide(x=w2678, y=3) -> (x/y=w2681:dbl)
                        n1422 = To Word Integer(number=w2681) -> (16bit integer=w2680:i16)
                        n1423 = Replace Array Subset(array=w2682, new element=w2679, index (row)=w2680, index (col)=1) -> (w2677:string[][])
                      }
                      frame True {
                        n1424 = local read "New: VT-Sat"() -> (w2692:dbl)
                        n1425 = Search 1D Array(1D array=w2688, element="Threshold V (V):") -> (index of element=w2687:i32)  [unwired: 1 in]
                        n1426 = Divide(x=w2687, y=3) -> (x/y=w2695:dbl)
                        n1427 = To Word Integer(number=w2695) -> (16bit integer=w2686:i16)
                        n1428 = Format Value(format string="%#g", value (0)=w2692) -> (output string=w2698:string)  [unwired: 1 in]
                        n1429 = Build Array(w2689, w2698) -> (w2694:string[])
                        n1430 = Replace Array Subset(array=w2691, new element=w2694, index (row)=w2686) -> (w2690:string[][])  [unwired: 1 in]
                      }
                    }
                    n1431 = local write "Save1 Array"(w2673) -> ()
                  }
                  frame #10 {
                    n1432 = local read "Save1 Array"() -> (w2699:string[][])
                    n1433 = Array Size(array=w2699) -> (size(s)=w2705:i32[])
                    n1434 = Array Subset(array=w2699, index (row)=0, index (col)=0, length (col)=3) -> (w2701:string[][])  [unwired: 1 in]
                    n1435 = Index Array(array=w2705, index=0) -> (element=w2707:i32)
                    n1436 = Reshape Array(w2701, w2707) -> (w2700:string[])
                    n1437 = Search 1D Array(1D array=w2700, element="VT-Lin (V):") -> (index of element=w2710:i32)  [unwired: 1 in]
                    n1438 = Equal?(x=w2710, y=-1) -> (x = y?=w2709:bool)
                    n1439 = case shown="False" w2709 {
                      tunnel: w2699 -> [w2720 w2723]
                      tunnel: w2710 -> [w2717 _]
                      tunnel: [w2716 w2723] -> w2708
                      frame False {
                        n1440 = local read "New: VT-Lin"() -> (w2714:dbl)
                        n1441 = Divide(x=w2717, y=3) -> (x/y=w2719:dbl)
                        n1442 = Format Value(format string="%#g", value (0)=w2714) -> (output string=w2713:string)  [unwired: 1 in]
                        n1443 = To Word Integer(number=w2719) -> (16bit integer=w2718:i16)
                        n1444 = Replace Array Subset(array=w2720, new element=w2713, index (row)=w2718, index (col)=1) -> (w2716:string[][])
                      }
                      frame True {
                      }
                    }
                    n1445 = local write "Save1 Array"(w2708) -> ()
                  }
                  frame #11 {
                    w2724 = "STS-Sat (V/decade):"
                    n1446 = local read "Save1 Array"() -> (w2726:string[][])
                    n1447 = Array Size(array=w2726) -> (size(s)=w2731:i32[])
                    n1448 = Array Subset(array=w2726, index (row)=0, index (col)=0, length (col)=3) -> (w2727:string[][])  [unwired: 1 in]
                    n1449 = Index Array(array=w2731, index=0) -> (element=w2733:i32)
                    n1450 = Reshape Array(w2727, w2733) -> (w2725:string[])
                    n1451 = Search 1D Array(1D array=w2725, element=w2724) -> (index of element=w2736:i32)  [unwired: 1 in]
                    n1452 = Equal?(x=w2736, y=-1) -> (x = y?=w2735:bool)
                    n1453 = case shown="True" w2735 {
                      tunnel: w2726 -> [w2745 w2751]
                      tunnel: w2736 -> [w2742 _]
                      tunnel: [w2741 w2752] -> w2734
                      tunnel: w2725 -> [_ w2750]
                      tunnel: w2724 -> [_ w2749]
                      frame False {
                        n1454 = local read "New: STS"() -> (w2739:dbl)
                        n1455 = Divide(x=w2742, y=3) -> (x/y=w2744:dbl)
                        n1456 = Format Value(format string="%#g", value (0)=w2739) -> (output string=w2738:string)  [unwired: 1 in]
                        n1457 = To Word Integer(number=w2744) -> (16bit integer=w2743:i16)
                        n1458 = Replace Array Subset(array=w2745, new element=w2738, index (row)=w2743, index (col)=1) -> (w2741:string[][])
                      }
                      frame True {
                        n1459 = local read "New: STS"() -> (w2753:dbl)
                        n1460 = Search 1D Array(1D array=w2750, element="S.T.S. (V/decade):") -> (index of element=w2756:i32)  [unwired: 1 in]
                        n1461 = Divide(x=w2756, y=3) -> (x/y=w2757:dbl)
                        n1462 = To Word Integer(number=w2757) -> (16bit integer=w2748:i16)
                        n1463 = Format Value(format string="%#g", value (0)=w2753) -> (output string=w2760:string)  [unwired: 1 in]
                        n1464 = Build Array(w2749, w2760) -> (w2755:string[])
                        n1465 = Replace Array Subset(array=w2751, new element=w2755, index (row)=w2748) -> (w2752:string[][])  [unwired: 1 in]
                      }
                    }
                    n1466 = local write "Save1 Array"(w2734) -> ()
                  }
                  frame #12 {
                    w2761 = "Trap Density-VT (Traps/Vcm^2):"
                    n1467 = local read "Save1 Array"() -> (w2763:string[][])
                    n1468 = Array Size(array=w2763) -> (size(s)=w2768:i32[])
                    n1469 = Array Subset(array=w2763, index (row)=0, index (col)=0, length (col)=3) -> (w2764:string[][])  [unwired: 1 in]
                    n1470 = Index Array(array=w2768, index=0) -> (element=w2770:i32)
                    n1471 = Reshape Array(w2764, w2770) -> (w2762:string[])
                    n1472 = Search 1D Array(1D array=w2762, element=w2761) -> (index of element=w2773:i32)  [unwired: 1 in]
                    n1473 = Equal?(x=w2773, y=-1) -> (x = y?=w2772:bool)
                    n1474 = case shown="True" w2772 {
                      tunnel: w2763 -> [w2782 w2787]
                      tunnel: w2773 -> [w2778 _]
                      tunnel: [w2777 w2788] -> w2771
                      tunnel: w2762 -> [_ w2786]
                      tunnel: w2761 -> [_ w2785]
                      frame False {
                        n1475 = local read "New: Trap Density-VT"() -> (w2776:dbl)
                        n1476 = Format Value(format string="%#g", value (0)=w2776) -> (output string=w2779:string)  [unwired: 1 in]
                        n1477 = Divide(x=w2778, y=3) -> (x/y=w2781:dbl)
                        n1478 = To Word Integer(number=w2781) -> (16bit integer=w2780:i16)
                        n1479 = Replace Array Subset(array=w2782, new element=w2779, index (row)=w2780, index (col)=1) -> (w2777:string[][])
                      }
                      frame True {
                        n1480 = local read "New: Trap Density-VT"() -> (w2798:dbl)
                        n1481 = Search 1D Array(1D array=w2786, element="STS-Sat (V/decade):") -> (index of element=w2793:i32)  [unwired: 1 in]
                        n1482 = Divide(x=w2793, y=3) -> (x/y=w2792:dbl)
                        n1483 = To Word Integer(number=w2792) -> (16bit integer=w2794:i16)
                        n1484 = Format Value(format string="%#g", value (0)=w2798) -> (output string=w2789:string)  [unwired: 1 in]
                        n1485 = Build Array(w2785, w2789) -> (w2796:string[])
                        n1486 = Increment(x=w2794) -> (x+1=w2795:i16)
                        n1487 = Insert Into Array(array=w2787, index (row)=w2795, new element=w2796) -> (w2788:string[][])  [unwired: 1 in]
                      }
                    }
                    n1488 = local write "Save1 Array"(w2771) -> ()
                  }
                  frame #13 {
                    w2800 = "Trap Density-STS (Traps/Vcm^2):"
                    n1489 = local read "Save1 Array"() -> (w2802:string[][])
                    n1490 = Array Size(array=w2802) -> (size(s)=w2807:i32[])
                    n1491 = Array Subset(array=w2802, index (row)=0, index (col)=0, length (col)=3) -> (w2803:string[][])  [unwired: 1 in]
                    n1492 = Index Array(array=w2807, index=0) -> (element=w2809:i32)
                    n1493 = Reshape Array(w2803, w2809) -> (w2801:string[])
                    n1494 = Search 1D Array(1D array=w2801, element=w2800) -> (index of element=w2811:i32)  [unwired: 1 in]
                    n1495 = Equal?(x=w2811, y=-1) -> (x = y?=w2810:bool)
                    n1496 = case shown="True" w2810 {
                      tunnel: w2802 -> [w2820 w2825]
                      tunnel: w2811 -> [w2817 _]
                      tunnel: [w2816 w2826] -> w2799
                      tunnel: w2801 -> [_ w2824]
                      tunnel: w2800 -> [_ w2823]
                      frame False {
                        n1497 = local read "New: Trap Density-STS"() -> (w2814:dbl)
                        n1498 = Divide(x=w2817, y=3) -> (x/y=w2819:dbl)
                        n1499 = To Word Integer(number=w2819) -> (16bit integer=w2818:i16)
                        n1500 = Format Value(format string="%#g", value (0)=w2814) -> (output string=w2813:string)  [unwired: 1 in]
                        n1501 = Replace Array Subset(array=w2820, new element=w2813, index (row)=w2818, index (col)=1) -> (w2816:string[][])
                      }
                      frame True {
                        n1502 = local read "New: Trap Density-STS"() -> (w2827:dbl)
                        n1503 = Search 1D Array(1D array=w2824, element="Trap Density-VT (Traps/Vcm^2):") -> (index of element=w2832:i32)  [unwired: 1 in]
                        n1504 = Divide(x=w2832, y=3) -> (x/y=w2833:dbl)
                        n1505 = To Word Integer(number=w2833) -> (16bit integer=w2831:i16)
                        n1506 = Format Value(format string="%#g", value (0)=w2827) -> (output string=w2836:string)  [unwired: 1 in]
                        n1507 = Build Array(w2823, w2836) -> (w2829:string[])
                        n1508 = Increment(x=w2831) -> (x+1=w2830:i16)
                        n1509 = Insert Into Array(array=w2825, index (row)=w2830, new element=w2829) -> (w2826:string[][])  [unwired: 1 in]
                      }
                    }
                    n1510 = local write "Save1 Array"(w2799) -> ()
                  }
                }
                n1511 = String To Path(string=w2373) -> (path=w2356:path)
                "No Image 2" <- w2356
              }
              frame #1 {
                n1512 = Equal?(x=w2840, y=w2839) -> (x = y?=w2838:bool)
                n1513 = case shown="False" w2838 {
                  tunnel: w2840 -> [w2844 _]
                  tunnel: w2839 -> [w2843 _]
                  frame False {
                    n1514 = Move(source path=w2844, 9:TRUE, 10:w2843) -> ()  [unwired: 2 in, 3 out]
                  }
                  frame True {
                  }
                }
              }
              frame #2 {
                n1515 = local write "Transfer File"(w2846) -> ()
                n1516 = call-poly <vilib>:"Write To Spreadsheet File.vi"("2D data"=w2845, "file path (dialog if empty)"=w2846) -> ()  [unwired: 6 in, 1 out]
              }
              frame #3 {
                w2946 = 0
                # "Moves to next file and displays new image/data"
                n1517 = property on="Image Out" class="ImageControl"() -> (error out=w2908:errorcluster, "Image Center Position"=w2912:cluster{"X":u32, "Y":u32})  [unwired: 2 in, 1 out]
                n1518 = local read "Transfer File"() -> (w2951:path)
                n1519 = Strip Path(path=w2951) -> (stripped path=w2942:path, name=w2960:string)
                n1520 = Unbundle(w2912) -> ("X"=w2910:u32)  [unwired: 1 out]
                n1521 = local write "Transfer Folder"(w2942) -> ()
                n1522 = Bundle("X"=w2910, 0) -> (w2911:cluster{"X":u32, i32})  [unwired: 1 in]
                n1523 = property on="Image Out" class="ImageControl"(error in=w2908, "Image Center Position"=w2911) -> ()  [unwired: 1 in, 2 out]
                n1524 = List Folder(path=w2942) -> (filenames=w2956:string[])  [unwired: 3 in, 3 out]
                n1525 = Search 1D Array(1D array=w2956, element=w2960) -> (index of element=w2953:i32)  [unwired: 1 in]
                n1526 = Array Size(array=w2956) -> (size(s)=w2952:i32)
                n1527 = Decrement(x=w2952) -> (x-1=w2954:i32)
                n1528 = Equal?(x=w2953, y=w2954) -> (x = y?=w2955:bool)
                n1529 = local read "Folder Index"() -> (w2904:dbl)
                n1530 = case shown="False" w2955 {
                  tunnel: w2904 -> [w3085 _]
                  tunnel: [w3084 0] -> w2903
                  frame False {
                    n1531 = Increment(x=w3085) -> (x+1=w3084:dbl)
                  }
                  frame True {
                  }
                }
                n1532 = invoke on="Image Out" class="ImageControl" method="Clear ROI"() -> ()  [unwired: 3 in, 3 out]
                n1533 = local write "Folder Index"(w2903) -> ()
                n1534 = Path To String(path=w2942) -> (string=w2961:string)
                n1535 = Index Array(array=w2956, index=w2903) -> (element=w2957:string)
                n1536 = local write "Data Name:"(w2957) -> ()
                n1537 = Concatenate Strings(w2961, "\\", w2957) -> (w2959:string)
                n1538 = String To Path(string=w2959) -> (path=w2855:path)
                n1539 = call "Recorded Values.vi"("Path"=w2855) -> ("Recorded Char"=w2857:T5, "Recorded Prop"=w2858:T6, "Fabrication Prop"=w2856:T7)  [unwired: 8 in]
                n1540 = Unbundle By Name(w2857) -> ("Mobility-Sat"=w2870:dbl, "Moblitity-Lin"=w2871:dbl, "On/Off"=w2872:dbl, "Off Current"=w2873:dbl, "Vt-Sat"=w2849:dbl, "STS"=w2874:dbl, "Trap Density-VT"=w2875:dbl, "Trap Density-STS"=w2876:dbl)
                n1541 = Unbundle By Name(w2858) -> ("Date Recorded"=w2866:string, "Index"=w2867:string, "Length"=w2868:dbl, "Width"=w2869:dbl, "Sample Temp"=w2852:dbl)
                n1542 = Unbundle By Name(w2856) -> ("Date Created"=w2877:string, "Material"=w2859:string, "Solvent"=w2860:string, "Concentration"=w2861:dbl, "Method"=w2862:string, "Dielectric (nm)"=w2863:dbl, "Treatment"=w2864:string, "Comments"=w2865:string)
                n1543 = local write "Rec: Off I-Sat"(w2873) -> ()
                n1544 = local write "Rec: Comments"(w2865) -> ()
                n1545 = local write "Rec: VT-Sat"(w2849) -> ()
                n1546 = local write "Date Created"(w2877) -> ()
                n1547 = local write "Rec: Material"(w2859) -> ()
                n1548 = local write "Rec: Solvent"(w2860) -> ()
                n1549 = local write "Rec: Concentration"(w2861) -> ()
                n1550 = local write "Rec: Method"(w2862) -> ()
                n1551 = local write "Rec: Dielectric (d)"(w2863) -> ()
                n1552 = local write "Surface Treatment:"(w2864) -> ()
                n1553 = local write "Index"(w2867) -> ()
                n1554 = local write "Rec: Mobility-Sat"(w2870) -> ()
                n1555 = local write "Rec: Mobility-Lin"(w2871) -> ()
                n1556 = local write "Rec: On/Off"(w2872) -> ()
                n1557 = local write "Rec: STS"(w2874) -> ()
                n1558 = local write "Rec: Trap Density-VT"(w2875) -> ()
                n1559 = local write "Rec: Trap Density-STS"(w2876) -> ()
                n1560 = local write "Date Recorded"(w2866) -> ()
                n1561 = local write "Rec: Length"(w2868) -> ()
                n1562 = local write "Rec: Width"(w2869) -> ()
                n1563 = local write "Rec: Temp"(w2852) -> ()
                n1564 = Equal To 0?(x=w2852) -> (x = 0?=w2853:bool)
                n1565 = case shown="False" w2853 {
                  tunnel: [w2962 w2963] -> w2850
                  tunnel: w2852 -> [w2962 _]
                  frame False {
                  }
                  frame True {
                    n1566 = local read "Room Temp"() -> (w2963:dbl)
                  }
                }
                n1567 = local write "Transfer File"(w2855) -> ()
                n1568 = local read "NumPts 2"() -> (w2899:dbl)
                n1569 = local read "NumPts"() -> (w2888:dbl)
                n1570 = local read "NumPts"() -> (w2900:dbl)
                n1571 = call-poly <vilib>:"Read From Spreadsheet File.vi"("file path (dialog if empty)"=w2855) -> ("all rows"=w2948:string[][])  [unwired: 6 in, 4 out]
                n1572 = call "Mobility-Vt Calculator-File.vi"("NumPts"=w2900, "Path"=w2855) -> ("XY Graph-Sat"=w2901:cluster{dbl[], dbl[]}[], "XY Graph-Lin"=w2883:cluster{dbl[], dbl[]}[], "Output"=w2902:T8, "Index-Sat"=w2880:dbl, "Index-Lin"=w2887:dbl)  [unwired: 4 in, 1 out]
                n1573 = Decimate 1D Array(w2883) -> (w2895:cluster{dbl[], dbl[]}[])  [unwired: 1 out]
                n1574 = Array To Cluster(array=w2895) -> (cluster=w2893:T9)
                n1575 = Unbundle(w2893) -> ("[0]"=w2894:cluster{dbl[], dbl[]})  [unwired: 8 out]
                n1576 = local write "XY Graph-Lin"(w2883) -> ()
                n1577 = Unbundle(w2894) -> (w2892:dbl[], w2891:dbl[])
                n1578 = Array Subset(array=w2891, index=w2887, length=w2888) -> (w2889:dbl[])
                n1579 = Array Subset(array=w2892, index=w2887, length=w2888) -> (w2890:dbl[])
                n1580 = call "STS Calculator-File.vi"("NumPts"=w2899, "Path"=w2855) -> ("STS Index-Sat"=w2898:dbl, "XY Graph-Sat"=w2897:cluster{dbl[], dbl[]}[], "Ouput"=w2896:cluster{"STS-Sat":dbl, "STS-Lin":dbl})  [unwired: 5 in, 2 out]
                n1581 = local read "New: Dielectric"() -> (w2882:dbl)
                n1582 = local write "Lin Id-Used"(w2889) -> ()
                n1583 = local write "Lin-Vg Array-Used"(w2890) -> ()
                n1584 = local write "MobVi Index"(w2880) -> ()
                n1585 = local write "Slide"(w2880) -> ()
                n1586 = local write "XY Graph"(w2901) -> ()
                n1587 = local write "Index 2"(w2898) -> ()
                n1588 = local write "XY Graph 2"(w2897) -> ()
                n1589 = Unbundle By Name(w2902) -> ("Mobility-Sat"=w2886:dbl, "Vt-Sat"=w2847:dbl, "Mobility-Lin"=w2885:dbl, "Mobility-Lin"=w2884:dbl, "Off I-Sat"=w2878:dbl, "On/Off I-Sat"=w2848:dbl)
                n1590 = Array Size(array=w2948) -> (size(s)=w2947:i32[])
                n1591 = local write "New: Temp"(w2850) -> ()
                n1592 = Unbundle By Name(w2896) -> ("STS-Sat"=w2881:dbl)
                n1593 = call "Trap Density_STS.vi"("Temp (T) [K]"=w2850, "S.T.S. (S)"=w2881, "Dielectric"=w2882) -> ("Trap Density (N)"=w2854:dbl)  [unwired: 8 in]
                n1594 = local write "Calc: Mobility-Lin"(w2885) -> ()
                n1595 = local write "Calc: Mobility-Sat"(w2886) -> ()
                n1596 = local write "Calc: Off I-Sat"(w2878) -> ()
                n1597 = local write "Calc: VT-Sat"(w2847) -> ()
                n1598 = local write "New: VT-Lin"(w2884) -> ()
                n1599 = local write "New: Trap Density-STS"(w2854) -> ()
                n1600 = local write "Calc: Trap Density-STS"(w2854) -> ()
                n1601 = local read "Image Folder"() -> (w2936:path)
                n1602 = local read "New: Dielectric"() -> (w2879:dbl)
                n1603 = Decimate 1D Array(w2901) -> (w2931:cluster{dbl[], dbl[]}[])  [unwired: 1 out]
                n1604 = Decimate 1D Array(w2897) -> (w2921:cluster{dbl[], dbl[]}[])  [unwired: 1 out]
                n1605 = Index Array(array=w2947, index=w2946) -> (element=w2927:i32)
                n1606 = Array Subset(array=w2948, index (row)=w2946, index (col)=w2946, length (col)=3) -> (w2949:string[][])  [unwired: 1 in]
                n1607 = local write "Calc: STS"(w2881) -> ()
                n1608 = local write "New: VT-Sat"(w2847) -> ()
                n1609 = local write "New: Mobility-Sat"(w2886) -> ()
                n1610 = local write "Calc: On/Off"(w2848) -> ()
                n1611 = local write "New: Mobility-Lin"(w2885) -> ()
                n1612 = List Folder(path=w2936) -> (filenames=w2941:string[])  [unwired: 3 in, 3 out]
                n1613 = local write "New: VT-Lin"(w2884) -> ()
                n1614 = Array To Cluster(array=w2931) -> (cluster=w2933:T9)
                n1615 = Array To Cluster(array=w2921) -> (cluster=w2919:T9)
                n1616 = Reshape Array(w2949, w2927) -> (w2934:string[])
                n1617 = Subtract(x=w2927, y=20) -> (x-y=w2926:i32)
                n1618 = local write "New: STS"(w2881) -> ()
                n1619 = property on="Slide" class="Slide (strict)"("Scale.Maximum"=w2926) -> ()  [unwired: 2 in, 2 out]
                n1620 = call "Trap Density_VT.vi"("VT"=w2847, "Dielectric"=w2879) -> ("Trap Density-VT"=w2851:dbl)
                n1621 = Unbundle(w2933) -> ("[0]"=w2932:cluster{dbl[], dbl[]})  [unwired: 8 out]
                n1622 = Unbundle(w2919) -> ("[0]"=w2920:cluster{dbl[], dbl[]})  [unwired: 8 out]
                n1623 = Search 1D Array(1D array=w2934, element="Index:") -> (index of element=w2943:i32)  [unwired: 1 in]
                n1624 = local write "New: Trap Density-VT"(w2851) -> ()
                n1625 = local write "Calc: Trap Density-VT"(w2851) -> ()
                n1626 = Unbundle(w2932) -> (w2923:dbl[], w2922:dbl[])
                n1627 = Unbundle(w2920) -> (w2918:dbl[], w2917:dbl[])
                n1628 = Increment(x=w2943) -> (x+1=w2944:i32)
                n1629 = Array Subset(array=w2923, index=w2880, length=w2900) -> (w2930:dbl[])
                n1630 = Array Subset(array=w2922, index=w2880, length=w2900) -> (w2929:dbl[])
                n1631 = Array Subset(array=w2918, index=w2898, length=w2899) -> (w2925:dbl[])
                n1632 = Array Subset(array=w2917, index=w2898, length=w2899) -> (w2924:dbl[])
                n1633 = Index Array(array=w2934, index=w2944) -> (element=w2939:string)
                n1634 = local write "Vg Array-Log-Used"(w2924) -> ()
                n1635 = local write "Sat Id-Log-Used"(w2925) -> ()
                n1636 = local write "Sat Id-Used"(w2929) -> ()
                n1637 = local write "Index"(w2939) -> ()
                n1638 = local write "Sat Vg Array-Used"(w2930) -> ()
                n1639 = while {
                  tunnel: w2941 -> [w2971]
                  tunnel: w2939 -> [w2969]
                  tunnel: [w2968] -> _
                  tunnel: [w2968] -> w2940
                  tunnel: w2927 -> [w2967]
                  i -> [w2968]
                  stop <- w2964 stop-if-true
                  n1640 = Index Array(array=w2971, index=w2968) -> (element=w2972:string)
                  n1641 = xnode "Match Regular Expression"("input string"=w2972, "regular expression"=w2969) -> ("whole match"=w2970:string)  [unwired: 4 in, 4 out]
                  n1642 = Equal?(x=w2970, y=w2969) -> (x = y?=w2966:bool)
                  n1643 = Equal?(x=w2967, y=w2968) -> (x = y?=w2965:bool)
                  n1644 = Or(x=w2966, y=w2965) -> (x .or. y?=w2964:bool)
                }
                n1645 = Path To String(path=w2936) -> (string=w2938:string)
                n1646 = Index Array(array=w2941, index=w2940) -> (element=w2915:string)
                n1647 = local write "Image Name"(w2915) -> ()
                n1648 = Empty String/Path?(string/path=w2915) -> (empty?=w2916:bool)
                n1649 = Concatenate Strings(w2938, "\\", w2915) -> (w2937:string)
                n1650 = String To Path(string=w2937) -> (path=w2914:path)
                n1651 = local read "No Image File"() -> (w2913:path)
                n1652 = Select(t=w2913, s=w2916, f=w2914) -> (s? t:f=w2907:path)
                n1653 = local write "Image File"(w2907) -> ()
                n1654 = local read "Image Out"() -> (w2905:T2)
                n1655 = call "IMAQ ReadFile"("File Path"=w2907, "Image"=w2905) -> ("Image Out"=w2906:T2)  [unwired: 5 in, 4 out]
                n1656 = local write "Image Out"(w2906) -> ()
                n1657 = local write "Image Out 2"(w2906) -> ()
              }
              frame #4 {
                # "Output ROI data"
                n1658 = local read "Image Folder"() -> (w3087:path)
                n1659 = Build Path(base path=w3087, name or relative path="ROI") -> (appended path=w3089:path)
                n1660 = local read "Index"() -> (w3088:string)
                n1661 = Build Path(base path=w3089, name or relative path=w3088) -> (appended path=w3094:path)
                n1662 = invoke on="Image Out" class="ImageControl" method="Clear ROI"() -> (error out=w3093:errorcluster)  [unwired: 3 in, 2 out]
                n1663 = call <vilib>:"Check if File or Folder Exists.vi"("error in (no error)"=w3093, "path"=w3094) -> ("file or folder exists?"=w3091:bool, "dup path"=w3092:path)  [unwired: 7 in, 1 out]
                n1664 = case shown="True" w3091 {
                  tunnel: w3092 -> [_ w3095]
                  frame False {
                  }
                  frame True {
                    n1665 = Read from Text File(file (use dialog)=w3095) -> (text=w3099:string)  [unwired: 3 in, 3 out]
                    n1666 = property on="Image Out" class="ImageControl"() -> ("ROI"=w3096:T10)  [unwired: 2 in, 2 out]
                    n1667 = Unflatten From String(type=w3096, binary string=w3099) -> (value=w3097:T10, error out=w3098:errorcluster)  [unwired: 3 in, 1 out]
                    n1668 = property on="Image Out" class="ImageControl"(error in=w3098, "ROI"=w3097) -> ()  [unwired: 1 in, 2 out]
                  }
                }
              }
            }
            n1669 = flat-sequence {
              tunnel: [w2313] -> w2300
              tunnel: w2300 -> [w2327]
              frame #0 {
                # "Makes Empty File for Transformer Data"
                n1670 = local read "Transfer Folder"() -> (w2302:path)
                n1671 = Build Path(base path=w2302, name or relative path="Stats") -> (appended path=w2304:path)
                n1672 = call <vilib>:"Check if File or Folder Exists.vi"("path"=w2304) -> ("file or folder exists?"=w2305:bool, "dup path"=w2306:path)  [unwired: 8 in, 1 out]
                n1673 = case shown="False" w2305 {
                  tunnel: [w2310 w2312] -> w2307
                  tunnel: w2306 -> [w2311 w2312]
                  frame False {
                    n1674 = Create Folder(path (use dialog)=w2311) -> (created path=w2310:path)  [unwired: 2 in, 2 out]
                  }
                  frame True {
                  }
                }
                n1675 = Build Path(base path=w2307, name or relative path="Tranformer Data.txt") -> (appended path=w2309:path)
                n1676 = call-poly <vilib>:"Write To Spreadsheet File.vi"("append to file? (new file:F)"=TRUE, "file path (dialog if empty)"=w2309) -> ()  [unwired: 6 in, 1 out]
              }
              frame #1 {
                # "Adds Headers if they don't exist"
                n1677 = local read "Transfer Folder"() -> (w2319:path)
                n1678 = Concatenate Strings("Stats\\", "Tranformer Data.txt") -> (w2320:string)
                n1679 = Build Path(base path=w2319, name or relative path=w2320) -> (appended path=w2313:path)
                n1680 = call-poly <vilib>:"Read From Spreadsheet File.vi"("file path (dialog if empty)"=w2313) -> ("first row"=w2318:string[])  [unwired: 6 in, 4 out]
                n1681 = Search 1D Array(1D array=w2318, element="DeviceID") -> (index of element=w2316:i32)  [unwired: 1 in]
                n1682 = Equal?(x=w2316, y=0) -> (x = y?=w2314:bool)
                n1683 = case shown="False" w2314 {
                  tunnel: w2313 -> [w2324 _]
                  frame False {
                    n1684 = local read "Transformer \nHeaders"() -> (w2323:string[])
                    n1685 = call-poly <vilib>:"Write To Spreadsheet File.vi"("1D data"=w2323, "file path (dialog if empty)"=w2324) -> ()  [unwired: 6 in, 1 out]
                  }
                  frame True {
                  }
                }
              }
              frame #2 {
                # "Adds current device if it doesn't exist"
                n1686 = local read "Current \nRecord"() -> (w2330:string[])
                n1687 = Index Array(array=w2330, index=0) -> (element=w2329:string)
                n1688 = local read "Transfer Folder"() -> (w2332:path)
                n1689 = Concatenate Strings("Stats\\", "Tranformer Data.txt") -> (w2333:string)
                n1690 = local write "Current Device ID"(w2329) -> ()
                n1691 = local read "Current Device ID"() -> (w2339:string)
                n1692 = Build Path(base path=w2332, name or relative path=w2333) -> (appended path=w2331:path)
                n1693 = call-poly <vilib>:"Read From Spreadsheet File.vi"("file path (dialog if empty)"=w2331) -> ("all rows"=w2326:string[][])  [unwired: 6 in, 4 out]
                n1694 = Index Array(array=w2326, index (col)=0) -> (element=w2337:string[])  [unwired: 1 in]
                n1695 = Search 1D Array(1D array=w2337, element=w2339) -> (index of element=w2325:i32)  [unwired: 1 in]
                n1696 = Equal?(x=w2325, y=-1) -> (x = y?=w2328:bool)
                n1697 = case shown="False" w2328 {
                  tunnel: w2327 -> [w2341 w2354]
                  tunnel: w2325 -> [w2346 _]
                  tunnel: w2326 -> [w2347 _]
                  frame False {
                    n1698 = local read "Current \nRecord"() -> (w2345:string[])
                    n1699 = Replace Array Subset(array=w2347, new element=w2345, index (row)=w2346) -> (w2342:string[][])  [unwired: 1 in]
                    n1700 = flat-sequence {
                      tunnel: [w2348] -> _
                      tunnel: [w2349] -> _
                      tunnel: [w2349] -> w2344
                      tunnel: [w2348] -> w2343
                      tunnel: w2342 -> [w2349]
                      tunnel: w2341 -> [w2348]
                      tunnel: w2344 -> [w2351]
                      tunnel: w2343 -> [w2350]
                      frame #0 {
                        n1701 = Delete(path (use dialog)=w2348) -> ()  [unwired: 4 in, 3 out]
                      }
                      frame #1 {
                        n1702 = call-poly <vilib>:"Write To Spreadsheet File.vi"("append to file? (new file:F)"=TRUE, "2D data"=w2351, "file path (dialog if empty)"=w2350) -> ()  [unwired: 5 in, 1 out]
                      }
                    }
                  }
                  frame True {
                    n1703 = local read "Current \nRecord"() -> (w2353:string[])
                    n1704 = call-poly <vilib>:"Write To Spreadsheet File.vi"("append to file? (new file:F)"=TRUE, "1D data"=w2353, "file path (dialog if empty)"=w2354) -> ()  [unwired: 5 in, 1 out]
                  }
                }
              }
            }
          }
          event "Export": Mouse Down {
            n1705 = event-data() -> ()  [unwired: 1 in, 7 out]
            n1706 = flat-sequence {
              frame #0 {
                n1707 = stacked-sequence {
                  frame #0 {
                    n1708 = local read "Independant Variable"() -> (w3101:string)
                    n1709 = Equal?(x=w3101, y="Length (um):") -> (x = y?=w3102:bool)
                    n1710 = case shown="True" w3102 {
                      frame False {
                      }
                      frame True {
                        n1711 = local write "X Axis Display Type"("1") -> ()
                        n1712 = local write "Opj X Axis"("2") -> ()
                      }
                    }
                  }
                  frame #1 {
                    n1713 = local read "Independant Variable"() -> (w3106:string)
                    n1714 = Equal?(x=w3106, y="Sample Temp (K):") -> (x = y?=w3107:bool)
                    n1715 = case shown="True" w3107 {
                      frame False {
                      }
                      frame True {
                        n1716 = local write "X Axis Display Type"("1") -> ()
                        n1717 = local write "Opj X Axis"("1") -> ()
                      }
                    }
                  }
                  frame #2 {
                    n1718 = local read "Independant Variable"() -> (w3111:string)
                    n1719 = Equal?(x=w3111, y="Mobility-Sat (cm^2/Vs):") -> (x = y?=w3112:bool)
                    n1720 = case shown="True" w3112 {
                      frame False {
                      }
                      frame True {
                        n1721 = local write "X Axis Display Type"("2") -> ()
                        n1722 = local write "Opj X Axis"("2") -> ()
                      }
                    }
                  }
                  frame #3 {
                    n1723 = local read "Independant Variable"() -> (w3116:string)
                    n1724 = Equal?(x=w3116, y="Mobility-Lin (cm^2/Vs):") -> (x = y?=w3117:bool)
                    n1725 = case shown="True" w3117 {
                      frame False {
                      }
                      frame True {
                        n1726 = local write "X Axis Display Type"("2") -> ()
                        n1727 = local write "Opj X Axis"("2") -> ()
                      }
                    }
                  }
                  frame #4 {
                    n1728 = local read "Independant Variable"() -> (w3121:string)
                    n1729 = Equal?(x=w3121, y="On/Off I-Sat:") -> (x = y?=w3122:bool)
                    n1730 = case shown="True" w3122 {
                      frame False {
                      }
                      frame True {
                        n1731 = local write "X Axis Display Type"("2") -> ()
                        n1732 = local write "Opj X Axis"("2") -> ()
                      }
                    }
                  }
                  frame #5 {
                    n1733 = local read "Independant Variable"() -> (w3126:string)
                    n1734 = Equal?(x=w3126, y="Off I-Sat (A):") -> (x = y?=w3127:bool)
                    n1735 = case shown="True" w3127 {
                      frame False {
                      }
                      frame True {
                        n1736 = local write "X Axis Display Type"("2") -> ()
                        n1737 = local write "Opj X Axis"("2") -> ()
                      }
                    }
                  }
                  frame #6 {
                    n1738 = local read "Independant Variable"() -> (w3131:string)
                    n1739 = Equal?(x=w3131, y="Vt-Sat (V):") -> (x = y?=w3132:bool)
                    n1740 = case shown="True" w3132 {
                      frame False {
                      }
                      frame True {
                        n1741 = local write "X Axis Display Type"("1") -> ()
                        n1742 = local write "Opj X Axis"("1") -> ()
                      }
                    }
                  }
                  frame #7 {
                    n1743 = local read "Independant Variable"() -> (w3136:string)
                    n1744 = Equal?(x=w3136, y="STS-Sat (V/decade):") -> (x = y?=w3137:bool)
                    n1745 = case shown="True" w3137 {
                      frame False {
                      }
                      frame True {
                        n1746 = local write "X Axis Display Type"("1") -> ()
                        n1747 = local write "Opj X Axis"("1") -> ()
                      }
                    }
                  }
                  frame #8 {
                    n1748 = local read "Independant Variable"() -> (w3141:string)
                    n1749 = Equal?(x=w3141, y="Trap Density-VT (Traps/Vcm^2):") -> (x = y?=w3142:bool)
                    n1750 = case shown="True" w3142 {
                      frame False {
                      }
                      frame True {
                        n1751 = local write "X Axis Display Type"("2") -> ()
                        n1752 = local write "Opj X Axis"("2") -> ()
                      }
                    }
                  }
                  frame #9 {
                    n1753 = local read "Independant Variable"() -> (w3146:string)
                    n1754 = Equal?(x=w3146, y="Trap Density-STS (Traps/Vcm^2):") -> (x = y?=w3147:bool)
                    n1755 = case shown="True" w3147 {
                      frame False {
                      }
                      frame True {
                        n1756 = local write "X Axis Display Type"("2") -> ()
                        n1757 = local write "Opj X Axis"("2") -> ()
                      }
                    }
                  }
                }
              }
              frame #1 {
                n1758 = local read "Transfer Folder"() -> (w3155:path)
                n1759 = Build Path(base path=w3155, name or relative path="Stats") -> (appended path=w3156:path)
                n1760 = local read "Origin Project File"() -> (w3167:path)
                n1761 = call <vilib>:"Check if File or Folder Exists.vi"("path"=w3156) -> ("file or folder exists?"=w3171:bool, "dup path"=w3170:path)  [unwired: 8 in, 1 out]
                n1762 = call <userlib>:"OA_ConnectToOrigin.vi"() -> ("error out"=w3168:errorcluster, "Origin.IOApplication"=w3169:refnum<k7>)  [unwired: 8 in]
                n1763 = case shown="False" w3171 {
                  tunnel: w3170 -> [w3344 w3345]
                  tunnel: [w3343 w3345] -> w3154
                  frame False {
                    n1764 = Create Folder(path (use dialog)=w3344) -> (created path=w3343:path)  [unwired: 2 in, 2 out]
                  }
                  frame True {
                  }
                }
                n1765 = call <userlib>:"OA_Load.vi"("error in (no error)"=w3168, "Path"=w3167, "Origin.IOApplication"=w3169) -> ("error out"=w3165:errorcluster, "Origin.IOApplication"=w3166:refnum<k7>)  [unwired: 1 out]
                n1766 = call <userlib>:"OAExecute.vi"("script"="document -m 3;", "Error IO"=w3165, "Origin.IOApplication"=w3166) -> ("Error IO Out"=w3163:errorcluster, "Origin.IOApplication"=w3164:refnum<k7>)  [unwired: 1 in, 1 out]
                n1767 = call "File Dialog"("start path"=w3156) -> ("selected path"=w3158:path)  [unwired: 11 in, 3 out]
                n1768 = local read "Independant Variable"() -> (w3151:string)
                n1769 = stacked-sequence {
                  tunnel: w3155 -> [w3182 w3212 w3224 w3246 w3266 w3287 w3308 w3331]
                  tunnel: w3154 -> [w3183 w3211 w3225 w3245 w3267 w3288 w3309 w3332]
                  tunnel: w3164 -> [w3185 w3209 w3227 w3248 w3269 w3290 w3311 w3334]
                  tunnel: w3163 -> [w3184 w3210 w3226 w3247 w3268 w3289 w3310 w3333]
                  tunnel: [_ _ _ _ _ _ _ w3329] -> w3153
                  tunnel: [_ _ _ _ _ _ _ w3330] -> w3152
                  tunnel: w3151 -> [w3181 w3202 w3223 w3244 w3265 w3286 w3307 w3328]
                  frame #0 {
                    n1770 = local read "X Axis Display Type"() -> (w3173:string)
                    n1771 = local read "Opj X Axis"() -> (w3178:string)
                    n1772 = Concatenate Strings("window -a MOBLGraph;\nlayer.x.type=", w3178, "; layer.x.label.numFormat = ", w3173, "; Y3 = 1; X3 = 1;", "window -a MOBLTable;\nwindow -s TV;") -> (w3176:string)
                    n1773 = call "Param_Analysis_7_24b_JW.vi"("Independant Variable"=w3181, "error in (no error)"=w3184, "Data Folder"=w3182, "Parameter String"="Mobility-Lin (cm^2/Vs):", "Parameter Name"="Mobility-Lin", "Stats Folder"=w3183) -> ("error out"=w3187:errorcluster, "Output Array"=w3189:string[][], "Variables"=w3180:T16)  [unwired: 2 in, 1 out]
                    n1774 = call "Origin_Export_7_27a_JW.vi"("Input Conditions"=w3180, "Analysis Array"=w3189, "error in (no error)"=w3187, "Parameter Worksheet Name"="[MOBLTable]Mobilities", "Parameter Folder Script"="pe_cd \"Mobility-Lin\";", "Origin.IOApplication"=w3185) -> ("error out"=w3186:errorcluster, "reference out"=w3188:refnum<k7>)  [unwired: 3 in, 1 out]
                    n1775 = call <userlib>:"OAExecute.vi"("script"=w3176, "Error IO"=w3186, "Origin.IOApplication"=w3188) -> ()  [unwired: 1 in, 3 out]
                  }
                  frame #1 {
                    n1776 = local read "X Axis Display Type"() -> (w3194:string)
                    n1777 = local read "Opj X Axis"() -> (w3199:string)
                    n1778 = Concatenate Strings("window -a MOBSGraph;\nlayer.x.type=", w3199, "; layer.x.label.numFormat = ", w3194, "; Y3 = 1; X3 = 1;", "window -a MOBSTable;\nwindow -s TV;") -> (w3197:string)
                    n1779 = call "Param_Analysis_7_24b_JW.vi"("Independant Variable"=w3202, "error in (no error)"=w3210, "Data Folder"=w3212, "Parameter String"="Mobility-Sat (cm^2/Vs):", "Parameter Name"="Mobility-Sat", "Stats Folder"=w3211) -> ("error out"=w3205:errorcluster, "Output Array"=w3203:string[][], "Variables"=w3201:T16)  [unwired: 2 in, 1 out]
                    n1780 = call "Origin_Export_7_27a_JW.vi"("Input Conditions"=w3201, "Analysis Array"=w3203, "error in (no error)"=w3205, "Parameter Worksheet Name"="[MOBSTable]Mobilities", "Parameter Folder Script"="pe_cd \"Mobility-Sat\";", "Origin.IOApplication"=w3209) -> ("error out"=w3204:errorcluster, "reference out"=w3206:refnum<k7>)  [unwired: 3 in, 1 out]
                    n1781 = call <userlib>:"OAExecute.vi"("script"=w3197, "Error IO"=w3204, "Origin.IOApplication"=w3206) -> ()  [unwired: 1 in, 3 out]
                  }
                  frame #2 {
                    n1782 = local read "X Axis Display Type"() -> (w3215:string)
                    n1783 = local read "Opj X Axis"() -> (w3220:string)
                    n1784 = Concatenate Strings("window -a NSTSGraph;\nlayer.x.type=", w3220, "; layer.x.label.numFormat = ", w3215, "; Y3 = 1; X3 = 1;", "window -a NSTSTable;\nwindow -s TV;") -> (w3218:string)
                    n1785 = call "Param_Analysis_7_24b_JW.vi"("Independant Variable"=w3223, "error in (no error)"=w3226, "Data Folder"=w3224, "Parameter String"="Trap Density-STS (Traps/Vcm^2):", "Parameter Name"="Trap Density-STS", "Stats Folder"=w3225) -> ("error out"=w3230:errorcluster, "Output Array"=w3228:string[][], "Variables"=w3222:T16)  [unwired: 2 in, 1 out]
                    n1786 = call "Origin_Export_7_27a_JW.vi"("Input Conditions"=w3222, "Analysis Array"=w3228, "error in (no error)"=w3230, "Parameter Worksheet Name"="[NSTSTable]Trap Densities", "Parameter Folder Script"="pe_cd \"N-STS\";", "Origin.IOApplication"=w3227) -> ("error out"=w3229:errorcluster, "reference out"=w3231:refnum<k7>)  [unwired: 3 in, 1 out]
                    n1787 = call <userlib>:"OAExecute.vi"("script"=w3218, "Error IO"=w3229, "Origin.IOApplication"=w3231) -> ()  [unwired: 1 in, 3 out]
                  }
                  frame #3 {
                    n1788 = local read "X Axis Display Type"() -> (w3236:string)
                    n1789 = local read "Opj X Axis"() -> (w3241:string)
                    n1790 = call "Param_Analysis_7_24b_JW.vi"("Independant Variable"=w3244, "error in (no error)"=w3247, "Data Folder"=w3246, "Parameter String"="Trap Density-VT (Traps/Vcm^2):", "Parameter Name"="Trap Density-Vt", "Stats Folder"=w3245) -> ("error out"=w3251:errorcluster, "Output Array"=w3249:string[][], "Variables"=w3243:T16)  [unwired: 2 in, 1 out]
                    n1791 = Concatenate Strings("window -a NVtGraph;\nlayer.x.type=", w3241, "; layer.x.label.numFormat = ", w3236, "; Y3 = 1; X3 = 1;", "window -a NVtTable;\nwindow -s TV;") -> (w3239:string)
                    n1792 = call "Origin_Export_7_27a_JW.vi"("Input Conditions"=w3243, "Analysis Array"=w3249, "error in (no error)"=w3251, "Parameter Worksheet Name"="[NVTTable]Trap Densities", "Parameter Folder Script"="pe_cd \"N-Vt\";", "Origin.IOApplication"=w3248) -> ("error out"=w3250:errorcluster, "reference out"=w3252:refnum<k7>)  [unwired: 3 in, 1 out]
                    n1793 = call <userlib>:"OAExecute.vi"("script"=w3239, "Error IO"=w3250, "Origin.IOApplication"=w3252) -> ()  [unwired: 1 in, 3 out]
                  }
                  frame #4 {
                    n1794 = local read "X Axis Display Type"() -> (w3257:string)
                    n1795 = local read "Opj X Axis"() -> (w3262:string)
                    n1796 = Concatenate Strings("window -a OffIGraph;\nlayer.x.type=", w3262, "; layer.x.label.numFormat = ", w3257, "; Y3 = 1; X3 = 1;", "window -a OffITable;\nwindow -s TV;") -> (w3260:string)
                    n1797 = call "Param_Analysis_7_24b_JW.vi"("Independant Variable"=w3265, "error in (no error)"=w3268, "Data Folder"=w3266, "Parameter String"="Off I-Sat (A):", "Parameter Name"="Off I-Sat", "Stats Folder"=w3267) -> ("error out"=w3272:errorcluster, "Output Array"=w3270:string[][], "Variables"=w3264:T16)  [unwired: 2 in, 1 out]
                    n1798 = call "Origin_Export_7_27a_JW.vi"("Input Conditions"=w3264, "Analysis Array"=w3270, "error in (no error)"=w3272, "Parameter Worksheet Name"="[OffItable]OffCurrents", "Parameter Folder Script"="pe_cd \"OffI-Sat\";", "Origin.IOApplication"=w3269) -> ("error out"=w3271:errorcluster, "reference out"=w3273:refnum<k7>)  [unwired: 3 in, 1 out]
                    n1799 = call <userlib>:"OAExecute.vi"("script"=w3260, "Error IO"=w3271, "Origin.IOApplication"=w3273) -> ()  [unwired: 1 in, 3 out]
                  }
                  frame #5 {
                    n1800 = local read "X Axis Display Type"() -> (w3278:string)
                    n1801 = local read "Opj X Axis"() -> (w3283:string)
                    n1802 = Concatenate Strings("window -a OnOffGraph;\nlayer.x.type=", w3283, "; layer.x.label.numFormat = ", w3278, "; Y3 = 1; X3 = 1;", "window -a OnOffTable;\nwindow -s TV;") -> (w3281:string)
                    n1803 = call "Param_Analysis_7_24b_JW.vi"("Independant Variable"=w3286, "error in (no error)"=w3289, "Data Folder"=w3287, "Parameter String"="On/Off I-Sat:", "Parameter Name"="OnOff Ratio", "Stats Folder"=w3288) -> ("error out"=w3293:errorcluster, "Output Array"=w3291:string[][], "Variables"=w3285:T16)  [unwired: 2 in, 1 out]
                    n1804 = call "Origin_Export_7_27a_JW.vi"("Input Conditions"=w3285, "Analysis Array"=w3291, "error in (no error)"=w3293, "Parameter Worksheet Name"="[OnOffTable]On/Off Ratios", "Parameter Folder Script"="pe_cd \"OnOff-Ratio\";", "Origin.IOApplication"=w3290) -> ("error out"=w3292:errorcluster, "reference out"=w3294:refnum<k7>)  [unwired: 3 in, 1 out]
                    n1805 = call <userlib>:"OAExecute.vi"("script"=w3281, "Error IO"=w3292, "Origin.IOApplication"=w3294) -> ()  [unwired: 1 in, 3 out]
                  }
                  frame #6 {
                    n1806 = local read "X Axis Display Type"() -> (w3299:string)
                    n1807 = local read "Opj X Axis"() -> (w3304:string)
                    n1808 = call "Param_Analysis_7_24b_JW.vi"("Independant Variable"=w3307, "error in (no error)"=w3310, "Data Folder"=w3308, "Parameter String"="STS-Sat (V/decade):", "Parameter Name"="STS-Sat", "Stats Folder"=w3309) -> ("error out"=w3314:errorcluster, "Output Array"=w3312:string[][], "Variables"=w3306:T16)  [unwired: 2 in, 1 out]
                    n1809 = Concatenate Strings("window -a SGraph;\nlayer.x.type=", w3304, "; layer.x.label.numFormat = ", w3299, "; Y3 = 1; X3 = 1;", "window -a STable;\nwindow -s TV;") -> (w3302:string)
                    n1810 = call "Origin_Export_7_27a_JW.vi"("Input Conditions"=w3306, "Analysis Array"=w3312, "error in (no error)"=w3314, "Parameter Worksheet Name"="[STable]Threshold Swing", "Parameter Folder Script"="pe_cd \"STS-Sat\";", "Origin.IOApplication"=w3311) -> ("error out"=w3313:errorcluster, "reference out"=w3315:refnum<k7>)  [unwired: 3 in, 1 out]
                    n1811 = call <userlib>:"OAExecute.vi"("script"=w3302, "Error IO"=w3313, "Origin.IOApplication"=w3315) -> ()  [unwired: 1 in, 3 out]
                  }
                  frame #7 {
                    n1812 = local read "X Axis Display Type"() -> (w3320:string)
                    n1813 = local read "Opj X Axis"() -> (w3325:string)
                    n1814 = Concatenate Strings("window -a VtGraph;\nlayer.x.type=", w3325, "; layer.x.label.numFormat = ", w3320, "; Y3 = 1; X3 = 1;", "window -a VtTable;\nwindow -s TV;") -> (w3323:string)
                    n1815 = call "Param_Analysis_7_24b_JW.vi"("Independant Variable"=w3328, "error in (no error)"=w3333, "Data Folder"=w3331, "Parameter String"="Vt-Sat (V):", "Parameter Name"="Vt-Sat", "Stats Folder"=w3332) -> ("error out"=w3337:errorcluster, "Output Array"=w3335:string[][], "Variables"=w3327:T16)  [unwired: 2 in, 1 out]
                    n1816 = call "Origin_Export_7_27a_JW.vi"("Input Conditions"=w3327, "Analysis Array"=w3335, "error in (no error)"=w3337, "Parameter Worksheet Name"="[VtTable]Threshold Voltages", "Parameter Folder Script"="pe_cd \"Vt-Sat\";", "Origin.IOApplication"=w3334) -> ("error out"=w3336:errorcluster, "reference out"=w3338:refnum<k7>)  [unwired: 3 in, 1 out]
                    n1817 = call <userlib>:"OAExecute.vi"("script"=w3323, "Error IO"=w3336, "Origin.IOApplication"=w3338) -> ("Error IO Out"=w3329:errorcluster, "Origin.IOApplication"=w3330:refnum<k7>)  [unwired: 1 in, 1 out]
                  }
                }
                n1818 = Path To String(path=w3158) -> (string=w3157:string)
                n1819 = call <userlib>:"OAExecute.vi"("script"="pe_cd /; ", "Error IO"=w3153, "Origin.IOApplication"=w3152) -> ("Error IO Out"=w3159:errorcluster, "Origin.IOApplication"=w3160:refnum<k7>)  [unwired: 1 in, 1 out]
                n1820 = call <userlib>:"OASaveProject.vi"("path"=w3157, "Error IO"=w3159, "Origin.IOApplication"=w3160) -> ()  [unwired: 3 out]
              }
            }
          }
          event "Blank Button": Mouse Down {
            n1821 = event-data() -> ()  [unwired: 1 in, 7 out]
            n1822 = local read "Transfer File"() -> (w3353:path)
            n1823 = disable-structure shown="Disabled" {
              frame Disabled {
                n1824 = local read "Folder Index"() -> (w3354:dbl)
                n1825 = Decrement(x=w3354) -> (x-1=w3355:dbl)
                n1826 = local write "Folder Index"(w3355) -> ()
              }
              frame Enabled {
              }
            }
            n1827 = Strip Path(path=w3353) -> (stripped path=w3349:path, name=w3351:string)
            n1828 = Path To String(path=w3349) -> (string=w3348:string)
            n1829 = Concatenate Strings(w3348, "\\", "X_", w3351) -> (w3347:string)
            n1830 = String To Path(string=w3347) -> (path=w3346:path)
            n1831 = Move(source path=w3353, 10:w3346) -> ()  [unwired: 3 in, 3 out]
            n1832 = local write "Transfer File"(w3346) -> ()
          }
          event "Cancel Button": Mouse Down {
            (unwired) 6
            n1833 = event-data() -> ()  [unwired: 1 in, 7 out]
            n1834 = call "Simulate_Keyboard.vi"("Action"=2, "Virtual Key"=162) -> ()  [unwired: 7 in, 1 out]
          }
        }
        n1835 = Multiply(x=w525, y=10) -> (x*y=w527:sgl)
        n1836 = case shown="\"0\"" w566 {
          tunnel: w540 -> [w637 w643 w647 w649 w653 w655 w657 w659 w661 w663 w665 w667 w669 w671 w673 w675 w677 w679 w681 w683 w685 w687 w689 w691 w693 w695 w697 w699 w701 w703 w705 w707 w709 w711 w713 w715 w717 w719 w721 w723 w725 w727 w729 w731 w733 w735 w737 w739 w741 w743 w745 w747 w749 w751 w753 w755 w757 w759 w761 w763 w765 w767 w769 w771 w773 w775 w777 w779 w781 w783 w785 w787 w789 w791 w793 w795 w797 w799 w801 w803 w805 w807 w809 w811 w813 w815 w817 w819 w821 w823 w825 w827 w829 w831 w833 w835 w837 w839 w841 w843 w845 w847 w849 w851 w853]
          tunnel: [w637 w642 w646 w649 w653 w655 w657 w659 w661 w663 w665 w667 w669 w671 w673 w675 w677 w679 w681 w683 w685 w687 w689 w691 w693 w695 w697 w699 w701 w703 w705 w707 w709 w711 w713 w715 w717 w719 w721 w723 w725 w727 w729 w731 w733 w735 w737 w739 w741 w743 w745 w747 w749 w751 w753 w755 w757 w759 w761 w763 w765 w767 w769 w771 w773 w775 w777 w779 w781 w783 w785 w787 w789 w791 w793 w795 w797 w799 w801 w803 w805 w807 w809 w811 w813 w815 w817 w819 w821 w823 w825 w827 w829 w831 w833 w835 w837 w839 w841 w843 w845 w847 w849 w851 w853] -> w565
          tunnel: w541 -> [w639 w641 w645 w651 w652 w654 w656 w658 w660 w662 w664 w666 w668 w670 w672 w674 w676 w678 w680 w682 w684 w686 w688 w690 w692 w694 w696 w698 w700 w702 w704 w706 w708 w710 w712 w714 w716 w718 w720 w722 w724 w726 w728 w730 w732 w734 w736 w738 w740 w742 w744 w746 w748 w750 w752 w754 w756 w758 w760 w762 w764 w766 w768 w770 w772 w774 w776 w778 w780 w782 w784 w786 w788 w790 w792 w794 w796 w798 w800 w802 w804 w806 w808 w810 w812 w814 w816 w818 w820 w822 w824 w826 w828 w830 w832 w834 w836 w838 w840 w842 w844 w846 w848 w850 w852]
          tunnel: [w638 w641 w645 w650 w652 w654 w656 w658 w660 w662 w664 w666 w668 w670 w672 w674 w676 w678 w680 w682 w684 w686 w688 w690 w692 w694 w696 w698 w700 w702 w704 w706 w708 w710 w712 w714 w716 w718 w720 w722 w724 w726 w728 w730 w732 w734 w736 w738 w740 w742 w744 w746 w748 w750 w752 w754 w756 w758 w760 w762 w764 w766 w768 w770 w772 w774 w776 w778 w780 w782 w784 w786 w788 w790 w792 w794 w796 w798 w800 w802 w804 w806 w808 w810 w812 w814 w816 w818 w820 w822 w824 w826 w828 w830 w832 w834 w836 w838 w840 w842 w844 w846 w848 w850 w852] -> w564
          tunnel: w527 -> [w636 w640 w644 w648 _ _ _ _ _ _ _ _ _ _ _ _ _ _ _ _ _ _ _ _ _ _ _ _ _ _ _ _ _ _ _ _ _ _ _ _ _ _ _ _ _ _ _ _ _ _ _ _ _ _ _ _ _ _ _ _ _ _ _ _ _ _ _ _ _ _ _ _ _ _ _ _ _ _ _ _ _ _ _ _ _ _ _ _ _ _ _ _ _ _ _ _ _ _ _ _ _ _ _ _ _]
          frame "DOWN" {
            n1837 = Add(x=w639, y=w636) -> (x+y=w638:sgl)
          }
          frame "LEFT" {
            n1838 = Subtract(x=w643, y=w640) -> (x-y=w642:sgl)
          }
          frame "RIGHT" {
            n1839 = Add(x=w647, y=w644) -> (x+y=w646:sgl)
          }
          frame "UP" {
            n1840 = Subtract(x=w651, y=w648) -> (x-y=w650:sgl)
          }
          frame "ENTER (num pad)" {
          }
          frame "' (quote)" {
          }
          frame "END" {
          }
          frame "EQUALS" {
          }
          frame "ESCAPE" {
          }
          frame "GRAVE (`)" {
          }
          frame "HOME" {
          }
          frame "INSERT" {
          }
          frame "LBRACKET" {
          }
          frame "LCONTROL" {
          }
          frame "L ALT" {
          }
          frame "LSHIFT" {
          }
          frame "LWIN" {
          }
          frame "MINUS" {
          }
          frame "MULTIPLY" {
          }
          frame "NEXT" {
          }
          frame "NUMLOCK" {
          }
          frame "NUMPAD_0" {
          }
          frame "NUMPAD_1" {
          }
          frame "NUMPAD_2" {
          }
          frame "NUMPAD_3" {
          }
          frame "NUMPAD_4" {
          }
          frame "NUMPAD_5" {
          }
          frame "NUMPAD_6" {
          }
          frame "NUMPAD_7" {
          }
          frame "NUMPAD_8" {
          }
          frame "NUMPAD_9" {
          }
          frame "PAUSE" {
          }
          frame "PERIOD" {
          }
          frame "PRIOR (PG UP)" {
          }
          frame "RBRACKET" {
          }
          frame "RCONTROL" {
          }
          frame "RETURN" {
          }
          frame "R ALT" {
          }
          frame "RSHIFT" {
          }
          frame "RWIN" {
          }
          frame "SCROLL" {
          }
          frame "SEMICOLON" {
          }
          frame "SLASH" {
          }
          frame "SPACE" {
          }
          frame "SUBTRACT" {
          }
          frame "TAB" {
          }
          frame "DIVIDE" {
          }
          frame "DELETE" {
          }
          frame "DECIMAL" {
          }
          frame "COMMA" {
          }
          frame "CAPITAL" {
          }
          frame "BACKSLASH" {
          }
          frame "BACK" {
          }
          frame "ADD" {
          }
          frame "F15" {
          }
          frame "F14" {
          }
          frame "F13" {
          }
          frame "F12" {
          }
          frame "F11" {
          }
          frame "F10" {
          }
          frame "F9" {
          }
          frame "F8" {
          }
          frame "F7" {
          }
          frame "F6" {
          }
          frame "F5" {
          }
          frame "F4" {
          }
          frame "F3" {
          }
          frame "F2" {
          }
          frame "F1" {
          }
          frame "Z" {
          }
          frame "Y" {
          }
          frame "X" {
          }
          frame "W" {
          }
          frame "V" {
          }
          frame "U" {
          }
          frame "T" {
          }
          frame "S" {
          }
          frame "R" {
          }
          frame "Q" {
          }
          frame "P" {
          }
          frame "O" {
          }
          frame "N" {
          }
          frame "M" {
          }
          frame "L" {
          }
          frame "K" {
          }
          frame "J" {
          }
          frame "I" {
          }
          frame "H" {
          }
          frame "G" {
          }
          frame "F" {
          }
          frame "E" {
          }
          frame "D" {
          }
          frame "C" {
          }
          frame "B" {
          }
          frame "A" {
          }
          frame "9" {
          }
          frame "8" {
          }
          frame "7" {
          }
          frame "6" {
          }
          frame "5" {
          }
          frame "4" {
          }
          frame "3" {
          }
          frame "2" {
          }
          frame "1" {
          }
          frame "0" {
          }
        }
        n1841 = Bundle(w543, w542, w557, w556, 0.0) -> (w555:cluster{dbl, dbl, dbl, dbl, dbl})  [unwired: 1 in]
        n1842 = Bundle("X"=w565, "Y"=w564) -> (w559:cluster{"X":sgl, "Y":sgl})  [unwired: 1 in]
        n1843 = Divide(x=20, y=w526) -> (x/y=w529:sgl)
        n1844 = property on="Image Out" class="ImageControl"("Image Center Position"=w559) -> ()  [unwired: 2 in, 2 out]
        n1845 = call "IMAQ Convert Rectangle to ROI (Polygon)"("Rectangle"=w555) -> ("ROI Descriptor"=w553:T3)  [unwired: 7 in, 2 out]
        n1846 = Bundle("Application Font", w529, w533, w533, w533, w533, w533, TRUE, w531) -> (w535:T17)  [unwired: 1 in]
        n1847 = property on="Image Out 2" class="ImageControl"("ROI"=w553) -> ()  [unwired: 2 in, 2 out]
        n1848 = Bundle(w531, w535, w531, w531) -> (w534:T18)  [unwired: 1 in]
        n1849 = property on="Image Out" class="ImageControl"() -> ("ROI"=w518:T10)  [unwired: 2 in, 2 out]
        n1850 = Unbundle By Name(w518) -> ("Contours"=w582:T14)
        n1851 = local read "Image Out"() -> (w537:T2)
        n1852 = call "IMAQ Clear Overlay"("Image"=w537) -> ("Image Out"=w536:T2)  [unwired: 9 in, 1 out]
        n1853 = Initialize Array(0) -> (w580:i32[])  [unwired: 1 in]
        n1854 = local read "Magnification"() -> (w571:u16)
        n1855 = Array Size(array=w582) -> (size(s)=w581:i32)
        n1856 = Build Array(0.505025, 0.252522, 0.127742, 0.050345, 0.031129) -> (w572:dbl[])
        n1857 = Array Subset(array=w572, index=w571, length=1) -> (w569:dbl[])
        n1858 = property on="Image Out" class="ImageControl"() -> ("ZoomInteger"=w561:cluster{"X":i32, "Y":i32})  [unwired: 2 in, 2 out]
        n1859 = To Double Precision Float(number=w569) -> (double precision float=w568:dbl[])
        n1860 = for {
          N: w581 -> [_]
          shift-right: [w876] -> _
          shift-left: w582 -> [w876]
          shift-right: [w874] -> w567
          shift-left: w580 -> [w873]
          tunnel: w568 -> [w872]
          shift-right: [w869] -> _
          shift-left: w536 -> [w871]
          tunnel: w534 -> [w864]
          i -> [w868]
          n1861 = Index Array(array=w876, index=w868) -> (element=w885:T19)
          n1862 = Unbundle(w885) -> ("Points"=w884:i32[])  [unwired: 2 out]
          n1863 = Array To Cluster(array=w884) -> (cluster=w883:T20)
          n1864 = Unbundle(w883) -> ("Points[0]"=w863:i32, "Points[1]"=w860:i32, "Points[2]"=w875:i32, "Points[3]"=w881:i32)  [unwired: 5 out]
          n1865 = Add(x=w863, y=10) -> (x+y=w861:i32)
          n1866 = Subtract(x=w860, y=w881) -> (x-y=w880:i32)
          n1867 = Subtract(x=w863, y=w875) -> (x-y=w882:i32)
          n1868 = Square(x=w880) -> (x^2=w878:i32)
          n1869 = Square(x=w882) -> (x^2=w879:i32)
          n1870 = Add(x=w879, y=w878) -> (x+y=w877:i32)
          n1871 = Square Root(x=w877) -> (sqrt(x)=w854:dbl)
          n1872 = Multiply(x=w854, y=0.5) -> (x*y=w857:dbl)
          n1873 = Add(x=w857, y=w860) -> (x+y=w859:dbl)
          n1874 = Bundle(w861, w859) -> (w870:cluster{i32, dbl})  [unwired: 1 in]
          n1875 = Multiply(x=w854, y=w872) -> (x*y=w867:dbl[])
          n1876 = Index Array(array=w867) -> (element=w866:dbl)  [unwired: 1 in]
          n1877 = Number To Fractional String(number=w866) -> (F-format string=w865:string)  [unwired: 3 in]
          n1878 = call "IMAQ Overlay Text"("BG Color (Transparent)"=u32 0, "Text Color (black)"=u32 16448250, "Font, Size & Style"=w864, "String"=w865, "Origin"=w870, "Image"=w871) -> ("Image Out"=w869:T2)  [unwired: 4 in, 1 out]
          n1879 = Build Array (concatenate)(w873, w867) -> (w874:dbl[])
          n1880 = local write "Numeric 3"(w854) -> ()
        }
        n1881 = local write "ROI Descriptor"(w518) -> ()
        n1882 = Unbundle(w561) -> ("X"=w560:i32)  [unwired: 1 out]
        n1883 = Add Array Elements(numeric array=w567) -> (sum=w578:dbl)
        n1884 = local write "Distances"(w567) -> ()
        n1885 = local write "Total Width"(w578) -> ()
        n1886 = local write "Zoom"(w560) -> ()
        n1887 = local read "Manual-Width"() -> (w416:bool)
        n1888 = local read "Total Width"() -> (w521:dbl)
        n1889 = local read "Rec: Width"() -> (w519:dbl)
        n1890 = case shown="False" w416 {
          frame False {
            n1891 = property on="New: Width" class="DigNum (strict)"("DisabledEnum"=1) -> ()  [unwired: 2 in, 2 out]
          }
          frame True {
            n1892 = property on="New: Width" class="DigNum (strict)"("DisabledEnum"=0) -> ()  [unwired: 2 in, 2 out]
          }
        }
        n1893 = Not(x=w416) -> (.not. x?=w516:bool)
        n1894 = Equal To 0?(x=w521) -> (x = 0?=w517:bool)
        n1895 = Or(x=w517, y=w416) -> (x .or. y?=w520:bool)
        n1896 = And(x=w517, y=w516) -> (x .and. y?=w515:bool)
        n1897 = case shown="True" w515 {
          tunnel: w519 -> [_ w612]
          frame False {
          }
          frame True {
            n1898 = local write "New: Width"(w612) -> ()
          }
        }
        n1899 = case shown="False" w520 {
          tunnel: w521 -> [w614 _]
          frame False {
            n1900 = local write "New: Width"(w614) -> ()
            n1901 = property on="New: Width" class="DigNum (strict)"("DisabledEnum"=1) -> ()  [unwired: 2 in, 2 out]
          }
          frame True {
            n1902 = property on="New: Width" class="DigNum (strict)"("DisabledEnum"=0) -> ()  [unwired: 2 in, 2 out]
          }
        }
        n1903 = local read "Manual Comments"() -> (w417:bool)
        n1904 = local read "Rec: Comments"() -> (w418:string)
        n1905 = local read "Manuel-Dielectric"() -> (w444:bool)
        n1906 = local read "Rec: Dielectric (d)"() -> (w443:dbl)
        n1907 = local read "Manuel-Length"() -> (w445:bool)
        n1908 = local read "Rec: Length"() -> (w446:dbl)
        n1909 = case shown="True" w417 {
          tunnel: w418 -> [w587 _]
          frame False {
            n1910 = local write "Comments:"(w587) -> ()
            n1911 = property on="Comments:" class="Str"("DisabledEnum"=1) -> ()  [unwired: 2 in, 2 out]
          }
          frame True {
            n1912 = property on="Comments:" class="Str"("DisabledEnum"=0) -> ()  [unwired: 2 in, 2 out]
          }
        }
        n1913 = case shown="True" w445 {
          tunnel: w446 -> [w602 _]
          frame False {
            n1914 = local write "New: Length"(w602) -> ()
            n1915 = property on="New: Length" class="DigNum (strict)"("DisabledEnum"=1) -> ()  [unwired: 2 in, 2 out]
          }
          frame True {
            n1916 = property on="New: Length" class="DigNum (strict)"("DisabledEnum"=0) -> ()  [unwired: 2 in, 2 out]
          }
        }
        n1917 = case shown="True" w444 {
          tunnel: w443 -> [w599 _]
          frame False {
            n1918 = local write "New: Dielectric"(w599) -> ()
            n1919 = property on="New: Dielectric" class="DigNum (strict)"("DisabledEnum"=1) -> ()  [unwired: 2 in, 2 out]
          }
          frame True {
            n1920 = property on="New: Dielectric" class="DigNum (strict)"("DisabledEnum"=0) -> ()  [unwired: 2 in, 2 out]
          }
        }
      }
    }
  }
  n1921 = Build Array("DeviceID", "Fabricator", "Deposition", "Date", "Sample", "Row", "Column", "L (um)", "W (um)", "Material", "Treatment", "TC (mM)", "Solvent", "C (%)", "ST (C)", "Drops", "Wait (s)", "RT (F)", "RH (%)", "Ramp (s)", "RPM", "Accel (RPM/s)", "Time (s)", "Mobility", "On/Off", "Vt", "S.T.S") -> (→"Transformer \nHeaders":string[])
